vi "MANIPULATOR.vi"() -> ()   [LabVIEW 2018]
uses:
  MCode_LV_86/Set Parameter.ctl
  subVIs/Units_of_Move.ctl
  subVIs/Define_Position.ctl
  subVIs/KE_Scan_XY-Graph.ctl
  Keithley Picoammeter/subVIs/Current_Range_Control.ctl
  subVIs/Scan Mode.ctl
  Surveillance/limit_switch_Cluster.ctl
  ConversionAndInformation/Unit_Control.ctl
  <vilib>/DAQmx/read.llb/DAQmx Read (Analog 1D DBL 1Chan NSamp).vi
  subVIs/Save_Time_Global.vi
  Surveillance/Pressure_Ch_1_2_Manipulator_Pos.vi
  <vilib>/DAQmx/create/channels.llb/DAQmx Create Channel (AI-Voltage-Basic).vi
  <vilib>/DAQmx/configure/timing.llb/DAQmx Timing (Sample Clock).vi
  <vilib>/DAQmx/miscellaneous.llb/DAQmx Fill In Error Info.vi
  subVIs/Global_Next_Scan_Position.vi
  subVIs/Global_external_move_cmd.vi
  Surveillance/Switch _Laser_Global.vi
  <vilib>/Utility/file.llb/Write To Spreadsheet File (DBL).vi
  subVIs/Global_Stop_Scan.vi
panel:
  out "Current Scan Step":i32
  out "Number of Scan Steps":i32
  in  "Next Scan Step":bool
  out "Sample Scan Array Out":i32[][](array[numeric])
  in  "Last Scan Step?":bool
  out "velocity cluster":T1
  out "limit switch cluster":T2
  out "Motor 6":u16
  out "At Next Pos?":bool caption="At Next Position?"
  out "At first Scan Pos?":bool
  out "waypoint info pic":picture
  in  "Disp Axis Info":bool
  out "axis info pic":picture
  in  "Current\nRange Ch2":T3 items=["Autorange", "+/- 20 mikroA", "+/- 2 mikroA", "+/- 200 nA", "+/- 20 nA", "+/- 2 nA"]
  in  "Current\nRange Ch1":T3 items=["Autorange", "+/- 20 mikroA", "+/- 2 mikroA", "+/- 200 nA", "+/- 20 nA", "+/- 2 nA"]
  in  "GPIB (t) / RS-232 (f)":bool=TRUE
  in  "DAQ Dev":refnum<visa-resource-name>="GPIB0::25::INSTR"
  out "Status":i32 format="%.0b"
  out "use data":bool
  out "buffer":string
  in  "Cluster":T4={"Baudrate (57600)"=57600, "Data Bits (8)"=8, "Parity (None)"=0, "Stop Bits (1)"=10, "Flow Control (None)"=0, "End Mode Read (TermChar)"=2} {"End Mode Read (TermChar)" items=["None", "Last Bit", "TermChar"]; "Flow Control (None)" items=["None", "XON/XOFF", "RTS/CTS", "XON/XOFF & RTS/CTS", "DTR/DSR", "XON/XOFF & DTR/DSR"]; "Stop Bits (1)" items=["1.0"=10, "1.5"=15, "2.0"=20]; "Parity (None)" items=["None", "Odd", "Even", "Mark", "Space"]; "Baudrate (57600)" items=["300"=300, "600"=600, "1200"=1200, "2400"=2400, "4800"=4800, "9600"=9600, "19200"=19200, "38400"=38400, "57600"=57600, "115200"=115200]}
  in  "Notizen":string="Limit switch rotation at +225 degrees\n                                          -135 degrees\nSample 1\nSample 2\nSample 3\nSample 4 rutile single crystal (left edge, middle)"
  out "Loaded Positions":string
  in  "Load Motor Positions":bool
  in  "Define New\nPos Dummy":bool
  in  "Set x,y,z Zero Dummy":bool
  in  "Set Angle Zero Dummy":bool
  in  "Stop w Save Pos":bool
  out "MM?":bool
  in  "emergency stop":bool
  in  "stop":bool
  in  "Tab Control":T5(tab)
  in  "ComPort Manipulator":refnum<visa-resource-name>="COM5"
  out "error out":errorcluster={"status"=FALSE, "code"=1073676294, "source"="VISA Read in write_read.vi"}
  out "ComPort out":refnum<visa-resource-name>
  in  "Answer":string
  in  "Send Cmd":bool
  in  "Value":string
  in  "Reset Error":bool
  in  "Command":T6
  in  "Send Cmd as is":bool
  in  "Send As Is String":string
  in  "Motor":u16(ring) items=["none", "1", "2", "3", "4", "all"]
  in  "Print":bool
  in  "Print Error":bool
  out "Transmitted String":string
  in  "Clear Answer":bool
  out "Firmware Version":string
  out "Stop Scan GLOBAL":bool
  out "scan info pic":picture
  in  "ext. Cmd":bool
  out "Scan\nProb?":bool
  in  "POV Map":bool
  out "Next Pos":i32[](array[numeric])
  in  "Disp Path":bool=TRUE
  in  "refresh (s)":dbl=2.0
  in  "Reset Map":bool
  out "Pos Graph":cluster{dbl[], dbl[]}[](graph)
  out "Paused?":bool
  in  "Disp Waypoint Info":bool
  out "Pico Error":bool
  in  "Z tilt (x/z)":dbl=0.00339817
  in  "pause scan":bool
  in  "Scan Type":bool
  in  "Scan Mode":T7 caption="Scan Settings" items=["Mode 1", "Mode 2", "Reversed 1", "Reversed 2"]
  in  "Disp Scan Info":bool
  in  "Stop Scan (2D)":bool
  in  "Speed [microns/s]":dbl=100.0 min=0.0 max=1500.0
  in  "Sample\nScan":bool
  in  "Channel IN":tag
  out "Mean":dbl caption="Analog IN (V)" format="%_3e"
  in  "V_min":dbl=-10.0
  in  "V_max":dbl=10.0
  in  "Stop NI":bool
  in  "Start NI":bool
  out "Display Saved Pos String":string
  in  "Display Saved Position":bool
  in  "WAYPOINTS":u16(ring) items=["Current Position", "Diode Bottom", "Diode Middle Small", "Diode Middle Large", "Diode Top", "Phosphor", "Sample 1", "Sample 2", "Sample 3", "Sample 4", "Horizontal Motor Scan", "Vertical Motor Scan", "Corner Left Top", "Corner Bottom Right"]
  in  "Go to Saved Position":bool
  in  "Motor 4":dbl
  in  "Motor 3":dbl
  in  "Motor 2":dbl
  in  "Motor 1":dbl
  in  "Def Speed":bool
  in  "Unit of Move":T8=1 items=["STEPS", "MICRONS / DEG", "MILLIMETER / DEG", "CENTIMETER / DEG", "INCHES / DEG"]
  in  "move in plain 2":bool caption="M1 + / M2 -"
  in  "move in plain 1":bool caption="M1 - / M2 +"
  in  "move away detector":bool caption="M1 +"
  in  "move to detector":bool caption="M1 -"
  in  "move clockwise":bool caption="M4 -"
  in  "move counterclockwise":bool caption="M4 +"
  in  "move away x-rays":bool caption="M2 +"
  in  "move to x-rays":bool caption="M2 -"
  out "Saved Positions":string
  in  "Save Motor Positions":bool
  in  "Set Angle Zero":bool
  in  "Set x,y,z Zero":bool
  in  "move down":bool caption="M3 +"
  in  "move up":bool caption="M3 -"
  in  "Rel Steps":string="1"
  in  "Speed":dbl=250.0 caption="(microns/s)/\n(degrees/s)" min=0.0 max=2000.0
  in  "Pos 1 (Steps)":i32 caption="Position 1 (Steps)"
  in  "Pos 2 (Steps)":i32 caption="Position 2 (Steps)"
  in  "Pos 3 (Steps)":i32 caption="Position 3 (Steps)"
  in  "Pos 4 (Steps)":i32 caption="Position 4 (Steps)"
  in  "Pos 1":dbl caption="Position 1" step=1.0 format="%_6g"
  in  "Pos 2":dbl caption="Position 2" step=1.0 format="%_6g"
  in  "Pos 3":dbl caption="Position 3" step=1.0 format="%_6g"
  in  "Pos 4 [Angle]":dbl caption="Position 4 [Angle]" step=0.1 format="%_6g"
  in  "Get Motor Positions":bool
  in  "Pos Unit":T8=1 items=["STEPS", "MICRONS / DEG", "MILLIMETER / DEG", "CENTIMETER / DEG", "INCHES / DEG"]
  in  "Z tilt (degrees)":dbl=-0.1947 caption="(degrees)"
  in  "Z tilt comp":bool
  in  "Motor2-xRays (degrees)":dbl
  in  "Unit of Move 3":T8=1 items=["STEPS", "MICRONS / DEG", "MILLIMETER / DEG", "CENTIMETER / DEG", "INCHES / DEG"]
  in  "M1 Change":T9
  in  "M2 Change":T9
  in  "M3 Change":T9
  in  "M4 Change":T9
  in  "Define New Pos":bool caption="DEFINE CURRENT POSITION"
  out "Data":dbl[](array[numeric]) caption="Channel 1 (A)\n\nChannel 2 (A)" format="%#_3e"
  in  "Stop K":bool
  in  "Calc Scan Time":bool
  out "Scan Time":string
  in  "Start K":bool
  in  "Line Spacing [microns]":dbl=500.0
  in  "Pico Steps":i32 caption="Steps"
  in  "PicoMotor":u16(ring) caption="Motor" items=["A", "B", "C"]
  in  "Move Pico":bool
  in  "Picomotors Port":refnum<visa-resource-name>="COM1"
  in  "GaussFit der (f, def) / raw (t)":bool caption="GaussFit\nder (f)\nraw (t)"
  in  "div I zero":bool=TRUE caption="divide by other K Ch"
  in  "Interrupt 2":bool
  in  "Interrupt 1":bool
  in  "Go to Cursor (1 Motor)":bool
  in  "Knife Edge Scan\n(1 Motor)":bool
  in  "Scan Range":dbl=100.0
  in  "Axis":u16(ring) items=["Detector", "X-Rays", "Vertical", "In-Plain", "Vertical (with tilt)"]
  in  "Nr. of Steps":u32=10
  in  "Integration Time per Step":u32=1500
  in  "Channel":i32=1 min=0 max=7 step=1
  in  "Go to Cursor (2 Motors)":bool
  in  "Knife Edge Scan\n(2 Motors)":bool
  out "XY Graph":T10
  out "FWHM":dbl format="%.1f"
  out "Center":dbl format="%.1f"
  out "Resolution":dbl
  out "Start\nTime":timestamp
  out "Estimated\nStop Time":timestamp
  out "Scan Number":i32
  out "Residue":dbl
  in  "NI DAQ (t) / Keithley (f)":bool
  out "current time":string
  out "end time":string
  in  "Switch Laser":bool
  in  "XPS Scan Speed [µm/s]":dbl=100.0 caption="Scan Speed [µm/s]" min=0.0 max=1500.0
  in  "Z tilt comp XPS":bool
  in  "Z tilt (M2/M3) XPS":dbl=0.00202
  in  "scan up M3- XPS":bool
  in  "scan down M3+ XPS":bool
  in  "Scan Distance XPS":string="5" caption="Scan Distance (mm)"
  in  "stop scan XPS":bool
  in  "scan left XPS":bool
  in  "scan right XPS":bool
  in  "Hor Angle Offset (degrees)":dbl
  in  "Hor Angle Offset (rad) M2/M1":dbl
  out "M4 XPS":dbl caption="M4 Angle (degrees)" step=10.0 format="%_6g"
  out "M3 XPS":dbl caption="M3 Vertical (micrometer)" step=1.0 format="%_6g"
  out "M2 XPS":dbl caption="M2 Analyzer (micrometer)" step=1.0 format="%_6g"
  out "M1 XPS":dbl caption="M1 X-rays (micrometer)" step=1.0 format="%_6g"
  in  "Rel Steps XPS":string="1000" caption="Micrometer µm"
  in  "approach XPS":bool caption="M 2 - / M 1 -"
  in  "retract XPS":bool caption="M 2 + / M 1 +"
  in  "in plain 2 XPS":bool caption="M 2 - / M 1 +"
  in  "in plain 1 XPS":bool caption="M 2 + / M 1 -"
  in  "away X-rays M1+ XPS":bool caption="M 1 +"
  in  "to X-rays M1- XPS":bool caption="M 1 -"
  in  "move clockwise XPS":bool caption="M 4 -"
  in  "move counterclockwise XPS":bool caption="M 4 +"
  in  "away analyzer M2+ XPS":bool caption="M 2 +"
  in  "to analyzer M2- XPS":bool caption="M 2 -"
  in  "down M3+ XPS":bool caption="M 3 +"
  in  "up M3- XPS":bool caption="M 3 -"
  in  "Rel Deg XPS":string="1" caption="Degrees"
  out "Pos Graph 2":cluster{dbl[], dbl[]}[](graph)
  in  "down M3+ TEST":bool
  in  "up M3- TEST":bool
  out "actual angle":dbl format="%_6g"
  out "V_max Motor 2":i32
  out "V_max Motor 1":i32
  out "steps motor 2 ()":string
  out "steps motor 1 ()":string
  in  "Idiotensicherung":bool
  out "delta time (ms)":i32
  in  "steps 2":i32
  in  "Loop Stop":bool
  in  "Motor 5":u16(ring) items=["none", "1", "2", "3", "4", "all"]
  in  "Move Time Test":bool
  in  "motor stopped":bool
  out "1":u32
  out "2":u32
  out "single steps 1":i32[](array[numeric])
  out "single steps 2":i32[](array[numeric])
  out "move time (ms)":u32
  out "single steps":i32[](array[numeric])
  out "New X-Ray Pos":i32
  out "Percentage Range Micron Pos":dbl
  out "Range X-Rays":i32
  out "Range M1/M3":i32
  out "Min Value X-Rays":i32
  in  "direction":bool
  in  "In-Plain subVI Test":bool
  in  "Speed [micron/s] 2":dbl=750.0 min=0.0
  in  "Steps":dbl format="%#_13g"
  in  "Unit of Move 2":T8 items=["STEPS", "MICRONS / DEG", "CENTIMETER / DEG", "INCHES / DEG"]
  out "move time (ms) 4":u32
  out "actual angle 2":dbl format="%_6g"
  out "angle":dbl
  out "Array Lengths equal?":bool
  out "V_max 1/3 and 2":i32[](array[numeric])
  out "micron steps":dbl[](array[numeric])
  out "New M1/M3 Pos":i32
  out "KE Scan Array":dbl[][](array[numeric])
  out "Transmitted 1/3":string
  out "Transmitted 2":string
  in  "Save latest KE Scan":bool
  out "error Keithley":errorcluster
  out "error NI":errorcluster
  out "corner 1":dbl[](array[numeric])
  out "corner 2":dbl[](array[numeric])
  in  "Reset V_max":bool
  in  "Save Files Array":path[](array[path])
  out "KE Positions":dbl[](array[numeric]) caption="(micron/degree)"
  out "Transmitted String Baud Rate":string
  in  "Baudrate":u32(ring)=9600 items=["9600"=9600, "19200"=19200, "38400"=38400, "115200"=115200]
  in  "Change Baud Rate":bool
  # "LIMIT\nSWITCH"
  # "KEITHLEY SETTINGS"
  # "angle element -90 to 90 deg:\n[sample holder facing xrays]\nIn plain 1 -> towards detector\nIn plain 2 -> away from det.\nangle <-90 or >90 deg:\n[back of sample holder facing xrays]\nIn plain 1 -> away from det.\nIn plain 2 -> towards detector"
  # "RELATIVE MOVEMENT"
  # "ABSOLUTE MOVEMENT"
  # "motor 1: detector axis [+ away / - towards detector]"
  # "motor 2: x-ray axis [+ away / - towards x-rays]"
  # "motor 3: vertical axis [+ down / - up]"
  # "motor 4: angle [+ counterclockwise / - clockwise]"
  # "TILT COMPENSATION"
  # "WAYPOINTS"
  # "NOT functional"
  # "Sample holder facing x-rays. Alpha is the angle between\nmanipulator z-axis and x-rays incident on the sample holder.\n\"Z tilt\" is > 0 if alpha >90 degreees (\"Z tilt\"<0 -> alpha < 90)."
  # "KEITHLEY PICCOAMMETER"
  # "NI USB DAQ BOARD"
  # "SAMPLE SCAN"
  # "NEWFOCUS PICOMOTORS"
  # "DAQ Source"
  # "Range: +/-"
  # "microns around current position"
  # "+1 | Integration time per step:"
  # "Steps: 2x"
  # "ms"
  # "Axis:"
  # "| Sampling:"
  # "microns"
  # "FINE POSITIONING"
  # "SCANNING SAMPLE"
  # "Replace In-Plain\nCode with real\ntrigonometric\nfunctions!"
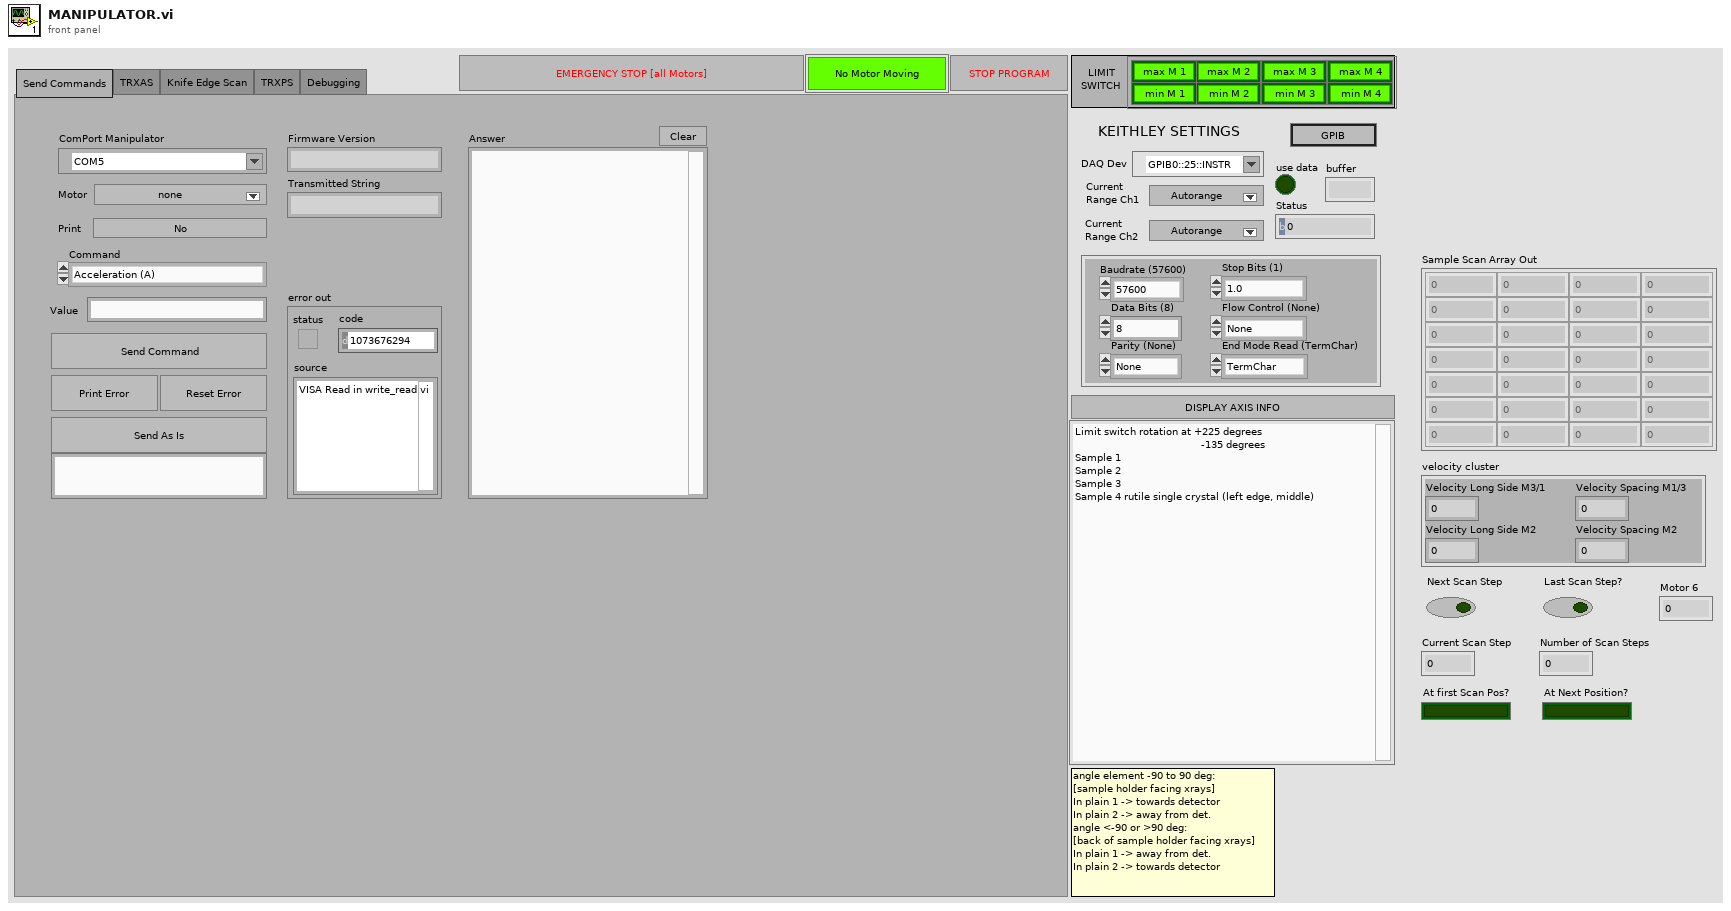
[diagram p1: front panel]
types:
  T1 = cluster{"Velocity Long Side M3/1":dbl, "Velocity Long Side M2":dbl, "Velocity Spacing M1/3":dbl, "Velocity Spacing M2":dbl}
  T2 = typedef "limit_switch_Cluster.ctl" = cluster{"Limit Switch max M 1":bool, "Limit Switch min M 1":bool, "Limit Switch max M 2":bool, "Limit Switch min M 2":bool, "Limit Switch max M 3":bool, "Limit Switch min M 3":bool, "Limit Switch max M 4":bool, "Limit Switch min M 4":bool}
  T3 = typedef "Current_Range_Control.ctl" = u16
  T4 = cluster{"Baudrate (57600)":u32, "Data Bits (8)":u16, "Parity (None)":u16, "Stop Bits (1)":u16, "Flow Control (None)":u16, "End Mode Read (TermChar)":u16}
  T5 = enum32{"Send Commands", "TRXAS", "Knife Edge Scan", "TRXPS", "Debugging"}
  T6 = typedef "Set Parameter.ctl" = enum16{"Acceleration (A)", "Baud Rate (BD)", "Counter 1 (C1)", "Counter 2 (C2)", "Control C Software Reset (CE)", "Check Sum Enable (CK)", "Clock Mode (CM)", "Clock Mode Ratio (CR)", "Clock Mode Out Step Width (CW)", "Deceleration (D)", "Digital Filtering, Input 1 (D1)", "Digital Filtering, Input 2 (D2)", "Digital Filtering, Input 3 (D3)", "Digital Filtering, Input 4 (D4)", "Digital Filtering, Input 5 (D5)", "Digital Filtering, Input 9 (D9)", "Digital Filtering, Input 10 (D10)", "Digital Filtering, Input 11 (D11)", "Digital Filtering, Input 12 (D12)", "Deadband (DB)", "Decrement Variable (DC)", "Enable/Disable Drive (DE)", "Device Name (DN)", "End Program Execution (E)", "Encoder Function Enable (EE)", "Error Flag (EF)", "Encoder Lines (EL)", "Echo Mode (EM)", "Error Value (ER)", "Escape (ES)", "Execute Program at Address (EX)", "Firmware Version (VR)", "Hold (H)", "Hold Current (HC)", "Hold Current Delay Time (HI)", "Home to Encoder Index (HM)", "Home to Home Switch (HT)", "Increment Variable (IC)", "Initialize Parameters to NVM (IP)", "Input into Variable (IV)", "Jog Enable (JE)", "Limit Stop Mode (LM)", "Move Absolute (MA)", "Move Relative (MR)", "MicroStepping Select (MS)", "Motor Settling Delay Time (MT)", "Moving [Flag] (MV)", "Output 1 (O1)", "Output 2 (O2)", "Output 3 (O3)", "Output 4 (O4)", "Output 9 (O9)", "Output 10 (O10)", "Output 11 (O11)", "Output 12 (O12)", "Output High Byte (9-12) (OH)", "Output Low Byte (1-4) (OL)", "Output Total (1-4 and 9-12) (OT)", "Position (P)", "Position Maintenance (PM)", "Party Mode (PY)", "Register 1 (R1)", "Register 2 (R2)", "Register 3 (R3)", "Register 4 (R4)", "Reset Error(\\03)", "Run Current (RC)", "Stall Factor (SF)", "Slew (SL)", "Stall Mode Set (SM)", "Upgrade Firmware (UG)", "Velocity Initial (VI)", "Velocity Maximum (VM)", "Current1 (I1)", "Current2 (I2)", "Current3 (I3)", "Current4 (I4)", "Current5 (I5)", "Current6 (I6)", "Save (S)"}
  T7 = typedef "Scan Mode.ctl" = u16
  T8 = typedef "Units_of_Move.ctl" = u16
  T9 = typedef "Define_Position.ctl" = bool
  T10 = typedef "KE_Scan_XY-Graph.ctl" = cluster{dbl[], "subarray":dbl[]}[]
  T11 = typedef "Unit_Control.ctl" = enum16{"Angle (Degrees)", "Rad", "Angle [TMC]", "Microsteps [TMC]", "Inches", "Nanometer", "Meter", "Centimeter", "Millimeter", "Micron"}
  T12 = cluster{"Baudrate (115200)":u32, "Data Bits (8)":u16, "Parity (None)":u16, "Stop Bits (1)":u16, "Flow Control (None)":u16, "End Mode for Reads (TermChar)":u16}
  T13 = enum16{"open", "replace", "create", "open or create", "replace or create", "replace or create with confirmation"}
  T14 = typedef "imagedata.ctl" = cluster{"image type":i32, "image depth":i32, "image":u8[], "mask":u8[], "colors":u32[], "Rectangle":cluster{"left":i16, "top":i16, "right":i16, "bottom":i16}}
  T15 = typedef "Semaphore RefNum" = refnum<k1>
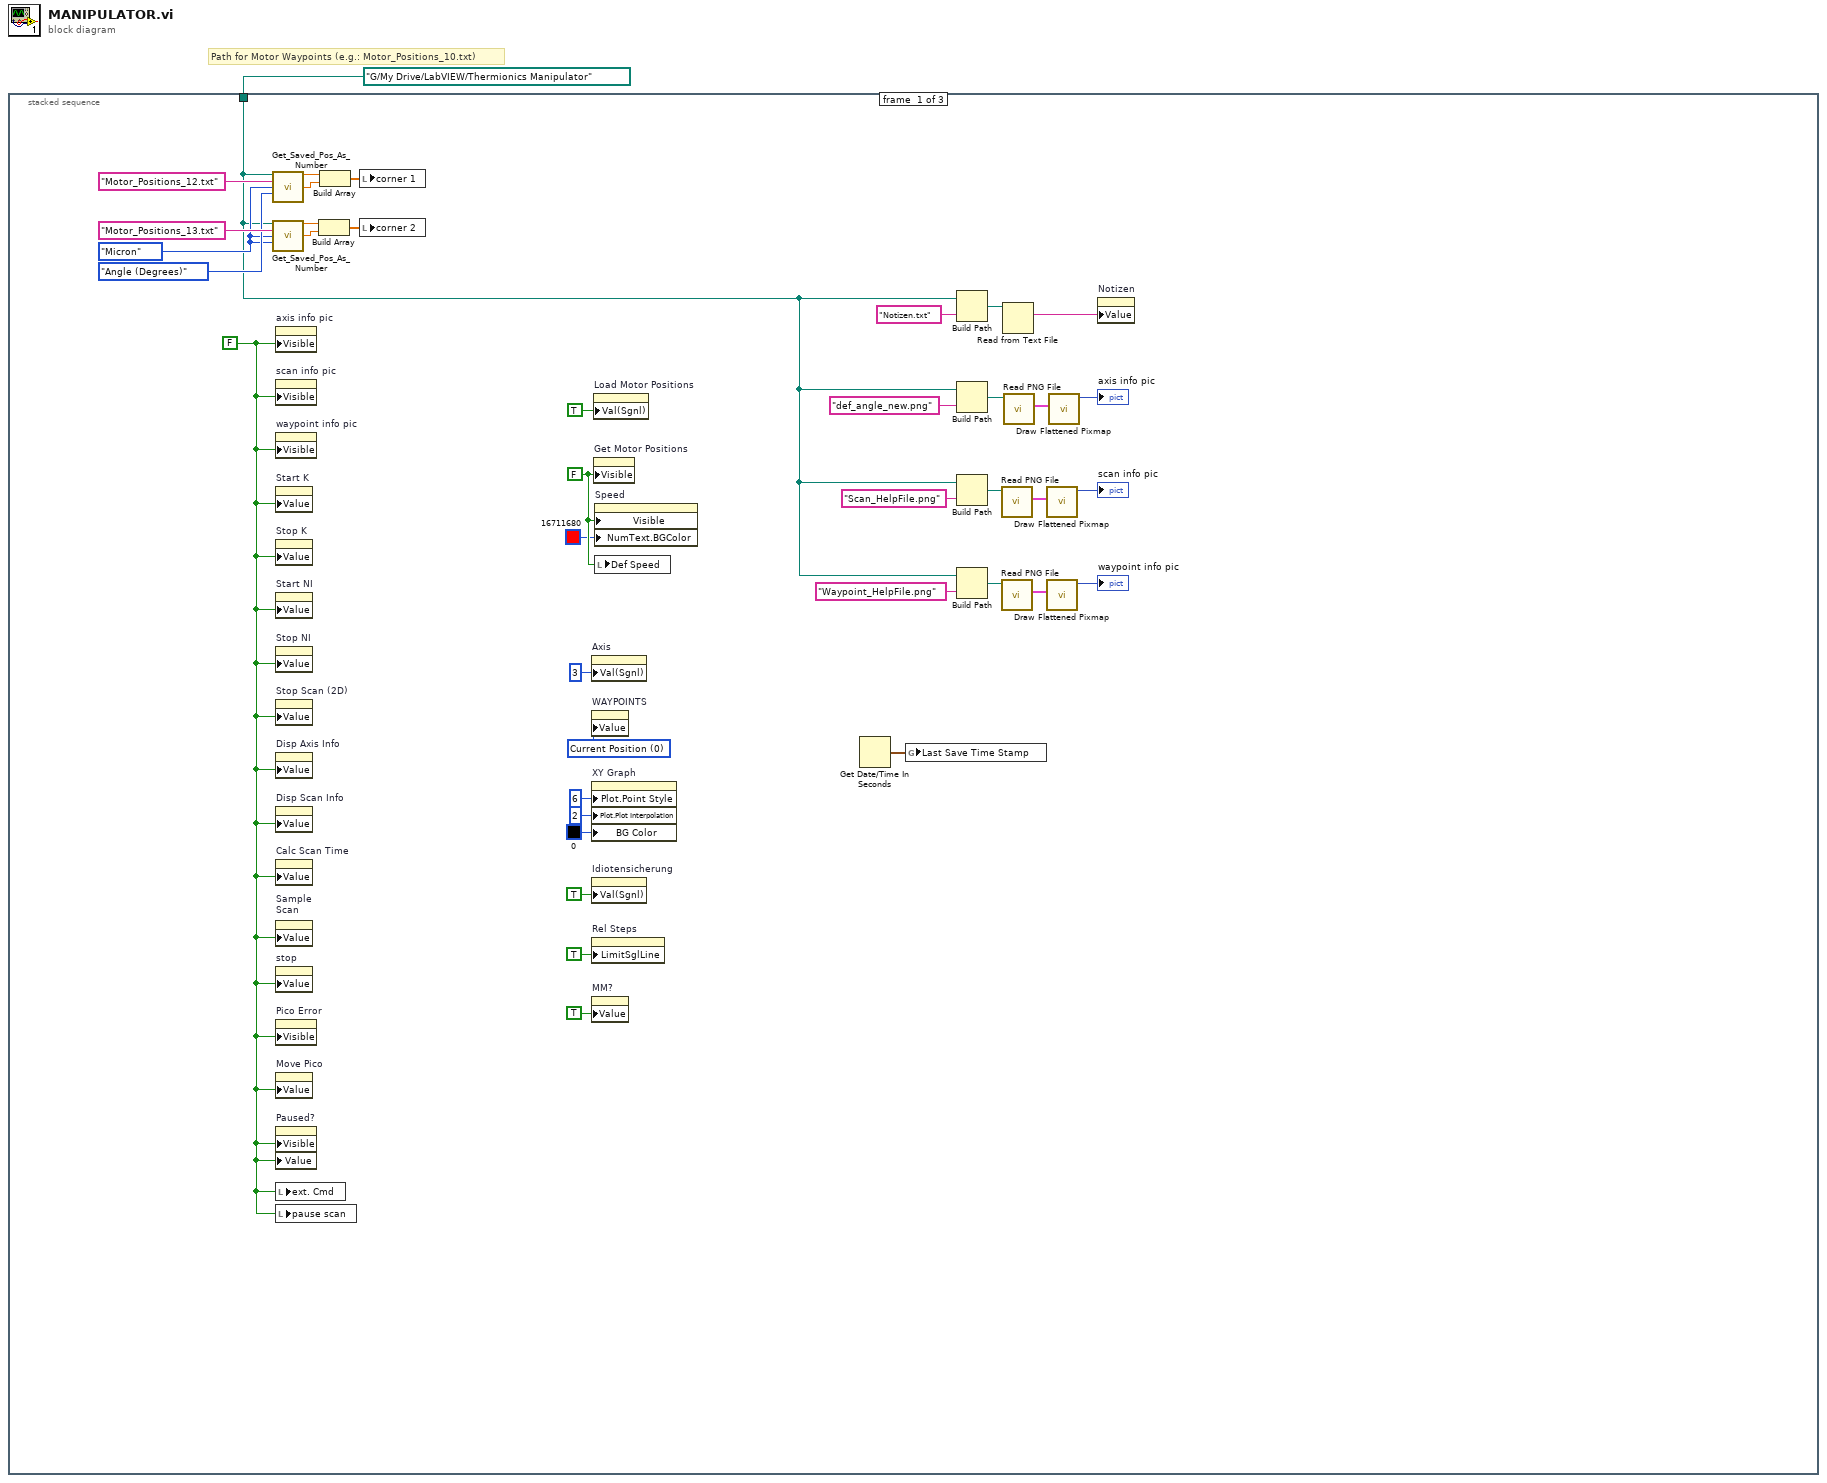
[diagram p0: block diagram]
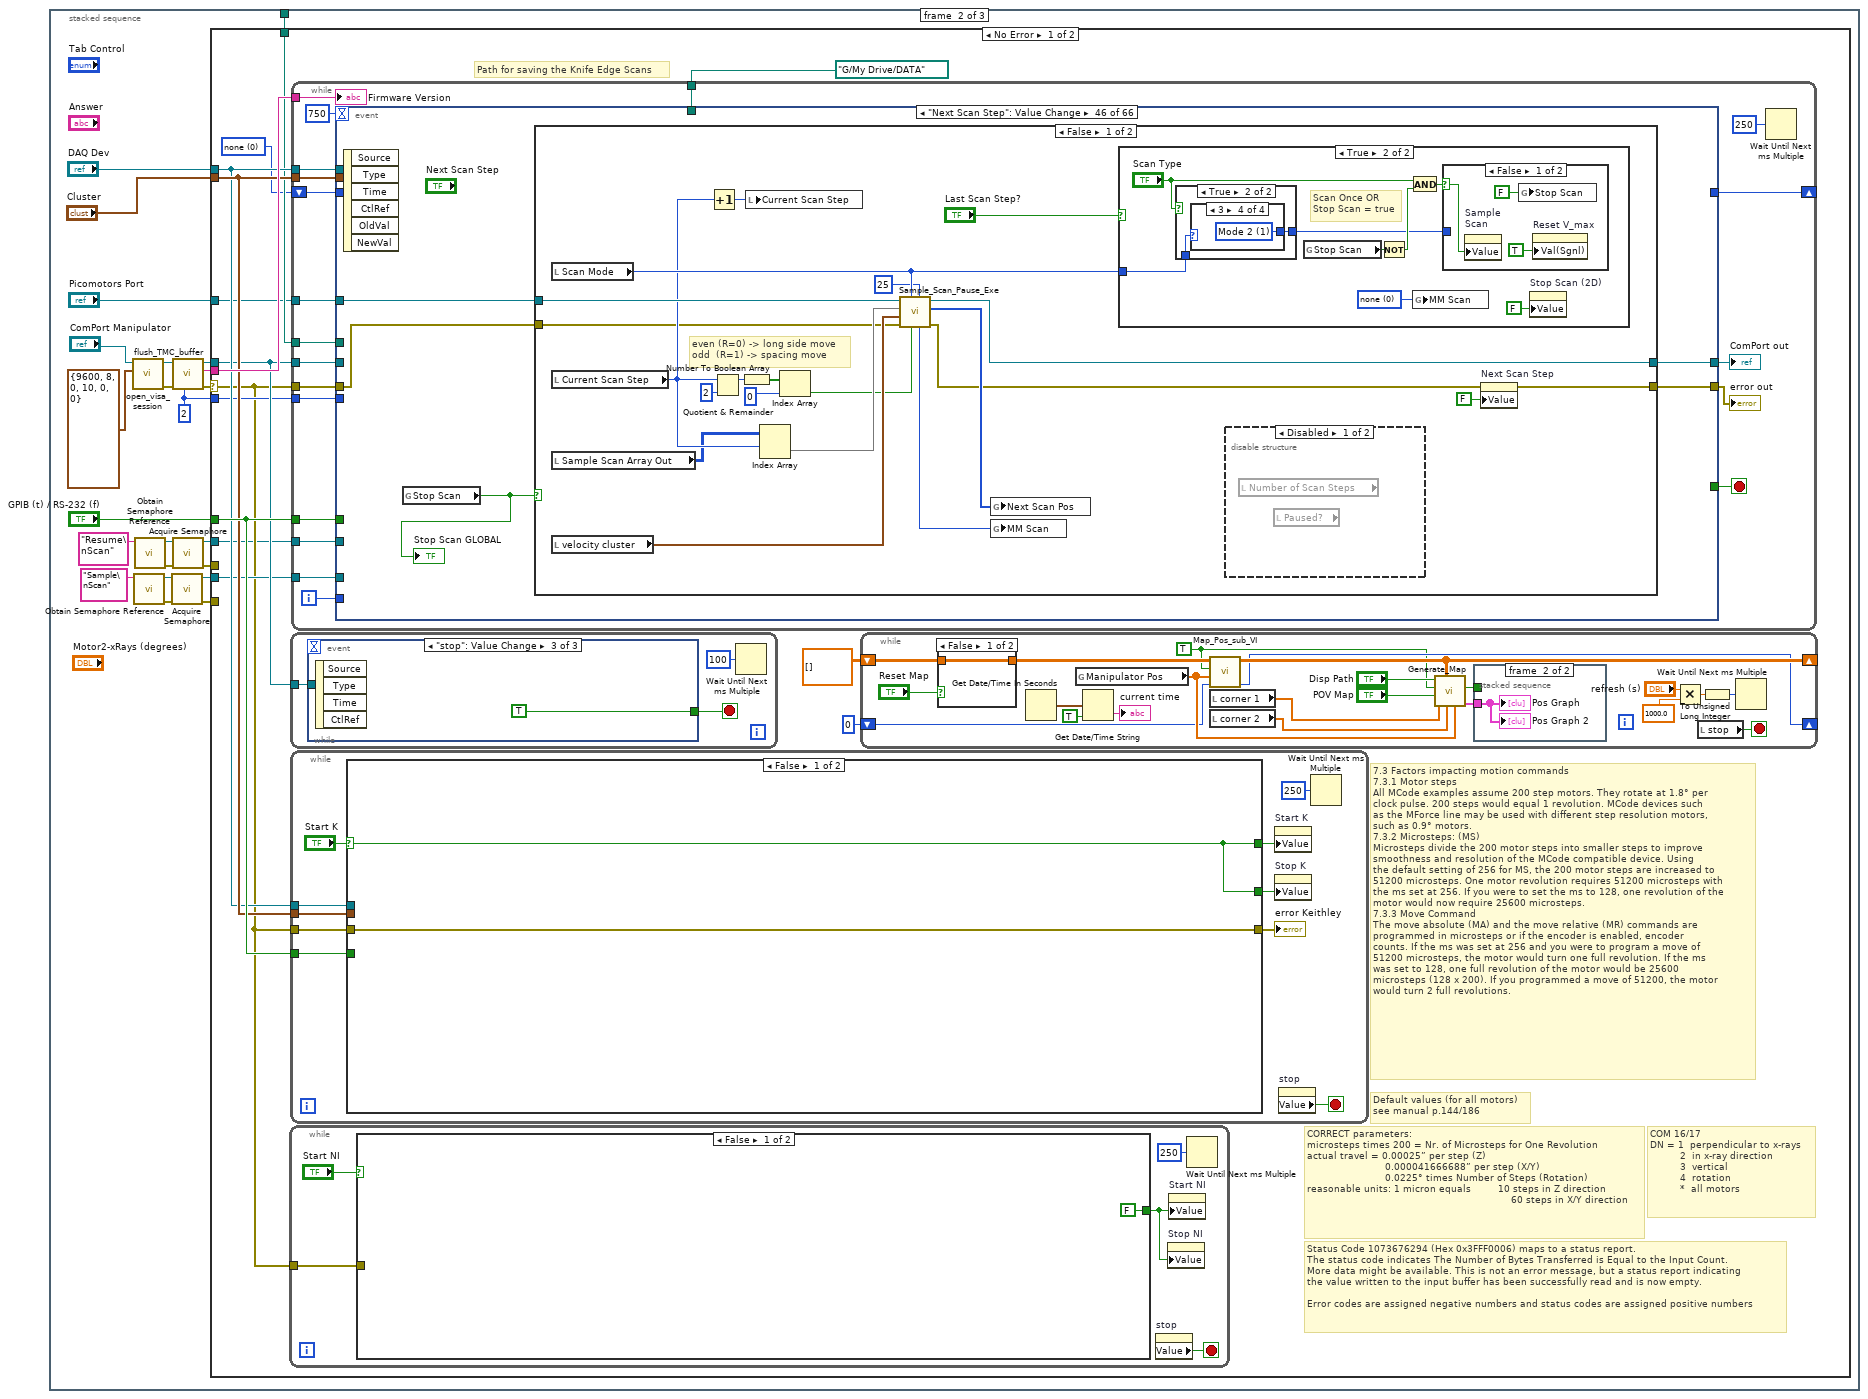
[diagram p2: hidden frame]
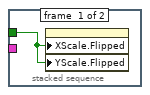
[diagram p3: hidden frame]
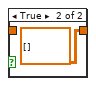
[diagram p4: hidden frame]
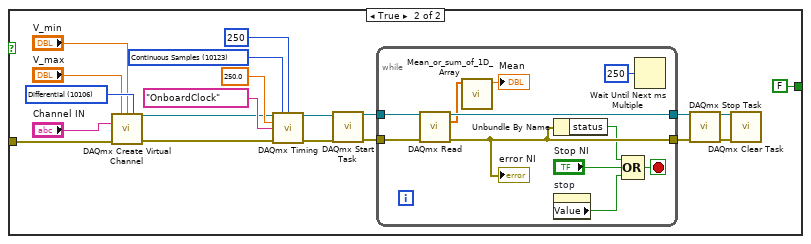
[diagram p5: hidden frame]
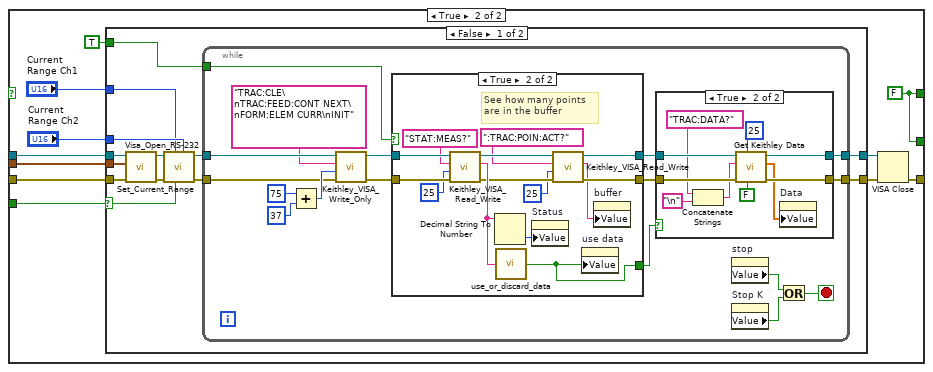
[diagram p6: hidden frame]
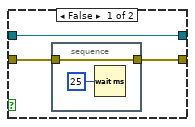
[diagram p7: hidden frame]
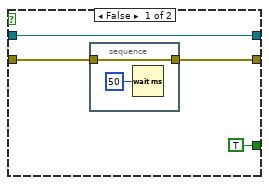
[diagram p8: hidden frame]
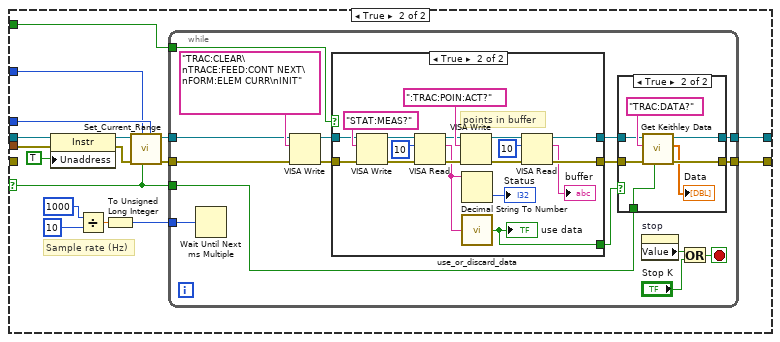
[diagram p9: hidden frame]
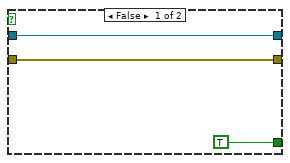
[diagram p11: hidden frame]
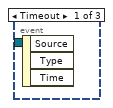
[diagram p12: hidden frame]
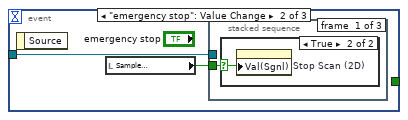
[diagram p13: hidden frame]
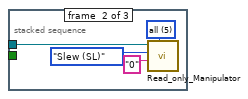
[diagram p15: hidden frame]
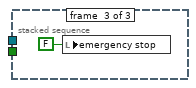
[diagram p16: hidden frame]
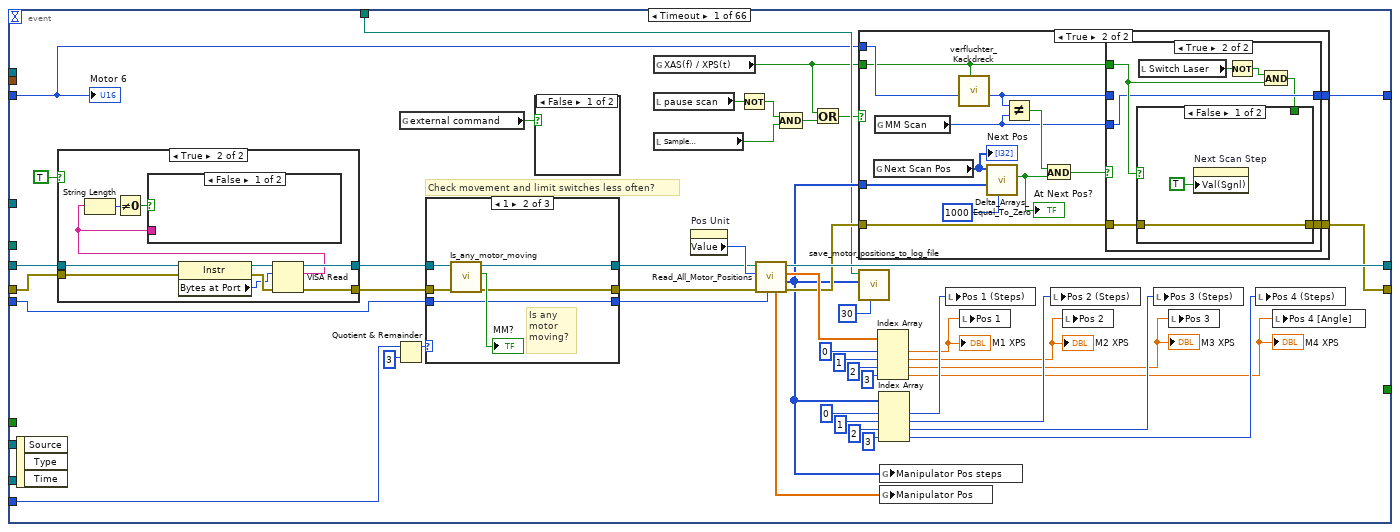
[diagram p17: hidden frame]
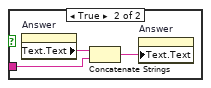
[diagram p19: hidden frame]
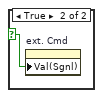
[diagram p20: hidden frame]
diagram:
  # "Path for Motor Waypoints (e.g.: Motor_Positions_10.txt)"
  n1 = stacked-sequence {
    tunnel: path "G:/My Drive/LabVIEW/Thermionics Manipulator" ("file path (use dialog)") -> [w5 w48 _]
    frame #0 {
      w18 = Unit_Control."Micron" ("Outuput Unit 1/2/3")
      w27 = u16 0 items=["Current Position", "Diode Bottom", "Diode Middle Small", "Diode Middle Large", "Diode Top", "Phosphor", "Sample 1", "Sample 2", "Sample 3", "Sample 4"] ("WAYPOINTS")
      w25 = FALSE ("Visible")
      w9 = FALSE ("Visible")
      n2 = call "Get_Saved_Pos_As_Number.vi"("file path"=w5, "file name"="Motor_Positions_12.txt" ("name or relative path"), "Outuput Unit 1/2/3"=w18, "Outuput Unit 4"=Unit_Control."Angle (Degrees)" ("Outuput Unit 1/2/3")) -> ("Pos 1"=w17:dbl, "Pos 3"=w16:dbl)  [unwired: 7 in, 3 out]
      n3 = call "Get_Saved_Pos_As_Number.vi"("file path"=w5, "file name"="Motor_Positions_13.txt" ("name or relative path"), "Outuput Unit 1/2/3"=w18, "Outuput Unit 4"=w18) -> ("Pos 1"=w15:dbl, "Pos 3"=w14:dbl)  [unwired: 7 in, 3 out]
      n4 = property on="axis info pic" class="Pict"("Visible"=w9) -> ()  [unwired: 2 in, 2 out]
      n5 = property on="scan info pic" class="Pict"("Visible"=w9) -> ()  [unwired: 2 in, 2 out]
      n6 = property on="waypoint info pic" class="Pict"("Visible"=w9) -> ()  [unwired: 2 in, 2 out]
      n7 = property on="Start K" class="Bool (strict)"("Value"=w9) -> ()  [unwired: 2 in, 2 out]
      n8 = property on="Stop K" class="Bool (strict)"("Value"=w9) -> ()  [unwired: 2 in, 2 out]
      n9 = property on="Start NI" class="Bool (strict)"("Value"=w9) -> ()  [unwired: 2 in, 2 out]
      n10 = property on="Stop NI" class="Bool (strict)"("Value"=w9) -> ()  [unwired: 2 in, 2 out]
      n11 = property on="Stop Scan (2D)" class="Bool (strict)"("Value"=w9) -> ()  [unwired: 2 in, 2 out]
      n12 = property on="Disp Axis Info" class="Bool (strict)"("Value"=w9) -> ()  [unwired: 2 in, 2 out]
      n13 = property on="Disp Scan Info" class="Bool (strict)"("Value"=w9) -> ()  [unwired: 2 in, 2 out]
      n14 = property on="Calc Scan Time" class="Bool (strict)"("Value"=w9) -> ()  [unwired: 2 in, 2 out]
      n15 = property on="Sample\nScan" class="Bool (strict)"("Value"=w9) -> ()  [unwired: 2 in, 2 out]
      n16 = property on="stop" class="Bool (strict)"("Value"=w9) -> ()  [unwired: 2 in, 2 out]
      n17 = property on="Pico Error" class="Bool (strict)"("Visible"=w9) -> ()  [unwired: 2 in, 2 out]
      n18 = property on="Move Pico" class="Bool (strict)"("Value"=w9) -> ()  [unwired: 2 in, 2 out]
      n19 = property on="Paused?" class="Bool (strict)"("Visible"=w9, "Value"=w9) -> ()  [unwired: 2 in, 2 out]
      n20 = local write "ext. Cmd"(w9) -> ()
      n21 = local write "pause scan"(w9) -> ()
      n22 = Build Array(w15, w14) -> (w22:dbl[])
      n23 = Build Array(w17, w16) -> (w23:dbl[])
      n24 = local write "corner 1"(w23) -> ()
      n25 = local write "corner 2"(w22) -> ()
      n26 = property on="Axis" class="Ring (strict)"("Val(Sgnl)"=u16 3 ("Value (Signaling)")) -> ()  [unwired: 2 in, 2 out]
      n27 = property on="WAYPOINTS" class="Ring (strict)"("Value"=w27) -> ()  [unwired: 2 in, 2 out]
      n28 = property on="XY Graph" class="XYGraph (strict)"("Plot.Point Style"=u8 6, "Plot.Plot Interpolation"=u8 2, "BG Color"=u32 0) -> ()  [unwired: 2 in, 2 out]
      n29 = property on="Idiotensicherung" class="Bool (strict)"("Val(Sgnl)"=TRUE ("Idiotensicherung")) -> ()  [unwired: 2 in, 2 out]
      n30 = property on="Rel Steps" class="Str"("LimitSglLine"=TRUE ("Limit To Single Line?")) -> ()  [unwired: 2 in, 2 out]
      n31 = property on="MM?" class="Bool (strict)"("Value"=TRUE) -> ()  [unwired: 2 in, 2 out]
      n32 = property on="Load Motor Positions" class="Bool (strict)"("Val(Sgnl)"=TRUE ("Value (Signaling)")) -> ()  [unwired: 2 in, 2 out]
      n33 = property on="Get Motor Positions" class="Bool (strict)"("Visible"=w25) -> ()  [unwired: 2 in, 2 out]
      n34 = property on="Speed" class="DigNum (strict)"("Visible"=w25, "NumText.BGColor"=u32 16711680) -> ()  [unwired: 2 in, 2 out]
      n35 = local write "Def Speed"(w25) -> ()
      n36 = Get Date/Time In Seconds() -> (seconds since 1Jan1904=w10:timestamp)
      n37 = global write "Save_Time_Global.vi" "Last Save Time Stamp"(w10) -> ()
      n38 = Build Path(base path=w5, name or relative path="Notizen.txt") -> (appended path=w38:path)
      n39 = Build Path(base path=w5, name or relative path="def_angle_new.png") -> (appended path=w4:path)
      n40 = Build Path(base path=w5, name or relative path="Scan_HelpFile.png") -> (appended path=w3:path)
      n41 = Build Path(base path=w5, name or relative path="Waypoint_HelpFile.png") -> (appended path=w2:path)
      n42 = call <vilib>:"Read PNG File.vi"("path to PNG file"=w3) -> ("image data"=w33:T14)  [unwired: 8 in, 2 out]
      n43 = call <vilib>:"Read PNG File.vi"("path to PNG file"=w2) -> ("image data"=w13:T14)  [unwired: 8 in, 2 out]
      n44 = Read from Text File(file (use dialog)=w38) -> (text=w39:string)  [unwired: 3 in, 3 out]
      n45 = call <vilib>:"Read PNG File.vi"("path to PNG file"=w4) -> ("image data"=w36:T14)  [unwired: 8 in, 2 out]
      n46 = call <vilib>:"Draw Flattened Pixmap.vi"("image data"=w33) -> ("new picture"=→"scan info pic":picture)  [unwired: 8 in]
      n47 = call <vilib>:"Draw Flattened Pixmap.vi"("image data"=w13) -> ("new picture"=→"waypoint info pic":picture)  [unwired: 8 in]
      n48 = call <vilib>:"Draw Flattened Pixmap.vi"("image data"=w36) -> ("new picture"=→"axis info pic":picture)  [unwired: 8 in]
      n49 = property on="Notizen" class="Str"("Value"=w39) -> ()  [unwired: 2 in, 2 out]
    }
    frame #1 {
      w58 = 2 ("Echo Mode")
      n50 = call "open_visa_session.vi"("Cluster"=T12 {"Baudrate (115200)"=9600, "Data Bits (8)"=8, "Parity (None)"=0, "Stop Bits (1)"=10, "Flow Control (None)"=0, "End Mode for Reads (TermChar)"=0}, "ComPort"="ComPort Manipulator") -> ("error out"=w61:errorcluster, "VISA resource name out"=w62:refnum<visa-resource-name>)  [unwired: 8 in]
      n51 = call <vilib>:"Obtain Semaphore Reference.vi"("name (unnamed)"="Sample\nScan") -> ("error out"=w52:errorcluster, "semaphore"=w53:T15)  [unwired: 4 in, 1 out]
      n52 = call <vilib>:"Obtain Semaphore Reference.vi"("name (unnamed)"="Resume\nScan") -> ("error out"=w47:errorcluster, "semaphore"=w45:T15)  [unwired: 4 in, 1 out]
      n53 = call <vilib>:"Acquire Semaphore.vi"("error in (no error)"=w52, "semaphore"=w53) -> ("error out"=w50:errorcluster, "semaphore out"=w49:T15)  [unwired: 3 in, 1 out]
      n54 = call "flush_TMC_buffer.vi"("Echo Mode"=w58, "error in"=w61, "ComPort"=w62) -> ("error out"=w56:errorcluster, "Firmware Version"=w60:string, "VISA ressource out"=w59:refnum<visa-resource-name>)  [unwired: 6 in]
      n55 = call <vilib>:"Acquire Semaphore.vi"("error in (no error)"=w47, "semaphore"=w45) -> ("error out"=w44:errorcluster, "semaphore out"=w43:T15)  [unwired: 3 in, 1 out]
      n56 = case shown="No Error" w56 {
        selector: w56 -> [w70 _]
        tunnel: w60 -> [w78 _]
        tunnel: w59 -> [w73 _]
        tunnel: w58 -> [w72 _]
        tunnel: "DAQ Dev" -> [w74 _]
        tunnel: "GPIB (t) / RS-232 (f)" -> [w76 _]
        tunnel: "Cluster" -> [w75 _]
        tunnel: w50 -> [_ _]
        tunnel: w49 -> [w71 _]
        tunnel: w48 -> [w68 _]
        tunnel: w44 -> [_ _]
        tunnel: w43 -> [w67 _]
        tunnel: "Picomotors Port" -> [w66 _]
        frame No Error {
          w64 = u16 0 items=["none", "1", "2", "3", "4", "all"] ("Motor 6")
          # "Status Code 1073676294 (Hex 0x3FFF0006) maps to a status report.\nThe status code indicates The Number of Bytes Transferred is Equal to the Input Count.\nMore data might be available. This is not an error message, but a status report indicating\nthe value written to the input buffer has been successfully read and is now empty.\n\nError codes are assigned negative numbers and status codes are assigned positive numbers"
          # "COM 16/17\nDN = 1  perpendicular to x-rays\n          2  in x-ray direction\n          3  vertical\n          4  rotation\n          *  all motors"
          # "CORRECT parameters:\nmicrosteps times 200 = Nr. of Microsteps for One Revolution\nactual travel = 0.00025” per step (Z)\n                          0.000041666688” per step (X/Y)\n                          0.0225° times Number of Steps (Rotation)\nreasonable units: 1 micron equals         10 steps in Z direction\n                                                                    60 steps in X/Y direction"
          # "Path for saving the Knife Edge Scans"
          # "7.3 Factors impacting motion commands\n7.3.1 Motor steps\nAll MCode examples assume 200 step motors. They rotate at 1.8° per\nclock pulse. 200 steps would equal 1 revolution. MCode devices such\nas the MForce line may be used with different step resolution motors,\nsuch as 0.9° motors.\n7.3.2 Microsteps: (MS)\nMicrosteps divide the 200 motor steps into smaller steps to improve\nsmoothness and resolution of the MCode compatible device. Using\nthe default setting of 256 for MS, the 200 motor steps are increased to\n51200 microsteps. One motor revolution requires 51200 microsteps with\nthe ms set at 256. If you were to set the ms to 128, one revolution of the\nmotor would now require 25600 microsteps.\n7.3.3 Move Command\nThe move absolute (MA) and the move relative (MR) commands are\nprogrammed in microsteps or if the encoder is enabled, encoder\ncounts. If the ms was set at 256 and you were to program a move of\n51200 microsteps, the motor would turn one full revolution. If the ms\nwas set to 128, one full revolution of the motor would be 25600\nmicrosteps (128 x 200). If you programmed a move of 51200, the motor\nwould turn 2 full revolutions."
          # "Default values (for all motors)\nsee manual p.144/186"
          n57 = while {
            tunnel: w70 -> [w106]
            stop <- w109 stop-if-true
            n58 = case shown="False" "Start NI" {
              tunnel: w106 -> [_ w113]
              tunnel: [FALSE FALSE] -> w105
              frame False {
              }
              frame True {
                w121 = 10106 items=["default"=-1, "RSE"=10083, "NRSE"=10078, "Differential"=10106, "Pseudodifferential"=12529] ("Terminal Configuration")
                w116 = 10123 items=["Finite Samples"=10178, "Continuous Samples"=10123, "Hardware Timed Single Point"=12522] ("Sample Mode")
                n59 = call-poly <vilib>:"DAQmx Create Virtual Channel.vi"("maximum value"="V_max", "minimum value"="V_min", "input terminal configuration"=w121, "physical channels"="Channel IN", "error in"=w113) -> ("task out"=w118:refnum<k21>, "error out"=w117:errorcluster)  [unwired: 9 in]
                n60 = call-poly <vilib>:"DAQmx Timing.vi"("task/channels in"=w118, "sample mode"=w116, "samples per channel"=250 ("Number of Samples"), "rate"=250.0 ("Sample Rate"), "source"=tag "OnboardClock" ("Sample Clock Source"), "error in"=w117) -> ("task out"=w129:refnum<k21>, "error out"=w128:errorcluster)  [unwired: 8 in]
                n61 = call <vilib>:"DAQmx Start Task.vi"("task/channels in"=w129, "error in"=w128) -> ("task out"=w119:refnum<k21>, "error out"=w120:errorcluster)  [unwired: 12 in]
                n62 = while {
                  tunnel: w119 -> [w141]
                  tunnel: w120 -> [w135]
                  tunnel: [w140] -> w124
                  tunnel: [w139] -> w125
                  stop <- w137 stop-if-true
                  n63 = call-poly <vilib>:"DAQmx Read.vi"("task/channels in"=w141, "error in"=w135) -> ("task out"=w140:refnum<k21>, "data"=w132:dbl[], "error out"=w139:errorcluster)  [unwired: 11 in]
                  "error NI" <- w139
                  n64 = call "Mean_or_sum_of_1D_Array.vi"("Array"=w132) -> ("Sum/Mean"=→"Mean":dbl)  [unwired: 10 in]
                  n65 = Unbundle By Name(w139) -> ("status"=w138:bool)
                  n66 = property on="stop" class="Bool (strict)"() -> ("Value"=w134:bool)  [unwired: 2 in, 2 out]
                  n67 = Compound Arithmetic op=OR(w138, "Stop NI", w134) -> (w137:bool)
                  n68 = Wait Until Next ms Multiple(millisecond multiple=u32 250) -> ()  [unwired: 1 out]
                }
                n69 = call <vilib>:"DAQmx Stop Task.vi"("task/channels in"=w124, "error in"=w125) -> ("task out"=w127:refnum<k21>, "error out"=w126:errorcluster)  [unwired: 12 in]
                n70 = call <vilib>:"DAQmx Clear Task.vi"("task in"=w127, "error in"=w126) -> ()  [unwired: 13 in, 1 out]
              }
            }
            n71 = property on="stop" class="Bool (strict)"() -> ("Value"=w109:bool)  [unwired: 2 in, 2 out]
            n72 = property on="Stop NI" class="Bool (strict)"("Value"=w105) -> ()  [unwired: 2 in, 2 out]
            n73 = property on="Start NI" class="Bool (strict)"("Value"=w105) -> ()  [unwired: 2 in, 2 out]
            n74 = Wait Until Next ms Multiple(millisecond multiple=u32 250) -> ()  [unwired: 1 out]
          }
          n75 = while {
            tunnel: w73 -> [w294]
            stop <- w295 stop-if-true
            n76 = event shown="[2] \"stop\": Value Change" {
              selector: _ -> [_ _ _]
              dyn-events: _ -> [_ _ _]
              timeout: _ -> [_ _ _]
              tunnel: [_ _ TRUE] -> w295
              tunnel: w294 -> [_ w297 _]
              event Timeout {
                n77 = event-data() -> ()  [unwired: 1 in, 3 out]
              }
              event "emergency stop": Value Change {
                n78 = event-data() -> ()  [unwired: 1 in, 1 out]
                n79 = local read "Sample\nScan"() -> (w296:bool)
                n80 = stacked-sequence {
                  tunnel: w297 -> [_ w303 _]
                  tunnel: w296 -> [w298 _ _]
                  frame #0 {
                    n81 = case shown="True" w298 {
                      selector: w298 -> [_ w299]
                      frame False {
                      }
                      frame True {
                        n82 = property on="Stop Scan (2D)" class="Bool (strict)"("Val(Sgnl)"=w299) -> ()  [unwired: 2 in, 2 out]
                      }
                    }
                  }
                  frame #1 {
                    w302 = u16 5 items=["none", "1", "2", "3", "4", "all"] ("Motor")
                    n83 = call "Read_only_Manipulator.vi"("Motor"=w302, "Value"="0", "Command"=Set_Parameter."Slew (SL)", "VISA resource name"=w303) -> ()  [unwired: 4 in, 4 out]
                  }
                  frame #2 {
                    n84 = local write "emergency stop"(FALSE ("emergency stop")) -> ()
                  }
                }
              }
              event "stop": Value Change {
                n85 = event-data() -> ()  [unwired: 1 in, 4 out]
              }
            }
            n86 = Wait Until Next ms Multiple(millisecond multiple=u32 100) -> ()  [unwired: 1 out]
          }
          n87 = while {
            tunnel: w76 -> [w143]
            tunnel: w74 -> [w145]
            tunnel: w70 -> [w144]
            tunnel: w75 -> [w142]
            stop <- w149 stop-if-true
            n88 = case shown="False" "Start K" {
              selector: "Start K" -> [w153 _]
              tunnel: [w153 w164] -> w150
              tunnel: [w153 w164] -> w147
              tunnel: [w152 w158] -> w146
              tunnel: w145 -> [_ w163]
              tunnel: w144 -> [w152 w162]
              tunnel: w143 -> [_ w161]
              tunnel: w142 -> [_ w160]
              frame False {
              }
              frame True {
                w164 = FALSE
                n89 = case shown="False" w161 {
                  selector: w161 -> [w170 w233]
                  tunnel: [w169 w241] -> w159
                  tunnel: w163 -> [w177 w240]
                  tunnel: w162 -> [w176 w239]
                  tunnel: w160 -> [w175 _]
                  tunnel: [w168 w234] -> w157
                  tunnel: TRUE ("Check Completeness of Data (true)") -> [w167 w230]
                  tunnel: "Current\nRange Ch2" -> [w166 w232]
                  tunnel: "Current\nRange Ch1" -> [w165 w231]
                  frame False {
                    n90 = call "Visa_Open_RS-232.vi"("error in (no error)"=w176, "Cluster"=w175, "ComPort"=w177) -> ("error out"=w173:errorcluster, "VISA resource name out"=w174:refnum<visa-resource-name>)  [unwired: 7 in]
                    n91 = call "Set_Current_Range.vi"("Current Range Ch 2"=w166, "GPIB (t) / RS-232 (f)"=w170, "Current Range Ch 1"=w165, "error in (no error)"=w173, "VISA resource name"=w174) -> ("error out"=w171:errorcluster, "VISA resource name out"=w172:refnum<visa-resource-name>)  [unwired: 5 in]
                    n92 = while {
                      tunnel: w172 -> [w189]
                      tunnel: w171 -> [w181]
                      tunnel: [w194] -> w168
                      tunnel: [w185] -> w169
                      tunnel: w167 -> [w193]
                      stop <- w178 stop-if-true
                      n93 = Add(x=u32 75 ("milliseconds to wait"), y=u32 37) -> (x+y=w183:u32)
                      n94 = call "Keithley_VISA_Write_Only.vi"("error in (no error)"=w181, "milliseconds to wait"=w183, "command"="TRAC:CLE\nTRAC:FEED:CONT NEXT\nFORM:ELEM CURR\nINIT", "VISA resource name"=w189) -> ("error out"=w187:errorcluster, "VISA resource name out"=w188:refnum<visa-resource-name>)  [unwired: 6 in]
                      n95 = case shown="True" w193 {
                        tunnel: w188 -> [w213 w228]
                        tunnel: w187 -> [w211 w229]
                        tunnel: [w213 w220] -> w192
                        tunnel: [TRUE w216] -> w190
                        tunnel: [w210 w219] -> w191
                        frame False {
                          n96 = stacked-sequence {
                            tunnel: w211 -> [w215]
                            tunnel: [w215] -> w210
                            frame #0 {
                              n97 = Wait (ms)(milliseconds to wait=u32 50) -> ()  [unwired: 1 out]
                            }
                          }
                        }
                        frame True {
                          # "See how many points\nare in the buffer"
                          n98 = call "Keithley_VISA_Read_Write.vi"("error in (no error)"=w229, "milliseconds to wait"=u32 25, "command"="STAT:MEAS?" ("write buffer"), "VISA resource name"=w228) -> ("error out"=w224:errorcluster, "read buffer"=w225:string, "VISA resource name out"=w223:refnum<visa-resource-name>)  [unwired: 5 in]
                          n99 = Decimal String To Number(string=w225) -> (number=w218:i32)  [unwired: 2 in, 1 out]
                          n100 = call "use_or_discard_data.vi"("Status"=w225) -> ("use data"=w216:bool)
                          n101 = property on="Status" class="DigNum (strict)"("Value"=w218) -> ()  [unwired: 2 in, 2 out]
                          n102 = call "Keithley_VISA_Read_Write.vi"("error in (no error)"=w224, "milliseconds to wait"=u32 25, "command"=":TRAC:POIN:ACT?" ("write buffer"), "VISA resource name"=w223) -> ("error out"=w219:errorcluster, "read buffer"=w217:string, "VISA resource name out"=w220:refnum<visa-resource-name>)  [unwired: 5 in]
                          n103 = property on="use data" class="Bool (strict)"("Value"=w216) -> ()  [unwired: 2 in, 2 out]
                          n104 = property on="buffer" class="Str"("Value"=w217) -> ()  [unwired: 2 in, 2 out]
                        }
                      }
                      n105 = case shown="True" w190 {
                        tunnel: [w197 w207] -> w194
                        tunnel: [w195 w206] -> w185
                        tunnel: w192 -> [w197 w209]
                        tunnel: w191 -> [w196 w208]
                        frame False {
                          n106 = stacked-sequence {
                            tunnel: w196 -> [w199]
                            tunnel: [w199] -> w195
                            frame #0 {
                              n107 = Wait (ms)(milliseconds to wait=u32 25) -> ()  [unwired: 1 out]
                            }
                          }
                        }
                        frame True {
                          n108 = Concatenate Strings("TRAC:DATA?", "\n") -> (w205:string)
                          n109 = call "Get Keithley Data.vi"("GPIB = true, RS-232 = false"=FALSE, "wait after write (ms)"=u32 25 ("milliseconds to wait"), "error in (no error)"=w208, "Command"=w205, "VISA resource name"=w209) -> ("error out"=w206:errorcluster, "Data"=w201:dbl[], "VISA resource name out"=w207:refnum<visa-resource-name>)  [unwired: 3 in, 1 out]
                          n110 = property on="Data" class="Arr (strict)"("Value"=w201) -> ()  [unwired: 2 in, 2 out]
                        }
                      }
                      n111 = property on="stop" class="Bool (strict)"() -> ("Value"=w180:bool)  [unwired: 2 in, 2 out]
                      n112 = property on="Stop K" class="Bool (strict)"() -> ("Value"=w179:bool)  [unwired: 2 in, 2 out]
                      n113 = Or(x=w180, y=w179) -> (x .or. y?=w178:bool)
                    }
                  }
                  frame True {
                    # "Sample rate (Hz)"
                    n114 = property class="Instr"(reference=w240, error in=w239, "Unaddress"=TRUE ("GPIB Settings:Unaddressing")) -> (reference out=w238:refnum<visa-resource-name>, error out=w237:errorcluster)
                    n115 = Divide(x=1000, y=10) -> (x/y=w244:dbl)
                    n116 = To Unsigned Long Integer(number=w244) -> (unsigned 32bit integer=w243:u32)
                    n117 = call "Set_Current_Range.vi"("Current Range Ch 2"=w232, "GPIB (t) / RS-232 (f)"=w233, "Current Range Ch 1"=w231, "error in (no error)"=w237, "VISA resource name"=w238) -> ("error out"=w235:errorcluster, "VISA resource name out"=w236:refnum<visa-resource-name>)  [unwired: 5 in]
                    n118 = while {
                      tunnel: w236 -> [w261]
                      tunnel: w235 -> [w254]
                      tunnel: [w260] -> w234
                      tunnel: [w259] -> w241
                      tunnel: w230 -> [w257]
                      tunnel: w243 -> [w253]
                      tunnel: w233 -> [w247]
                      stop <- w249 stop-if-true
                      n119 = Wait Until Next ms Multiple(millisecond multiple=w253) -> ()  [unwired: 1 out]
                      n120 = VISA Write(VISA resource name=w261, write buffer="TRAC:CLEAR\nTRACE:FEED:CONT NEXT\nFORM:ELEM CURR\nINIT", error in (no error)=w254) -> (VISA resource name out=w258:refnum<visa-resource-name>, error out=w252:errorcluster)  [unwired: 1 out]
                      n121 = case shown="True" w257 {
                        tunnel: w258 -> [w274 w288]
                        tunnel: w252 -> [w273 w287]
                        tunnel: [w274 w282] -> w256
                        tunnel: [w273 w281] -> w255
                        tunnel: [TRUE ("use data") w276] -> w248
                        frame False {
                        }
                        frame True {
                          # "points in buffer"
                          n122 = VISA Write(VISA resource name=w288, write buffer="STAT:MEAS?", error in (no error)=w287) -> (VISA resource name out=w290:refnum<visa-resource-name>, error out=w289:errorcluster)  [unwired: 1 out]
                          n123 = VISA Read(VISA resource name=w290, byte count=u32 10, error in (no error)=w289) -> (VISA resource name out=w280:refnum<visa-resource-name>, read buffer=w277:string, error out=w279:errorcluster)  [unwired: 1 out]
                          n124 = VISA Write(VISA resource name=w280, write buffer=":TRAC:POIN:ACT?", error in (no error)=w279) -> (VISA resource name out=w284:refnum<visa-resource-name>, error out=w283:errorcluster)  [unwired: 1 out]
                          n125 = Decimal String To Number(string=w277) -> (number=→"Status":i32)  [unwired: 2 in, 1 out]
                          n126 = call "use_or_discard_data.vi"("Status"=w277) -> ("use data"=w276:bool)
                          "use data" <- w276
                          n127 = VISA Read(VISA resource name=w284, byte count=u32 10, error in (no error)=w283) -> (VISA resource name out=w282:refnum<visa-resource-name>, read buffer=→"buffer":string, error out=w281:errorcluster)  [unwired: 1 out]
                        }
                      }
                      n128 = case shown="True" w248 {
                        tunnel: [w264 w268] -> w260
                        tunnel: [w263 w267] -> w259
                        tunnel: w256 -> [w264 w270]
                        tunnel: w255 -> [w263 w269]
                        tunnel: w247 -> [_ w265]
                        frame False {
                        }
                        frame True {
                          n129 = call "Get Keithley Data.vi"("GPIB = true, RS-232 = false"=w265, "error in (no error)"=w269, "Command"="TRAC:DATA?", "VISA resource name"=w270) -> ("error out"=w267:errorcluster, "Data"=→"Data":dbl[], "VISA resource name out"=w268:refnum<visa-resource-name>)  [unwired: 4 in, 1 out]
                        }
                      }
                      n130 = property on="stop" class="Bool (strict)"() -> ("Value"=w251:bool)  [unwired: 2 in, 2 out]
                      n131 = Or(x=w251, y="Stop K") -> (x .or. y?=w249:bool)
                    }
                  }
                }
                n132 = VISA Close(VISA resource name=w157, error in (no error)=w159) -> (error out=w158:errorcluster)
              }
            }
            "error Keithley" <- w146
            n133 = property on="Start K" class="Bool (strict)"("Value"=w150) -> ()  [unwired: 2 in, 2 out]
            n134 = property on="Stop K" class="Bool (strict)"("Value"=w147) -> ()  [unwired: 2 in, 2 out]
            n135 = property on="stop" class="Bool (strict)"() -> ("Value"=w149:bool)  [unwired: 2 in, 2 out]
            n136 = Wait Until Next ms Multiple(millisecond multiple=u32 250) -> ()  [unwired: 1 out]
          }
          n137 = while {
            tunnel: w73 -> [w325]
            tunnel: w70 -> [w324]
            tunnel: w68 -> [w320]
            tunnel: w78 -> [w319]
            tunnel: w72 -> [w317]
            tunnel: w74 -> [w316]
            tunnel: path "G:/My Drive/DATA" ("file path (use dialog)") -> [w315]
            tunnel: w76 -> [w314]
            tunnel: w75 -> [w313]
            tunnel: w71 -> [w312]
            tunnel: w67 -> [w311]
            tunnel: w66 -> [w310]
            shift-right: [w308] -> _
            shift-left: w64 -> [w309]
            i -> [w306]
            stop <- w321 stop-if-true
            n138 = event shown="[45] \"Next Scan Step\": Value Change" {
              selector: _ -> [_ _ _ _ _ _ _ _ _ _ _ _ _ _ _ _ _ _ _ _ _ _ _ _ _ _ _ _ _ _ _ _ _ _ _ _ _ _ _ _ _ _ _ _ _ _ _ _ _ _ _ _ _ _ _ _ _ _ _ _ _ _ _ _ _ _]
              dyn-events: _ -> [_ _ _ _ _ _ _ _ _ _ _ _ _ _ _ _ _ _ _ _ _ _ _ _ _ _ _ _ _ _ _ _ _ _ _ _ _ _ _ _ _ _ _ _ _ _ _ _ _ _ _ _ _ _ _ _ _ _ _ _ _ _ _ _ _ _]
              timeout: 750 -> [_ _ _ _ _ _ _ _ _ _ _ _ _ _ _ _ _ _ _ _ _ _ _ _ _ _ _ _ _ _ _ _ _ _ _ _ _ _ _ _ _ _ _ _ _ _ _ _ _ _ _ _ _ _ _ _ _ _ _ _ _ _ _ _ _ _]
              tunnel: w325 -> [w371 _ w513 w520 w533 w540 _ w559 w714 w874 w951 w1023 w1110 w1215 _ _ _ _ w1374 w1377 w1387 w1400 w1469 w1478 w1503 w1528 w1616 w1651 w1686 w1718 _ _ w1785 w1833 w1932 _ _ w2032 w2158 _ w2293 w2307 _ w2358 w2386 _ w2440 _ w2477 w2540 _ _ _ _ _ _ _ _ _ _ _ _ _ _ w2659 w2681]
              tunnel: w324 -> [w370 _ w514 w519 w532 w539 _ w560 w715 w873 w950 w1022 w1109 w1214 _ _ _ _ w1373 w1376 w1386 w1399 w1468 w1479 w1504 w1529 w1615 w1650 w1687 w1717 w1734 _ w1784 w1832 w1931 _ _ w2034 w2161 w2251 w2292 w2306 _ w2365 w2371 w2392 _ _ w2478 w2539 w2543 _ _ _ _ _ _ _ _ _ _ _ _ w2624 w2658 w2680]
              tunnel: [w348 _ w511 w517 w529 w537 _ w544 w701 w870 w955 w1029 w1093 w1199 _ _ _ _ w1371 w1380 w1390 w1398 w1472 w1490 w1515 w1536 w1627 w1648 w1684 w1716 _ _ w1777 w1820 w1919 _ _ w2008 w2131 _ w2301 w2331 _ _ w2382 w2394 _ _ w2471 w2535 _ _ _ _ _ _ _ _ _ _ _ _ _ _ w2661 w2679] -> w323
              tunnel: [w345 _ w512 w516 w528 w538 _ w548 w704 w867 w942 w1016 w1089 w1196 _ _ _ _ w1364 w1381 w1391 w1397 w1473 w1489 w1514 w1535 w1626 w1649 w1685 w1704 w1733 _ w1776 w1817 w1909 _ _ w1986 w2109 w2252 w2300 w2330 _ w2362 w2376 w2393 _ _ w2474 w2532 w2542 _ _ _ _ _ _ _ _ _ _ _ _ w2623 w2660 w2670] -> w322
              tunnel: [_ _ _ _ _ _ _ _ _ _ _ _ _ _ _ _ _ _ _ _ _ _ _ _ _ _ _ _ _ _ _ _ _ _ _ _ _ _ _ _ _ _ _ _ _ _ _ _ _ _ _ _ _ _ _ _ _ _ _ _ _ _ _ _ _ TRUE] -> w321
              tunnel: w320 -> [_ _ _ _ _ _ _ _ _ _ _ _ _ _ _ _ _ _ _ _ _ _ _ _ _ _ _ w1646 w1688 w1713 w1737 _ _ _ _ _ _ _ _ _ _ _ _ w2366 w2387 _ _ _ _ _ _ _ _ _ _ _ _ _ _ _ _ _ _ _ _ w2667]
              tunnel: w317 -> [w327 _ _ _ _ _ _ w552 w708 _ _ _ w1106 w1211 _ _ _ _ w1372 _ _ w1403 _ _ _ _ _ w1644 w1683 w1712 _ _ _ _ w1907 _ _ w2033 w2162 _ _ _ _ _ _ _ _ _ w2476 _ _ _ _ _ _ _ _ _ _ _ _ _ _ _ _ w2678]
              tunnel: w316 -> [_ _ _ _ _ _ _ _ _ _ _ _ _ _ _ _ _ _ _ _ _ _ _ _ _ _ _ _ _ _ _ _ _ _ _ _ _ w2000 w2123 _ _ _ _ _ _ _ _ _ _ _ _ _ _ _ _ _ _ _ _ _ _ _ _ _ _ _]
              tunnel: w315 -> [w337 _ _ _ _ _ _ _ _ _ _ _ _ _ _ _ _ _ _ _ _ _ _ _ _ _ _ _ _ _ _ _ _ _ _ _ _ w1984 w2105 _ _ _ _ _ _ _ _ _ _ _ _ _ _ _ _ _ _ _ _ _ _ _ _ _ _ _]
              tunnel: w314 -> [_ _ _ _ _ _ _ _ _ _ _ _ _ _ _ _ _ _ _ _ _ _ _ _ _ _ _ _ _ _ _ _ _ _ _ _ _ w1998 w2121 _ _ _ _ _ _ _ _ _ _ _ _ _ _ _ _ _ _ _ _ _ _ _ _ _ _ _]
              tunnel: w313 -> [_ _ _ _ _ _ _ _ _ _ _ _ _ _ _ _ _ _ _ _ _ _ _ _ _ _ _ _ _ _ _ _ _ _ _ _ _ w2001 w2124 _ _ _ _ _ _ _ _ _ _ _ _ _ _ _ _ _ _ _ _ _ _ _ _ _ _ _]
              tunnel: w312 -> [_ _ _ _ _ _ _ _ _ _ _ _ _ _ _ _ _ _ _ _ _ _ _ _ _ _ _ _ _ _ _ _ _ _ _ _ _ _ _ _ _ _ _ _ _ _ w2439 w2462 _ _ _ _ _ _ _ _ _ _ _ _ _ _ _ _ _ _]
              tunnel: w311 -> [_ _ _ _ _ _ _ _ _ _ _ _ _ _ _ _ _ _ _ _ _ _ _ _ _ _ _ _ _ _ _ _ _ _ _ _ _ _ _ _ _ _ _ _ _ _ w2442 _ _ _ _ _ _ _ _ _ _ _ _ _ _ _ _ _ _ _]
              tunnel: w310 -> [_ _ _ _ _ _ _ _ _ _ _ _ _ _ _ _ _ _ _ _ _ _ _ _ _ _ _ _ _ _ _ _ _ _ _ _ _ _ _ _ _ _ _ _ _ w2395 _ _ _ _ _ _ _ _ _ _ _ _ _ _ _ _ _ w2622 _ _]
              tunnel: w309 -> [w336 _ _ _ _ _ _ _ _ _ _ _ _ _ _ _ _ _ _ _ _ _ _ _ _ _ _ _ _ _ _ _ _ _ _ _ _ _ _ _ _ _ _ _ _ _ _ _ _ _ _ _ _ _ _ _ _ _ _ _ _ _ _ _ _ _]
              tunnel: [w344 _ _ _ _ _ _ _ _ _ _ _ _ _ _ _ _ _ _ _ _ _ _ _ _ _ _ _ _ _ _ _ _ _ _ _ _ _ _ _ _ _ _ _ _ _ _ _ _ _ _ _ _ _ _ _ _ _ _ _ _ _ _ _ _ _] -> w308
              tunnel: w306 -> [w331 _ _ _ _ _ _ _ _ _ _ _ _ _ _ _ _ _ _ _ _ _ _ _ _ _ _ _ _ _ _ _ _ _ _ _ _ _ _ _ _ _ _ _ _ _ _ _ _ _ _ _ _ _ _ _ _ _ _ _ _ _ _ _ _ _]
              event Timeout {
                # "Check movement and limit switches less often?"
                n139 = event-data() -> ()  [unwired: 1 in, 3 out]
                n140 = case shown="True" TRUE {
                  tunnel: w371 -> [w373 w381]
                  tunnel: w370 -> [w372 w380]
                  tunnel: [w373 w377] -> w369
                  tunnel: [w372 w376] -> w368
                  frame False {
                  }
                  frame True {
                    n141 = property class="Instr"(reference=w381, error in=w380) -> (reference out=w379:refnum<visa-resource-name>, error out=w378:errorcluster, "Bytes at Port"=w375:u32)
                    n142 = VISA Read(VISA resource name=w379, byte count=w375, error in (no error)=w378) -> (VISA resource name out=w377:refnum<visa-resource-name>, read buffer=w374:string, error out=w376:errorcluster)  [unwired: 1 out]
                    n143 = String Length(string=w374) -> (length=w383:i32)
                    n144 = Not Equal To 0?(x=w383) -> (x != 0?=w382:bool)
                    n145 = case shown="False" w382 {
                      tunnel: w374 -> [_ w384]
                      frame False {
                      }
                      frame True {
                        n146 = property on="Answer" class="Str"() -> ("Text.Text"=w386:string)  [unwired: 2 in, 2 out]
                        n147 = Concatenate Strings(w386, w384) -> (w385:string)
                        n148 = property on="Answer" class="Str"("Text.Text"=w385) -> ()  [unwired: 2 in, 2 out]
                      }
                    }
                  }
                }
                n149 = Quotient & Remainder(x=w331, y=3) -> (x-y*floor(x/y)=w328:i32)  [unwired: 1 out]
                n150 = global read "Global_external_move_cmd.vi" "external command"() -> (w329:bool)
                n151 = case shown="1" w328 {
                  tunnel: w369 -> [w390 w396 w402]
                  tunnel: w368 -> [w389 w395 w401]
                  tunnel: [w390 w392 w400] -> w363
                  tunnel: w327 -> [w388 w393 w398]
                  tunnel: [w389 w391 w399] -> w347
                  tunnel: [w388 w393 w398] -> w332
                  frame 0, Default {
                  }
                  frame 1 {
                    # "Is any\nmotor\nmoving?"
                    n152 = call "Is_any_motor_moving.vi"("error in (no error)"=w395, "VISA resource name"=w396) -> ("error out"=w391:errorcluster, "Motor Moving"=→"MM?":bool, "VISA ressource out"=w392:refnum<visa-resource-name>)  [unwired: 6 in, 1 out]
                  }
                  frame 2 {
                    n153 = call "Any_limit_switch_active.vi"("Echo Mode"=w398, "error in (no error)"=w401, "VISA resource name"=w402) -> ("error out"=w403:errorcluster, "limit switch cluster"=→"limit switch cluster":T2, "VISA ressource out"=w400:refnum<visa-resource-name>, "Any Limit Switch?"=w404:bool)  [unwired: 4 in, 1 out]
                    n154 = call "Play_Beep_Sound.vi"("error in"=w403, "Play Sound (def=t)"=w404, "duration (s)"=u32 1) -> ("error out"=w399:errorcluster)  [unwired: 8 in]
                  }
                }
                n155 = case shown="False" w329 {
                  selector: w329 -> [_ w387]
                  frame False {
                  }
                  frame True {
                    n156 = property on="ext. Cmd" class="Bool (strict)"("Val(Sgnl)"=w387) -> ()  [unwired: 2 in, 2 out]
                  }
                }
                n157 = global read "Global_Next_Scan_Position.vi" "XAS(f) / XPS(t)"() -> (w333:bool)
                n158 = local read "pause scan"() -> (w366:bool)
                n159 = local read "Sample\nScan"() -> (w365:bool)
                n160 = property on="Pos Unit" class="Ring (strict)"() -> ("Value"=w364:T8)  [unwired: 2 in, 2 out]
                n161 = Not(x=w366) -> (.not. x?=w367:bool)
                n162 = call "Read_All_Motor_Positions.vi"("Echo Mode"=w332, "error in"=w347, "Pos Unit"=w364, "VISA resource name"=w363) -> ("error out"=w346:errorcluster, "Manipulator Pos (Steps)"=w339:i32[], "Manipulator Pos (Pos Unit Input)"=w361:dbl[], "VISA out"=w348:refnum<visa-resource-name>, "Manipulator Pos (Microns/Degrees)"=w362:dbl[])  [unwired: 3 in]
                n163 = Compound Arithmetic op=AND(w367, w365) -> (w335:bool)
                n164 = Or(x=w333, y=w335) -> (x .or. y?=w334:bool)
                n165 = case shown="True" w334 {
                  tunnel: w346 -> [w407 w420]
                  tunnel: [w407 w419] -> w345
                  tunnel: w339 -> [_ w412]
                  tunnel: [w406 w418] -> w344
                  tunnel: w336 -> [w406 w411]
                  tunnel: w333 -> [_ w408]
                  frame False {
                  }
                  frame True {
                    n166 = global read "Global_Next_Scan_Position.vi" "Next Scan Pos"() -> (w413:i32[])
                    "Next Pos" <- w413
                    n167 = global read "Global_Next_Scan_Position.vi" "MM Scan"() -> (w415:u16)
                    n168 = call "verfluchter_Kackdreck.vi"("XAS (false, def), XPS (true)"=w408, "Last Motor moved in Scan"=w411) -> ("Last Motor Moved in Scan (Out)"=w410:u16)  [unwired: 9 in]
                    n169 = call "Delta_Arrays_Equal_To_Zero.vi"("max difference (0)"=1000, "Current Manipulator Position"=w412, "Next Scan Position"=w413) -> ("At Pos?"=w414:bool)  [unwired: 8 in]
                    "At Next Pos?" <- w414
                    n170 = Not Equal?(x=w410, y=w415) -> (x != y?=w417:bool)
                    n171 = And(x=w417, y=w414) -> (x .and. y?=w416:bool)
                    n172 = case shown="True" w416 {
                      tunnel: w420 -> [w422 w429]
                      tunnel: [w422 w428] -> w419
                      tunnel: [w421 w424] -> w418
                      tunnel: w415 -> [_ w424]
                      tunnel: w410 -> [w421 _]
                      tunnel: w408 -> [_ w425]
                      frame False {
                      }
                      frame True {
                        n173 = local read "Switch Laser"() -> (w427:bool)
                        n174 = Not(x=w427) -> (.not. x?=w426:bool)
                        n175 = And(x=w426, y=w425) -> (x .and. y?=w423:bool)
                        n176 = case shown="False" w425 {
                          tunnel: w429 -> [w430 w433]
                          tunnel: [w430 w432] -> w428
                          tunnel: w423 -> [_ w434]
                          frame False {
                            n177 = property on="Next Scan Step" class="Bool (strict)"("Val(Sgnl)"=TRUE ("Value (Signaling)")) -> ()  [unwired: 2 in, 2 out]
                          }
                          frame True {
                            n178 = case shown="True" w434 {
                              tunnel: w433 -> [w435 w436]
                              tunnel: [w435 w436] -> w432
                              frame False {
                              }
                              frame True {
                                n179 = call "PoD_Laser_ON_OFF.vi"("Enable VI"=TRUE, "Laser ON (t) / OFF (f)"=FALSE) -> ("AO switched"=w437:bool)  [unwired: 9 in]
                                n180 = Not(x=w437) -> (.not. x?=w438:bool)
                                n181 = global write "Switch _Laser_Global.vi" "Laser (on, t; off, f)"(w438) -> ()
                              }
                            }
                          }
                        }
                      }
                    }
                  }
                }
                n182 = call "save_motor_positions_to_log_file.vi"("Save Time (s)"=30, "Manipulator Pos (Steps)"=w339, "file path"=w337) -> ()  [unwired: 7 in, 2 out]
                n183 = Index Array(array=w361, index #1=0 ("index"), index #2=1 ("index"), index #3=2 ("index"), index #4=3 ("index")) -> (element #1=w343:dbl, element #2=w342:dbl, element #3=w341:dbl, element #4=w340:dbl)
                "M4 XPS" <- w340
                "M3 XPS" <- w341
                "M2 XPS" <- w342
                "M1 XPS" <- w343
                n184 = Index Array(array=w339, index #1=0 ("index"), index #2=1 ("index"), index #3=2 ("index"), index #4=3 ("index")) -> (element #1=w352:i32, element #2=w351:i32, element #3=w350:i32, element #4=w349:i32)
                n185 = global write "Pressure_Ch_1_2_Manipulator_Pos.vi" "Manipulator Pos steps"(w339) -> ()
                n186 = global write "Pressure_Ch_1_2_Manipulator_Pos.vi" "Manipulator Pos"(w362) -> ()
                n187 = local write "Pos 1 (Steps)"(w352) -> ()
                n188 = local write "Pos 1"(w343) -> ()
                n189 = local write "Pos 2 (Steps)"(w351) -> ()
                n190 = local write "Pos 2"(w342) -> ()
                n191 = local write "Pos 3 (Steps)"(w350) -> ()
                n192 = local write "Pos 3"(w341) -> ()
                n193 = local write "Pos 4 (Steps)"(w349) -> ()
                n194 = local write "Pos 4 [Angle]"(w340) -> ()
                "Motor 6" <- w336
              }
              event "ext. Cmd": Value Change {
                w445 = FALSE ("external command")
                n195 = event-data() -> ()  [unwired: 1 in, 6 out]
                n196 = global read "Global_external_move_cmd.vi" "Direction (+ true, - false)"() -> (w451:bool)
                n197 = global read "Pressure_Ch_1_2_Manipulator_Pos.vi" "Manipulator Pos steps"() -> (w448:i32[])
                n198 = global read "Global_external_move_cmd.vi" "Unit of Move"() -> (w441:T8)
                n199 = global read "Global_external_move_cmd.vi" "Rel Steps"() -> (w443:string)
                n200 = global read "Global_external_move_cmd.vi" "Motor"() -> (w442:u16)
                n201 = case shown="4" w442 {
                  tunnel: w451 -> [w491 w495 w499 w503]
                  tunnel: TRUE -> [w490 w494 w498 w502]
                  frame 1 {
                    n202 = case shown="False" w491 {
                      tunnel: w490 -> [w492 w493]
                      frame False {
                        n203 = property on="move to detector" class="Bool (strict)"("Val(Sgnl)"=w492) -> ()  [unwired: 2 in, 2 out]
                      }
                      frame True {
                        n204 = property on="move away detector" class="Bool (strict)"("Val(Sgnl)"=w493) -> ()  [unwired: 2 in, 2 out]
                      }
                    }
                  }
                  frame 2 {
                    n205 = case shown="False" w495 {
                      tunnel: w494 -> [w496 w497]
                      frame False {
                        n206 = property on="move to x-rays" class="Bool (strict)"("Val(Sgnl)"=w496) -> ()  [unwired: 2 in, 2 out]
                      }
                      frame True {
                        n207 = property on="move away x-rays" class="Bool (strict)"("Val(Sgnl)"=w497) -> ()  [unwired: 2 in, 2 out]
                      }
                    }
                  }
                  frame 3, Default {
                    n208 = case shown="False" w499 {
                      tunnel: w498 -> [w500 w501]
                      frame False {
                        n209 = property on="move up" class="Bool (strict)"("Val(Sgnl)"=w500) -> ()  [unwired: 2 in, 2 out]
                      }
                      frame True {
                        n210 = property on="move down" class="Bool (strict)"("Val(Sgnl)"=w501) -> ()  [unwired: 2 in, 2 out]
                      }
                    }
                  }
                  frame 4 {
                    n211 = case shown="False" w503 {
                      tunnel: w502 -> [w504 w505]
                      frame False {
                        n212 = property on="move clockwise" class="Bool (strict)"("Val(Sgnl)"=w504) -> ()  [unwired: 2 in, 2 out]
                      }
                      frame True {
                        n213 = property on="move counterclockwise" class="Bool (strict)"("Val(Sgnl)"=w505) -> ()  [unwired: 2 in, 2 out]
                      }
                    }
                  }
                }
                n214 = case shown="2" w441 {
                  tunnel: w443 -> [w454 w461 w468 w475 w482]
                  tunnel: [w454 w460 w467 w474 w481] -> _
                  tunnel: w442 -> [_ w462 w469 w476 w483]
                  tunnel: [w453 w456 w463 w470 w477] -> w444
                  frame 0, Default {
                    n215 = Scan Value(string=w454, format string="%.6f") -> (value=w453:dbl)  [unwired: 1 in, 1 out]
                  }
                  frame 1 {
                    n216 = call "Conversion_Simple.vi"("Input = DBL/String (DBL[false])"=TRUE, "Motor"=w462, "Output Unit"=Unit_Control."Microsteps [TMC]" ("Input Unit"), "Input Unit"=Unit_Control."Micron", "Input String"=w461) -> (2:"Output"=w460:string, 3:"Output"=w456:dbl)  [unwired: 5 in]
                  }
                  frame 2 {
                    n217 = call "Conversion_Simple.vi"("Input = DBL/String (DBL[false])"=TRUE, "Motor"=w469, "Output Unit"=Unit_Control."Microsteps [TMC]" ("Input Unit"), "Input Unit"=Unit_Control."Millimeter", "Input String"=w468) -> (2:"Output"=w467:string, 3:"Output"=w463:dbl)  [unwired: 5 in]
                  }
                  frame 3 {
                    n218 = call "Conversion_Simple.vi"("Input = DBL/String (DBL[false])"=TRUE, "Motor"=w476, "Output Unit"=Unit_Control."Microsteps [TMC]" ("Input Unit"), "Input Unit"=Unit_Control."Centimeter", "Input String"=w475) -> (2:"Output"=w474:string, 3:"Output"=w470:dbl)  [unwired: 5 in]
                  }
                  frame 4 {
                    n219 = call "Conversion_Simple.vi"("Input = DBL/String (DBL[false])"=TRUE, "Motor"=w483, "Output Unit"=Unit_Control."Microsteps [TMC]" ("Input Unit"), "Input Unit"=Unit_Control."Inches", "Input String"=w482) -> (2:"Output"=w481:string, 3:"Output"=w477:dbl)  [unwired: 5 in]
                  }
                }
                n220 = call "Motor_Pos_from_GlobaL_Variable.vi"("Motor"=w442, "Manipulator Pos IN"=w448) -> ("Motor Index"=w449:i32, "Motor Pos"=w450:i32)  [unwired: 8 in]
                n221 = case shown="False" w451 {
                  tunnel: w444 -> [w485 w488]
                  tunnel: w450 -> [w486 w489]
                  tunnel: [w484 w487] -> w447
                  frame False {
                    n222 = Subtract(x=w486, y=w485) -> (x-y=w484:dbl)
                  }
                  frame True {
                    n223 = Add(x=w488, y=w489) -> (x+y=w487:dbl)
                  }
                }
                n224 = Replace Array Subset(array=w448, new element=w447, index=w449) -> (w446:i32[])
                n225 = global write "Global_external_move_cmd.vi" "external command"(w445) -> ()
                n226 = local write "ext. Cmd"(w445) -> ()
                n227 = property on="Rel Steps" class="Str"("Value"=w443) -> ()  [unwired: 2 in, 2 out]
                n228 = property on="Unit of Move" class="Ring (strict)"("Value"=w441) -> ()  [unwired: 2 in, 2 out]
                n229 = global write "Global_external_move_cmd.vi" "Goal Man Pos (Steps)"(w446) -> ()
              }
              event "Send Cmd": Value Change {
                n230 = event-data() -> ()  [unwired: 1 in, 6 out]
                n231 = call "Read_only_Manipulator.vi"("Print?"="Print", "Motor"="Motor", "error in (no error)"=w514, "Value"="Value", "Command"="Command", "VISA resource name"=w513) -> ("error out"=w515:errorcluster, "Transmitted String"=→"Transmitted String":string, "VISA ressource out"=w511:refnum<visa-resource-name>)  [unwired: 2 in, 1 out]
                n232 = call <vilib>:"General Error Handler.vi"("error in (no error)"=w515) -> ("error out"=w512:errorcluster)  [unwired: 10 in, 4 out]
              }
              event "Send Cmd as is": Value Change {
                n233 = event-data() -> ()  [unwired: 1 in, 6 out]
                n234 = VISA Write(VISA resource name=w520, write buffer="Send As Is String", error in (no error)=w519) -> (VISA resource name out=w522:refnum<visa-resource-name>, error out=w521:errorcluster)  [unwired: 1 out]
                n235 = stacked-sequence {
                  tunnel: w522 -> [w525]
                  tunnel: [w525] -> w517
                  tunnel: w521 -> [w524]
                  tunnel: [w524] -> w516
                  frame #0 {
                    n236 = Wait (ms)(milliseconds to wait=u32 50) -> ()  [unwired: 1 out]
                  }
                }
                n237 = property on="Transmitted String" class="Str"("Text.Text"="Send As Is String") -> ()  [unwired: 2 in, 2 out]
              }
              event "Print Error": Value Change {
                n238 = event-data() -> ()  [unwired: 1 in, 6 out]
                n239 = local read "Motor"() -> (w527:u16)
                n240 = call "Read_only_Manipulator.vi"("Print?"=TRUE, "Motor"=w527, "error in (no error)"=w532, "Command"=Set_Parameter."Error Value (ER)", "VISA resource name"=w533) -> ("error out"=w528:errorcluster, "Transmitted String"=w526:string, "VISA ressource out"=w529:refnum<visa-resource-name>)  [unwired: 3 in, 1 out]
                n241 = property on="Transmitted String" class="Str"("Text.Text"=w526) -> ()  [unwired: 2 in, 2 out]
              }
              event "Reset Error": Value Change {
                n242 = event-data() -> ()  [unwired: 1 in, 6 out]
                n243 = local read "Motor"() -> (w535:u16)
                n244 = call "Read_only_Manipulator.vi"("Motor"=w535, "error in (no error)"=w539, "Command"=Set_Parameter."Reset Error(\\03)", "VISA resource name"=w540) -> ("error out"=w538:errorcluster, "Transmitted String"=w534:string, "VISA ressource out"=w537:refnum<visa-resource-name>)  [unwired: 4 in, 1 out]
                n245 = property on="Transmitted String" class="Str"("Text.Text"=w534) -> ()  [unwired: 2 in, 2 out]
              }
              event "Clear Answer": Value Change {
                n246 = event-data() -> ()  [unwired: 1 in, 6 out]
                n247 = property on="Answer" class="Str"("Text.Text"="") -> ()  [unwired: 2 in, 2 out]
              }
              event "move up", "move down": Value Change {
                w561 = u16 3 items=["none", "1", "2", "3", "4", "all"] ("Motor")
                n248 = event-data() -> ()  [unwired: 1 in, 6 out]
                n249 = property on="Speed" class="DigNum (strict)"() -> ("Value"=w558:dbl)  [unwired: 2 in, 2 out]
                n250 = property on="Def Speed" class="Bool (strict)"() -> ("Value"=w557:bool)  [unwired: 2 in, 2 out]
                n251 = case shown="True" w557 {
                  tunnel: w558 -> [w586 _]
                  tunnel: [w579 w593] -> w553
                  tunnel: w559 -> [w585 w589]
                  tunnel: w560 -> [w584 w597]
                  tunnel: [w583 w596] -> w550
                  tunnel: [w582 w595] -> w551
                  tunnel: w561 -> [w579 w593]
                  tunnel: [w578 w591] -> w555
                  frame True {
                    n252 = call "Conversion_Simple.vi"("Motor"=w579, "Output Unit"=Unit_Control."Microsteps [TMC]" ("Input Unit"), "Input Unit"=Unit_Control."Micron", "Input"=w586) -> (2:"Output"=w580:string, 3:"Output"=w578:dbl)  [unwired: 6 in]
                    n253 = call "Read_only_Manipulator.vi"("Motor"=w579, "error in (no error)"=w584, "Value"=w580, "Command"=Set_Parameter."Velocity Maximum (VM)", "VISA resource name"=w585) -> ("error out"=w583:errorcluster, "VISA ressource out"=w582:refnum<visa-resource-name>)  [unwired: 3 in, 2 out]
                  }
                  frame False {
                    w591 = 15000.0 ("Output")
                    n254 = To Long Integer(number=w591) -> (32bit integer=w590:i32)
                    n255 = Number To Decimal String(number=w590) -> (decimal integer string=w592:string)  [unwired: 1 in]
                    n256 = call "Read_only_Manipulator.vi"("Motor"=w593, "error in (no error)"=w597, "Value"=w592, "Command"=Set_Parameter."Velocity Maximum (VM)", "VISA resource name"=w589) -> ("error out"=w596:errorcluster, "VISA ressource out"=w595:refnum<visa-resource-name>)  [unwired: 3 in, 2 out]
                  }
                }
                n257 = case shown="True" "move down" {
                  tunnel: ["-" "+"] -> w567
                  tunnel: [-1.0 1.0] -> w562
                  frame False {
                  }
                  frame True {
                  }
                }
                n258 = case shown="2" "Unit of Move" {
                  tunnel: "Rel Steps" -> [w660 w667 w674 w681 w688]
                  tunnel: [w660 w666 w673 w680 w687] -> w564
                  tunnel: w553 -> [_ w668 w675 w682 w689]
                  tunnel: [w659 w662 w669 w676 w683] -> w554
                  frame 0, Default {
                    n259 = Scan Value(string=w660, format string="%.6f") -> (value=w659:dbl)  [unwired: 1 in, 1 out]
                  }
                  frame 1 {
                    n260 = call "Conversion_Simple.vi"("Input = DBL/String (DBL[false])"=TRUE, "Motor"=w668, "Output Unit"=Unit_Control."Microsteps [TMC]" ("Input Unit"), "Input Unit"=Unit_Control."Micron", "Input String"=w667) -> (2:"Output"=w666:string, 3:"Output"=w662:dbl)  [unwired: 5 in]
                  }
                  frame 2 {
                    n261 = call "Conversion_Simple.vi"("Input = DBL/String (DBL[false])"=TRUE, "Motor"=w675, "Output Unit"=Unit_Control."Microsteps [TMC]" ("Input Unit"), "Input Unit"=Unit_Control."Millimeter", "Input String"=w674) -> (2:"Output"=w673:string, 3:"Output"=w669:dbl)  [unwired: 5 in]
                  }
                  frame 3 {
                    n262 = call "Conversion_Simple.vi"("Input = DBL/String (DBL[false])"=TRUE, "Motor"=w682, "Output Unit"=Unit_Control."Microsteps [TMC]" ("Input Unit"), "Input Unit"=Unit_Control."Centimeter", "Input String"=w681) -> (2:"Output"=w680:string, 3:"Output"=w676:dbl)  [unwired: 5 in]
                  }
                  frame 4 {
                    n263 = call "Conversion_Simple.vi"("Input = DBL/String (DBL[false])"=TRUE, "Motor"=w689, "Output Unit"=Unit_Control."Microsteps [TMC]" ("Input Unit"), "Input Unit"=Unit_Control."Inches", "Input String"=w688) -> (2:"Output"=w687:string, 3:"Output"=w683:dbl)  [unwired: 5 in]
                  }
                }
                n264 = property on="Z tilt (degrees)" class="DigNum (strict)"() -> ("Value"=w556:dbl)  [unwired: 2 in, 2 out]
                n265 = Concatenate Strings(w567, w564) -> (w568:string)
                n266 = case shown="True" "Z tilt comp" {
                  tunnel: w551 -> [w598 w625]
                  tunnel: w550 -> [w599 w626]
                  tunnel: [w604 w629] -> w549
                  tunnel: [w603 w628] -> w545
                  tunnel: w568 -> [w602 w606]
                  tunnel: w553 -> [w600 w636]
                  tunnel: w554 -> [_ w637]
                  tunnel: w556 -> [_ w632]
                  tunnel: w562 -> [_ w644]
                  tunnel: w555 -> [_ w630]
                  tunnel: w552 -> [_ _]
                  frame False {
                    n267 = call "Read_only_Manipulator.vi"("Motor"=w600, "error in (no error)"=w599, "Value"=w602, "Command"=Set_Parameter."Move Relative (MR)", "VISA resource name"=w598) -> ("error out"=w604:errorcluster, "VISA ressource out"=w603:refnum<visa-resource-name>)  [unwired: 3 in, 2 out]
                  }
                  frame True {
                    w607 = 6.0
                    w639 = Set_Parameter."Move Relative (MR)" ("Command")
                    w618 = u16 2 items=["none", "1", "2", "3", "4", "all"] ("Motor")
                    # "This is the ratio of\nlength per step for\nmotors 3 and 2."
                    n268 = To Long Integer(number=w637) -> (32bit integer=w616:i32)
                    n269 = Negate(x=w632) -> (-x=w646:dbl)
                    n270 = Sign(1:w646) -> (0:w645:dbl)
                    n271 = Multiply(x=w645, y=w644) -> (x*y=w643:dbl)
                    n272 = call "Conversion_Simple.vi"("Output Unit"=Unit_Control."Rad", "Input Unit"=Unit_Control."Angle (Degrees)", "Input"=w632) -> ("Output"=w647:dbl)  [unwired: 7 in, 1 out]
                    n273 = To Long Integer(number=w643) -> (32bit integer=w642:i32)
                    n274 = Tangent(1:w647) -> (0:w631:dbl)
                    n275 = case shown="0, Default" w642 {
                      tunnel: ["-" "0" "+"] -> w638
                      frame -1 {
                      }
                      frame 0, Default {
                      }
                      frame 1 {
                      }
                    }
                    n276 = Multiply(x=w631, y=w616) -> (x*y=w615:dbl)
                    n277 = Multiply(x=w631, y=w630) -> (x*y=w613:dbl)
                    n278 = Multiply(x=w607, y=w613) -> (x*y=w612:dbl)
                    n279 = Multiply(x=w607, y=w615) -> (x*y=w614:dbl)
                    n280 = To Long Integer(number=w612) -> (32bit integer=w611:i32)
                    n281 = To Long Integer(number=w614) -> (32bit integer=w609:i32)
                    n282 = Absolute Value(x=w611) -> (abs(x)=w610:i32)
                    n283 = Absolute Value(x=w609) -> (abs(x)=w608:i32)
                    n284 = Number To Decimal String(number=w610) -> (decimal integer string=w623:string)  [unwired: 1 in]
                    n285 = Number To Decimal String(number=w608) -> (decimal integer string=w627:string)  [unwired: 1 in]
                    n286 = Concatenate Strings(w638, w627) -> (w635:string)
                    n287 = call "Read_only_Manipulator.vi"("Motor"=w618, "error in (no error)"=w626, "Value"=w623, "Command"=Set_Parameter."Velocity Maximum (VM)", "VISA resource name"=w625) -> ("error out"=w621:errorcluster, "VISA ressource out"=w622:refnum<visa-resource-name>)  [unwired: 3 in, 2 out]
                    n288 = stacked-sequence {
                      tunnel: w636 -> [w653]
                      tunnel: w635 -> [w655]
                      tunnel: [w653] -> w634
                      tunnel: [w655] -> w633
                      tunnel: w622 -> [w652]
                      tunnel: w621 -> [w651]
                      tunnel: [w651] -> w620
                      tunnel: [w652] -> w619
                      tunnel: w618 -> [w654]
                      tunnel: [w654] -> w617
                      tunnel: w606 -> [w650]
                      tunnel: [w650] -> w605
                      frame #0 {
                      }
                    }
                    n289 = call "Read_only_Manipulator.vi"("Motor"=w634, "error in (no error)"=w620, "Value"=w605, "Command"=w639, "VISA resource name"=w619) -> ("error out"=w640:errorcluster, "VISA ressource out"=w641:refnum<visa-resource-name>)  [unwired: 3 in, 2 out]
                    n290 = call "Read_only_Manipulator.vi"("Motor"=w617, "error in (no error)"=w640, "Value"=w633, "Command"=w639, "VISA resource name"=w641) -> ("error out"=w629:errorcluster, "VISA ressource out"=w628:refnum<visa-resource-name>)  [unwired: 3 in, 2 out]
                  }
                }
                n291 = local read "Sample\nScan"() -> (w542:bool)
                n292 = case shown="False" TRUE {
                  tunnel: w542 -> [_ _]
                  frame False {
                    n293 = property on="Reset V_max" class="Bool (strict)"("Val(Sgnl)"=TRUE) -> ()  [unwired: 2 in, 2 out]
                  }
                  frame True {
                  }
                }
                n294 = case shown="True" "move down" {
                  tunnel: w549 -> [w573 w577]
                  tunnel: [w572 w576] -> w548
                  tunnel: FALSE ("Input = DBL/String (DBL[false])") -> [w571 w575]
                  tunnel: w545 -> [w570 w574]
                  tunnel: [w570 w574] -> w544
                  frame False {
                    n295 = property on="move up" class="Bool (strict)"(error in=w573, "Value"=w571) -> (error out=w572:errorcluster)  [unwired: 1 in, 1 out]
                  }
                  frame True {
                    n296 = property on="move down" class="Bool (strict)"(error in=w577, "Value"=w575) -> (error out=w576:errorcluster)  [unwired: 1 in, 1 out]
                  }
                }
              }
              event "up M3- TEST", "down M3+ TEST": Value Change {
                w716 = u16 3 items=["none", "1", "2", "3", "4", "all"] ("Motor")
                n297 = event-data() -> ()  [unwired: 1 in, 6 out]
                n298 = property on="Speed" class="DigNum (strict)"() -> ("Value"=w713:dbl)  [unwired: 2 in, 2 out]
                n299 = property on="Def Speed" class="Bool (strict)"() -> ("Value"=w712:bool)  [unwired: 2 in, 2 out]
                n300 = property on="Rel Steps" class="Str"() -> ("Value"=w697:string)  [unwired: 2 in, 2 out]
                n301 = property on="Unit of Move" class="Ring (strict)"() -> ("Value"=w696:T8)  [unwired: 2 in, 2 out]
                n302 = case shown="True" w712 {
                  tunnel: w713 -> [w738 _]
                  tunnel: [w731 w745] -> w694
                  tunnel: w714 -> [w737 w741]
                  tunnel: w715 -> [w736 w749]
                  tunnel: [w735 w748] -> w706
                  tunnel: [w734 w747] -> w707
                  tunnel: w716 -> [w731 w745]
                  tunnel: [w730 w743] -> w710
                  frame True {
                    n303 = call "Conversion_Simple.vi"("Motor"=w731, "Output Unit"=Unit_Control."Microsteps [TMC]" ("Input Unit"), "Input Unit"=Unit_Control."Micron", "Input"=w738) -> (2:"Output"=w732:string, 3:"Output"=w730:dbl)  [unwired: 6 in]
                    n304 = call "Read_only_Manipulator.vi"("Motor"=w731, "error in (no error)"=w736, "Value"=w732, "Command"=Set_Parameter."Velocity Maximum (VM)", "VISA resource name"=w737) -> ("error out"=w735:errorcluster, "VISA ressource out"=w734:refnum<visa-resource-name>)  [unwired: 3 in, 2 out]
                  }
                  frame False {
                    w743 = 15000.0 ("Output")
                    n305 = To Long Integer(number=w743) -> (32bit integer=w742:i32)
                    n306 = Number To Decimal String(number=w742) -> (decimal integer string=w744:string)  [unwired: 1 in]
                    n307 = call "Read_only_Manipulator.vi"("Motor"=w745, "error in (no error)"=w749, "Value"=w744, "Command"=Set_Parameter."Velocity Maximum (VM)", "VISA resource name"=w741) -> ("error out"=w748:errorcluster, "VISA ressource out"=w747:refnum<visa-resource-name>)  [unwired: 3 in, 2 out]
                  }
                }
                n308 = case shown="True" "down M3+ TEST" {
                  tunnel: ["-" "+"] -> w719
                  tunnel: [-1.0 1.0] -> w717
                  frame False {
                  }
                  frame True {
                  }
                }
                n309 = case shown="2" w696 {
                  tunnel: w697 -> [w831 w838 w845 w852 w859]
                  tunnel: [w831 w837 w844 w851 w858] -> w718
                  tunnel: w694 -> [_ w839 w846 w853 w860]
                  tunnel: [w830 w833 w840 w847 w854] -> w709
                  frame 0, Default {
                    n310 = Scan Value(string=w831, format string="%.6f") -> (value=w830:dbl)  [unwired: 1 in, 1 out]
                  }
                  frame 1 {
                    n311 = call "Conversion_Simple.vi"("Input = DBL/String (DBL[false])"=TRUE, "Motor"=w839, "Output Unit"=Unit_Control."Microsteps [TMC]" ("Input Unit"), "Input Unit"=Unit_Control."Micron", "Input String"=w838) -> (2:"Output"=w837:string, 3:"Output"=w833:dbl)  [unwired: 5 in]
                  }
                  frame 2 {
                    n312 = call "Conversion_Simple.vi"("Input = DBL/String (DBL[false])"=TRUE, "Motor"=w846, "Output Unit"=Unit_Control."Microsteps [TMC]" ("Input Unit"), "Input Unit"=Unit_Control."Millimeter", "Input String"=w845) -> (2:"Output"=w844:string, 3:"Output"=w840:dbl)  [unwired: 5 in]
                  }
                  frame 3 {
                    n313 = call "Conversion_Simple.vi"("Input = DBL/String (DBL[false])"=TRUE, "Motor"=w853, "Output Unit"=Unit_Control."Microsteps [TMC]" ("Input Unit"), "Input Unit"=Unit_Control."Centimeter", "Input String"=w852) -> (2:"Output"=w851:string, 3:"Output"=w847:dbl)  [unwired: 5 in]
                  }
                  frame 4 {
                    n314 = call "Conversion_Simple.vi"("Input = DBL/String (DBL[false])"=TRUE, "Motor"=w860, "Output Unit"=Unit_Control."Microsteps [TMC]" ("Input Unit"), "Input Unit"=Unit_Control."Inches", "Input String"=w859) -> (2:"Output"=w858:string, 3:"Output"=w854:dbl)  [unwired: 5 in]
                  }
                }
                n315 = property on="Z tilt comp" class="Bool (strict)"() -> ("Value"=w695:bool)  [unwired: 2 in, 2 out]
                n316 = property on="Z tilt (degrees)" class="DigNum (strict)"() -> ("Value"=w711:dbl)  [unwired: 2 in, 2 out]
                n317 = Concatenate Strings(w719, w718) -> (w720:string)
                n318 = case shown="True" w695 {
                  tunnel: w707 -> [w750 w776]
                  tunnel: w706 -> [w751 w778]
                  tunnel: [w756 w786] -> w705
                  tunnel: [w755 w788] -> w702
                  tunnel: w720 -> [w754 w791]
                  tunnel: w694 -> [w752 w807]
                  tunnel: w709 -> [_ w808]
                  tunnel: w711 -> [_ w803]
                  tunnel: w717 -> [_ w813]
                  tunnel: w710 -> [_ w801]
                  tunnel: w708 -> [_ _]
                  frame False {
                    n319 = call "Read_only_Manipulator.vi"("Motor"=w752, "error in (no error)"=w751, "Value"=w754, "Command"=Set_Parameter."Move Relative (MR)", "VISA resource name"=w750) -> ("error out"=w756:errorcluster, "VISA ressource out"=w755:refnum<visa-resource-name>)  [unwired: 3 in, 2 out]
                  }
                  frame True {
                    w759 = TRUE ("abs?")
                    w765 = FALSE ("abs?")
                    w783 = u16 4 items=["none", "1", "2", "3", "4", "all"] ("Motor")
                    w773 = u16 1 items=["none", "1", "2", "3", "4", "all"] ("Motor")
                    w792 = 6.0
                    w772 = Set_Parameter."Velocity Maximum (VM)" ("Command")
                    w771 = Set_Parameter."Move Relative (MR)" ("Command")
                    w774 = u16 2 items=["none", "1", "2", "3", "4", "all"] ("Motor")
                    # "3"
                    # "2"
                    # "1"
                    # "tan(in-plain angle)"
                    # "This is the ratio of\nlength per step for\nmotors 3 and 2."
                    n320 = To Long Integer(number=w808) -> (32bit integer=w795:i32)
                    n321 = local read "Pos 4 (Steps)"() -> (w781:i32)
                    n322 = Negate(x=w803) -> (-x=w815:dbl)
                    n323 = Sign(1:w815) -> (0:w814:dbl)
                    n324 = Multiply(x=w814, y=w813) -> (x*y=w812:dbl)
                    n325 = call "Conversion_Simple.vi"("Input = DBL/String (DBL[false])"=FALSE ("DBL/String (DBL[false])"), "Motor"=w783, "Output Unit"=Unit_Control."Rad" ("Input Unit"), "Input Unit"=Unit_Control."Angle [TMC]", "Input"=w781) -> ("Output"=w784:dbl)  [unwired: 5 in, 1 out]
                    n326 = call "Conversion_Simple.vi"("Output Unit"=Unit_Control."Rad", "Input Unit"=Unit_Control."Angle (Degrees)", "Input"=w803) -> ("Output"=w816:dbl)  [unwired: 7 in, 1 out]
                    n327 = To Long Integer(number=w812) -> (32bit integer=w811:i32)
                    n328 = Tangent(1:w784) -> (0:w761:dbl)
                    n329 = Tangent(1:w816) -> (0:w802:dbl)
                    n330 = case shown="0, Default" w811 {
                      tunnel: ["-" "0" "+"] -> w768
                      frame -1 {
                      }
                      frame 0, Default {
                      }
                      frame 1 {
                      }
                    }
                    n331 = Multiply(x=w802, y=w801) -> (x*y=w793:dbl)
                    n332 = Multiply(x=w802, y=w795) -> (x*y=w794:dbl)
                    n333 = Multiply(x=w792, y=w793) -> (x*y=w757:dbl)
                    n334 = Multiply(x=w792, y=w794) -> (x*y=w766:dbl)
                    n335 = Divide(x=w766, y=w761) -> (x/y=w767:dbl)
                    n336 = Divide(x=w757, y=w761) -> (x/y=w760:dbl)
                    n337 = call "Round_DBL_to_String.vi"("Double"=w767, "abs?"=w765) -> ("String"=w764:string)
                    n338 = call "Round_DBL_to_String.vi"("Double"=w766, "abs?"=w765) -> ("String"=w770:string)
                    n339 = call "Round_DBL_to_String.vi"("Double"=w760, "abs?"=w759) -> ("String"=w758:string)
                    n340 = call "Round_DBL_to_String.vi"("Double"=w757, "abs?"=w759) -> ("String"=w769:string)
                    n341 = call "Read_only_Manipulator.vi"("Motor"=w774, "error in (no error)"=w778, "Value"=w769, "Command"=w772, "VISA resource name"=w776) -> ("error out"=w777:errorcluster, "VISA ressource out"=w775:refnum<visa-resource-name>)  [unwired: 3 in, 2 out]
                    n342 = Concatenate Strings(w768, w764) -> (w763:string)
                    n343 = Concatenate Strings(w768, w770) -> (w806:string)
                    n344 = call "Read_only_Manipulator.vi"("Motor"=w773, "error in (no error)"=w777, "Value"=w758, "Command"=w772, "VISA resource name"=w775) -> ("error out"=w799:errorcluster, "VISA ressource out"=w800:refnum<visa-resource-name>)  [unwired: 3 in, 2 out]
                    n345 = stacked-sequence {
                      tunnel: w807 -> [w824]
                      tunnel: w806 -> [w826]
                      tunnel: [w824] -> w805
                      tunnel: [w826] -> w804
                      tunnel: w800 -> [w823]
                      tunnel: w799 -> [w822]
                      tunnel: [w822] -> w798
                      tunnel: [w823] -> w797
                      tunnel: w774 -> [w825]
                      tunnel: [w825] -> w796
                      tunnel: w791 -> [w821]
                      tunnel: [w821] -> w790
                      tunnel: [w820] -> w785
                      tunnel: w773 -> [w820]
                      tunnel: [w819] -> w762
                      tunnel: w763 -> [w819]
                      frame #0 {
                      }
                    }
                    n346 = call "Read_only_Manipulator.vi"("Motor"=w805, "error in (no error)"=w798, "Value"=w790, "Command"=w771, "VISA resource name"=w797) -> ("error out"=w809:errorcluster, "VISA ressource out"=w810:refnum<visa-resource-name>)  [unwired: 3 in, 2 out]
                    n347 = call "Read_only_Manipulator.vi"("Motor"=w796, "error in (no error)"=w809, "Value"=w804, "Command"=w771, "VISA resource name"=w810) -> ("error out"=w787:errorcluster, "VISA ressource out"=w789:refnum<visa-resource-name>)  [unwired: 3 in, 2 out]
                    n348 = call "Read_only_Manipulator.vi"("Motor"=w785, "error in (no error)"=w787, "Value"=w762, "Command"=w771, "VISA resource name"=w789) -> ("error out"=w786:errorcluster, "VISA ressource out"=w788:refnum<visa-resource-name>)  [unwired: 3 in, 2 out]
                  }
                }
                n349 = local read "Sample\nScan"() -> (w699:bool)
                n350 = case shown="False" TRUE {
                  tunnel: w699 -> [_ _]
                  frame False {
                    n351 = property on="Reset V_max" class="Bool (strict)"("Val(Sgnl)"=TRUE) -> ()  [unwired: 2 in, 2 out]
                  }
                  frame True {
                  }
                }
                n352 = case shown="False" "down M3+ TEST" {
                  tunnel: w705 -> [w724 w728]
                  tunnel: [w723 w727] -> w704
                  tunnel: FALSE ("Input = DBL/String (DBL[false])") -> [w722 w726]
                  tunnel: w702 -> [w725 w729]
                  tunnel: [w725 w729] -> w701
                  frame False {
                    n353 = property on="up M3- TEST" class="Bool (strict)"(error in=w724, "Value"=w722) -> (error out=w723:errorcluster)  [unwired: 1 in, 1 out]
                  }
                  frame True {
                    n354 = property on="down M3+ TEST" class="Bool (strict)"(error in=w728, "Value"=w726) -> (error out=w727:errorcluster)  [unwired: 1 in, 1 out]
                  }
                }
              }
              event "move to x-rays", "move away x-rays": Value Change {
                w877 = u16 2 items=["none", "1", "2", "3", "4", "all"] ("Motor")
                n355 = event-data() -> ()  [unwired: 1 in, 6 out]
                n356 = property on="Speed" class="DigNum (strict)"() -> ("Value"=w876:dbl)  [unwired: 2 in, 2 out]
                n357 = property on="Def Speed" class="Bool (strict)"() -> ("Value"=w875:bool)  [unwired: 2 in, 2 out]
                n358 = property on="Unit of Move" class="Ring (strict)"() -> ("Value"=w879:u16)  [unwired: 2 in, 2 out]
                n359 = case shown="True" w875 {
                  tunnel: w876 -> [_ w900]
                  tunnel: [w892 w903] -> w878
                  tunnel: w874 -> [w890 w909]
                  tunnel: w873 -> [w894 w908]
                  tunnel: [w893 w907] -> w871
                  tunnel: [w891 w906] -> w872
                  tunnel: w877 -> [w892 w903]
                  frame False {
                    n360 = To Long Integer(number=15000.0 ("Output")) -> (32bit integer=w895:i32)
                    n361 = Number To Decimal String(number=w895) -> (decimal integer string=w897:string)  [unwired: 1 in]
                    n362 = call "Read_only_Manipulator.vi"("Motor"=w892, "error in (no error)"=w894, "Value"=w897, "Command"=Set_Parameter."Velocity Maximum (VM)", "VISA resource name"=w890) -> ("error out"=w893:errorcluster, "VISA ressource out"=w891:refnum<visa-resource-name>)  [unwired: 3 in, 2 out]
                  }
                  frame True {
                    n363 = In Range and Coerce(upper limit=250.0, x=w900, lower limit=0.0) -> (coerced(x)=w899:dbl)  [unwired: 1 out]
                    n364 = call "Conversion_Simple.vi"("Motor"=w903, "Output Unit"=Unit_Control."Microsteps [TMC]" ("Input Unit"), "Input Unit"=Unit_Control."Micron", "Input"=w899) -> ("Output"=w904:string)  [unwired: 6 in, 1 out]
                    n365 = call "Read_only_Manipulator.vi"("Motor"=w903, "error in (no error)"=w908, "Value"=w904, "Command"=Set_Parameter."Velocity Maximum (VM)", "VISA resource name"=w909) -> ("error out"=w907:errorcluster, "VISA ressource out"=w906:refnum<visa-resource-name>)  [unwired: 3 in, 2 out]
                  }
                }
                n366 = case shown="True" "move away x-rays" {
                  tunnel: ["-" "+"] -> w883
                  frame False {
                  }
                  frame True {
                  }
                }
                n367 = property on="Rel Steps" class="Str"() -> ("Text.Text"=w881:string)  [unwired: 2 in, 2 out]
                n368 = case shown="1" w879 {
                  tunnel: w881 -> [w912 w917 w923 w929 w935]
                  tunnel: [w912 w915 w921 w927 w933] -> w880
                  tunnel: w878 -> [_ w918 w924 w930 w936]
                  frame 0, Default {
                  }
                  frame 1 {
                    n369 = call "Conversion_Simple.vi"("Input = DBL/String (DBL[false])"=TRUE ("DBL/String (DBL[false])"), "Motor"=w918, "Output Unit"=Unit_Control."Microsteps [TMC]" ("Input Unit"), "Input Unit"=Unit_Control."Micron", "Input String"=w917) -> ("Output"=w915:string)  [unwired: 5 in, 1 out]
                  }
                  frame 2 {
                    n370 = call "Conversion_Simple.vi"("Input = DBL/String (DBL[false])"=TRUE ("DBL/String (DBL[false])"), "Motor"=w924, "Output Unit"=Unit_Control."Microsteps [TMC]" ("Input Unit"), "Input Unit"=Unit_Control."Millimeter", "Input String"=w923) -> ("Output"=w921:string)  [unwired: 5 in, 1 out]
                  }
                  frame 3 {
                    n371 = call "Conversion_Simple.vi"("Input = DBL/String (DBL[false])"=TRUE ("DBL/String (DBL[false])"), "Motor"=w930, "Output Unit"=Unit_Control."Microsteps [TMC]" ("Input Unit"), "Input Unit"=Unit_Control."Centimeter", "Input String"=w929) -> ("Output"=w927:string)  [unwired: 5 in, 1 out]
                  }
                  frame 4 {
                    n372 = call "Conversion_Simple.vi"("Input = DBL/String (DBL[false])"=TRUE ("DBL/String (DBL[false])"), "Motor"=w936, "Output Unit"=Unit_Control."Microsteps [TMC]" ("Input Unit"), "Input Unit"=Unit_Control."Inches", "Input String"=w935) -> ("Output"=w933:string)  [unwired: 5 in, 1 out]
                  }
                }
                n373 = Concatenate Strings(w883, w880) -> (w882:string)
                n374 = call "Read_only_Manipulator.vi"("Motor"=w878, "error in (no error)"=w871, "Value"=w882, "Command"=Set_Parameter."Move Relative (MR)", "VISA resource name"=w872) -> ("error out"=w868:errorcluster, "VISA ressource out"=w870:refnum<visa-resource-name>)  [unwired: 3 in, 2 out]
                n375 = local read "Sample\nScan"() -> (w869:bool)
                n376 = case shown="False" w869 {
                  frame False {
                    n377 = property on="Reset V_max" class="Bool (strict)"("Val(Sgnl)"=TRUE) -> ()  [unwired: 2 in, 2 out]
                  }
                  frame True {
                  }
                }
                n378 = case shown="True" "move away x-rays" {
                  tunnel: w868 -> [w886 w888]
                  tunnel: [w886 w888] -> w867
                  tunnel: FALSE -> [w885 w887]
                  frame False {
                    n379 = property on="move to x-rays" class="Bool (strict)"("Value"=w885) -> ()  [unwired: 2 in, 2 out]
                  }
                  frame True {
                    n380 = property on="move away x-rays" class="Bool (strict)"("Value"=w887) -> ()  [unwired: 2 in, 2 out]
                  }
                }
              }
              event "move counterclockwise", "move clockwise": Value Change {
                w949 = u16 4 items=["none", "1", "2", "3", "4", "all"] ("Motor")
                n381 = event-data() -> ()  [unwired: 1 in, 6 out]
                n382 = property on="Speed" class="DigNum (strict)"() -> ("Value"=w947:dbl)  [unwired: 2 in, 2 out]
                n383 = property on="Def Speed" class="Bool (strict)"() -> ("Value"=w948:bool)  [unwired: 2 in, 2 out]
                n384 = case shown="True" "move counterclockwise" {
                  tunnel: ["-" "+"] -> w957
                  frame False {
                  }
                  frame True {
                  }
                }
                n385 = property on="Rel Steps" class="Str"() -> ("Text.Text"=w954:string)  [unwired: 2 in, 2 out]
                n386 = property on="Unit of Move" class="Ring (strict)"() -> ("Value"=w953:u16)  [unwired: 2 in, 2 out]
                n387 = case shown="True" w948 {
                  tunnel: w947 -> [_ w974]
                  tunnel: [w965 w978] -> w946
                  tunnel: w951 -> [w964 w977]
                  tunnel: w950 -> [w967 w983]
                  tunnel: [w968 w982] -> w944
                  tunnel: [w966 w981] -> w945
                  tunnel: w949 -> [w965 w978]
                  frame False {
                    n388 = To Long Integer(number=15000.0 ("Output")) -> (32bit integer=w969:i32)
                    n389 = Number To Decimal String(number=w969) -> (decimal integer string=w971:string)  [unwired: 1 in]
                    n390 = call "Read_only_Manipulator.vi"("Motor"=w965, "error in (no error)"=w967, "Value"=w971, "Command"=Set_Parameter."Velocity Maximum (VM)", "VISA resource name"=w964) -> ("error out"=w968:errorcluster, "VISA ressource out"=w966:refnum<visa-resource-name>)  [unwired: 3 in, 2 out]
                  }
                  frame True {
                    n391 = In Range and Coerce(upper limit=5.2734375, x=w974, lower limit=0.0) -> (coerced(x)=w973:dbl)  [unwired: 1 out]
                    n392 = call "Conversion_Simple.vi"("Motor"=w978, "Output Unit"=Unit_Control."Angle [TMC]" ("Input Unit"), "Input Unit"=Unit_Control."Angle (Degrees)", "Input"=w973) -> ("Output"=w979:string)  [unwired: 6 in, 1 out]
                    n393 = call "Read_only_Manipulator.vi"("Motor"=w978, "error in (no error)"=w983, "Value"=w979, "Command"=Set_Parameter."Velocity Maximum (VM)", "VISA resource name"=w977) -> ("error out"=w982:errorcluster, "VISA ressource out"=w981:refnum<visa-resource-name>)  [unwired: 3 in, 2 out]
                  }
                }
                n394 = case shown="2" w953 {
                  tunnel: w954 -> [w986 w991 w997 w1003 w1009]
                  tunnel: [w986 w989 w995 w1001 w1007] -> w952
                  tunnel: w946 -> [_ w992 w998 w1004 w1010]
                  frame 0, Default {
                  }
                  frame 1 {
                    n395 = call "Conversion_Simple.vi"("Input = DBL/String (DBL[false])"=TRUE ("DBL/String (DBL[false])"), "Motor"=w992, "Output Unit"=Unit_Control."Angle [TMC]" ("Input Unit"), "Input Unit"=Unit_Control."Angle (Degrees)", "Input String"=w991) -> ("Output"=w989:string)  [unwired: 5 in, 1 out]
                  }
                  frame 2 {
                    n396 = call "Conversion_Simple.vi"("Input = DBL/String (DBL[false])"=TRUE ("DBL/String (DBL[false])"), "Motor"=w998, "Output Unit"=Unit_Control."Angle [TMC]" ("Input Unit"), "Input Unit"=Unit_Control."Angle (Degrees)", "Input String"=w997) -> ("Output"=w995:string)  [unwired: 5 in, 1 out]
                  }
                  frame 3 {
                    n397 = call "Conversion_Simple.vi"("Input = DBL/String (DBL[false])"=TRUE ("DBL/String (DBL[false])"), "Motor"=w1004, "Output Unit"=Unit_Control."Angle [TMC]" ("Input Unit"), "Input Unit"=Unit_Control."Angle (Degrees)", "Input String"=w1003) -> ("Output"=w1001:string)  [unwired: 5 in, 1 out]
                  }
                  frame 4 {
                    n398 = call "Conversion_Simple.vi"("Input = DBL/String (DBL[false])"=TRUE ("DBL/String (DBL[false])"), "Motor"=w1010, "Output Unit"=Unit_Control."Angle [TMC]" ("Input Unit"), "Input Unit"=Unit_Control."Angle (Degrees)", "Input String"=w1009) -> ("Output"=w1007:string)  [unwired: 5 in, 1 out]
                  }
                }
                n399 = Concatenate Strings(w957, w952) -> (w958:string)
                n400 = call "Read_only_Manipulator.vi"("Motor"=w946, "error in (no error)"=w944, "Value"=w958, "Command"=Set_Parameter."Move Relative (MR)", "VISA resource name"=w945) -> ("error out"=w941:errorcluster, "VISA ressource out"=w955:refnum<visa-resource-name>)  [unwired: 3 in, 2 out]
                n401 = local read "Sample\nScan"() -> (w943:bool)
                n402 = case shown="False" w943 {
                  frame False {
                    n403 = property on="Reset V_max" class="Bool (strict)"("Val(Sgnl)"=TRUE) -> ()  [unwired: 2 in, 2 out]
                  }
                  frame True {
                  }
                }
                n404 = case shown="False" "move counterclockwise" {
                  tunnel: [w960 w962] -> w942
                  tunnel: w941 -> [w960 w962]
                  tunnel: FALSE -> [w959 w961]
                  frame False {
                    n405 = property on="move clockwise" class="Bool (strict)"("Value"=w959) -> ()  [unwired: 2 in, 2 out]
                  }
                  frame True {
                    n406 = property on="move counterclockwise" class="Bool (strict)"("Value"=w961) -> ()  [unwired: 2 in, 2 out]
                  }
                }
              }
              event "move to detector", "move away detector": Value Change {
                w1020 = u16 1 items=["none", "1", "2", "3", "4", "all"] ("Motor")
                n407 = event-data() -> ()  [unwired: 1 in, 6 out]
                n408 = property on="Speed" class="DigNum (strict)"() -> ("Value"=w1025:dbl)  [unwired: 2 in, 2 out]
                n409 = property on="Def Speed" class="Bool (strict)"() -> ("Value"=w1021:bool)  [unwired: 2 in, 2 out]
                n410 = case shown="True" "move away detector" {
                  tunnel: ["-" "+"] -> w1031
                  frame False {
                  }
                  frame True {
                  }
                }
                n411 = property on="Rel Steps" class="Str"() -> ("Text.Text"=w1028:string)  [unwired: 2 in, 2 out]
                n412 = property on="Unit of Move" class="Ring (strict)"() -> ("Value"=w1026:u16)  [unwired: 2 in, 2 out]
                n413 = case shown="True" w1021 {
                  tunnel: w1025 -> [_ w1047]
                  tunnel: [w1040 w1050] -> w1024
                  tunnel: w1023 -> [w1039 w1056]
                  tunnel: w1022 -> [w1045 w1055]
                  tunnel: [w1045 w1054] -> w1018
                  tunnel: [w1038 w1053] -> w1019
                  tunnel: w1020 -> [w1040 w1050]
                  frame False {
                    n414 = To Long Integer(number=15000.0 ("Output")) -> (32bit integer=w1041:i32)
                    n415 = Number To Decimal String(number=w1041) -> (decimal integer string=w1043:string)  [unwired: 1 in]
                    n416 = call "Read_only_Manipulator.vi"("Motor"=w1040, "Value"=w1043, "Command"=Set_Parameter."Velocity Maximum (VM)", "VISA resource name"=w1039) -> ("VISA ressource out"=w1038:refnum<visa-resource-name>)  [unwired: 4 in, 3 out]
                  }
                  frame True {
                    n417 = In Range and Coerce(upper limit=250.0, x=w1047, lower limit=0.0) -> (coerced(x)=w1046:dbl)  [unwired: 1 out]
                    n418 = call "Conversion_Simple.vi"("Motor"=w1050, "Output Unit"=Unit_Control."Microsteps [TMC]" ("Input Unit"), "Input Unit"=Unit_Control."Micron", "Input"=w1046) -> ("Output"=w1051:string)  [unwired: 6 in, 1 out]
                    n419 = call "Read_only_Manipulator.vi"("Motor"=w1050, "error in (no error)"=w1055, "Value"=w1051, "Command"=Set_Parameter."Velocity Maximum (VM)", "VISA resource name"=w1056) -> ("error out"=w1054:errorcluster, "VISA ressource out"=w1053:refnum<visa-resource-name>)  [unwired: 3 in, 2 out]
                  }
                }
                n420 = case shown="0, Default" w1026 {
                  tunnel: w1028 -> [w1059 w1064 w1070 w1076 w1082]
                  tunnel: [w1059 w1062 w1068 w1074 w1080] -> w1027
                  tunnel: w1024 -> [_ w1065 w1071 w1077 w1083]
                  frame 0, Default {
                  }
                  frame 1 {
                    n421 = call "Conversion_Simple.vi"("Input = DBL/String (DBL[false])"=TRUE ("DBL/String (DBL[false])"), "Motor"=w1065, "Output Unit"=Unit_Control."Microsteps [TMC]" ("Input Unit"), "Input Unit"=Unit_Control."Micron", "Input String"=w1064) -> ("Output"=w1062:string)  [unwired: 5 in, 1 out]
                  }
                  frame 2 {
                    n422 = call "Conversion_Simple.vi"("Input = DBL/String (DBL[false])"=TRUE ("DBL/String (DBL[false])"), "Motor"=w1071, "Output Unit"=Unit_Control."Microsteps [TMC]" ("Input Unit"), "Input Unit"=Unit_Control."Millimeter", "Input String"=w1070) -> ("Output"=w1068:string)  [unwired: 5 in, 1 out]
                  }
                  frame 3 {
                    n423 = call "Conversion_Simple.vi"("Input = DBL/String (DBL[false])"=TRUE ("DBL/String (DBL[false])"), "Motor"=w1077, "Output Unit"=Unit_Control."Microsteps [TMC]" ("Input Unit"), "Input Unit"=Unit_Control."Centimeter", "Input String"=w1076) -> ("Output"=w1074:string)  [unwired: 5 in, 1 out]
                  }
                  frame 4 {
                    n424 = call "Conversion_Simple.vi"("Input = DBL/String (DBL[false])"=TRUE ("DBL/String (DBL[false])"), "Motor"=w1083, "Output Unit"=Unit_Control."Microsteps [TMC]" ("Input Unit"), "Input Unit"=Unit_Control."Inches", "Input String"=w1082) -> ("Output"=w1080:string)  [unwired: 5 in, 1 out]
                  }
                }
                n425 = Concatenate Strings(w1031, w1027) -> (w1032:string)
                n426 = call "Read_only_Manipulator.vi"("Motor"=w1024, "error in (no error)"=w1018, "Value"=w1032, "Command"=Set_Parameter."Move Relative (MR)", "VISA resource name"=w1019) -> ("error out"=w1015:errorcluster, "VISA ressource out"=w1029:refnum<visa-resource-name>)  [unwired: 3 in, 2 out]
                n427 = local read "Sample\nScan"() -> (w1017:bool)
                n428 = case shown="False" w1017 {
                  frame False {
                    n429 = property on="Reset V_max" class="Bool (strict)"("Val(Sgnl)"=TRUE) -> ()  [unwired: 2 in, 2 out]
                  }
                  frame True {
                  }
                }
                n430 = case shown="True" "move away detector" {
                  tunnel: [w1034 w1036] -> w1016
                  tunnel: w1015 -> [w1034 w1036]
                  tunnel: FALSE -> [w1033 w1035]
                  frame False {
                    n431 = property on="move to detector" class="Bool (strict)"("Value"=w1033) -> ()  [unwired: 2 in, 2 out]
                  }
                  frame True {
                    n432 = property on="move away detector" class="Bool (strict)"("Value"=w1035) -> ()  [unwired: 2 in, 2 out]
                  }
                }
              }
              event "move in plain 1", "move in plain 2": Value Change {
                w1090 = u16 1 items=["none", "1", "2", "3", "4", "all"] ("Motor")
                w1120 = u16 1 items=["none", "1", "2", "3", "4", "all"] ("Motor")
                w1119 = u16 2 items=["none", "1", "2", "3", "4", "all"] ("Motor")
                # "for angle between zero and ninty degrees:\n[origin = sample, zero points to detector, ninty away from x-rays ]\nmove in plain 1 = towards detector / away from x-rays\nmove in plain 2 = away from detector / towards x-rays"
                # "Do you need to maintain a constant v_x/v_y during acceleration and deceleration as well?\nThis would mean: Set A and D such that A_x/A_y = v_x/v_y."
                n433 = event-data() -> ()  [unwired: 1 in, 6 out]
                n434 = property on="Rel Steps" class="Str"() -> ("Text.Text"=w1104:string)  [unwired: 2 in, 2 out]
                n435 = property on="Unit of Move" class="Ring (strict)"() -> ("Value"=w1103:u16)  [unwired: 2 in, 2 out]
                n436 = property on="Def Speed" class="Bool (strict)"() -> ("Value"=w1100:bool)  [unwired: 2 in, 2 out]
                n437 = case shown="1" w1103 {
                  tunnel: w1104 -> [w1140 w1146 w1152 w1158 w1164]
                  tunnel: Unit_Control."Microsteps [TMC]" ("Input Unit") -> [_ w1143 w1149 w1155 w1161]
                  tunnel: [w1139 w1142 w1148 w1154 w1160] -> w1102
                  tunnel: w1090 -> [_ w1141 w1147 w1153 w1159]
                  frame 0, Default {
                    n438 = Scan Value(string=w1140, format string="%.6f") -> (value=w1139:dbl)  [unwired: 1 in, 1 out]
                  }
                  frame 1 {
                    n439 = call "Conversion_Simple.vi"("Input = DBL/String (DBL[false])"=TRUE ("DBL/String (DBL[false])"), "Motor"=w1141, "Output Unit"=w1143, "Input Unit"=Unit_Control."Micron", "Input String"=w1146) -> ("Output"=w1142:dbl)  [unwired: 5 in, 1 out]
                  }
                  frame 2 {
                    n440 = call "Conversion_Simple.vi"("Input = DBL/String (DBL[false])"=TRUE ("DBL/String (DBL[false])"), "Motor"=w1147, "Output Unit"=w1149, "Input Unit"=Unit_Control."Millimeter", "Input String"=w1152) -> ("Output"=w1148:dbl)  [unwired: 5 in, 1 out]
                  }
                  frame 3 {
                    n441 = call "Conversion_Simple.vi"("Input = DBL/String (DBL[false])"=TRUE ("DBL/String (DBL[false])"), "Motor"=w1153, "Output Unit"=w1155, "Input Unit"=Unit_Control."Centimeter", "Input String"=w1158) -> ("Output"=w1154:dbl)  [unwired: 5 in, 1 out]
                  }
                  frame 4 {
                    n442 = call "Conversion_Simple.vi"("Input = DBL/String (DBL[false])"=TRUE ("DBL/String (DBL[false])"), "Motor"=w1159, "Output Unit"=w1161, "Input Unit"=Unit_Control."Inches", "Input String"=w1164) -> ("Output"=w1160:dbl)  [unwired: 5 in, 1 out]
                  }
                }
                n443 = case shown="True" w1100 {
                  tunnel: [15000.0 ("Output") w1137] -> w1107
                  tunnel: w1090 -> [_ w1133]
                  frame False {
                  }
                  frame True {
                    n444 = property on="Speed" class="DigNum (strict)"() -> ("Value"=w1134:dbl)  [unwired: 2 in, 2 out]
                    n445 = call "Conversion_Simple.vi"("Motor"=w1133, "Output Unit"=Unit_Control."Microsteps [TMC]" ("Input Unit"), "Input Unit"=Unit_Control."Micron", "Input"=w1134) -> ("Output"=w1137:dbl)  [unwired: 6 in, 1 out]
                  }
                }
                n446 = local read "Hor Angle Offset (degrees)"() -> (w1086:dbl)
                n447 = Not(x=w1100) -> (.not. x?=w1101:bool)
                n448 = call "set_in_plane_move_speeds.vi"("Echo Mode"=w1106, "Use standard V_max (t)"=w1101, "error in (no error)"=w1109, "rotate by (degrees)"=w1086, "V_max total"=w1107, "VISA resource name"=w1110) -> ("error out"=w1099:errorcluster, "V_max Motor 2"=w1087:i32, "V_max Motor 1"=w1111:i32, "VISA ressource out"=w1097:refnum<visa-resource-name>, "Angle Sample Holder"=w1108:dbl)  [unwired: 1 in]
                "V_max Motor 1" <- w1111
                "V_max Motor 2" <- w1087
                n449 = Not(x="move in plain 1") -> (.not. x?=w1118:bool)
                n450 = Divide(x=w1087, y=w1111) -> (x/y=w1117:dbl)
                n451 = call "in plane scan.vi"("invert y"=w1118, "invert x"="move in plain 1", "angle (degrees)"=w1108, "v total"=w1102) -> ("v_y string"=w1121:string, "v_x string"=w1122:string)  [unwired: 2 in, 4 out]
                n452 = Inverse Tangent(1:w1117) -> (0:w1116:dbl)
                n453 = call "wait_milliseconds.vi"("milliseconds to wait"=u32 0, "error in"=w1099) -> ("error out"=w1096:errorcluster)  [unwired: 9 in]
                n454 = call "Conversion_Simple.vi"("Output Unit"=Unit_Control."Angle (Degrees)", "Input Unit"=Unit_Control."Rad", "Input"=w1116) -> ("Output"=→"actual angle":dbl)  [unwired: 7 in, 1 out]
                n455 = case shown="True" TRUE {
                  tunnel: w1122 -> [w1170 w1183]
                  tunnel: w1121 -> [w1167 w1182]
                  tunnel: w1097 -> [w1175 w1181]
                  tunnel: w1120 -> [_ w1180]
                  tunnel: w1119 -> [_ w1179]
                  tunnel: [w1172 w1178] -> w1094
                  tunnel: [w1173 w1176] -> w1095
                  tunnel: w1096 -> [w1174 w1177]
                  frame False {
                    w1166 = "\n"
                    n456 = call <vilib>:"Space Constant.vi"() -> ("String"=w1168:string)
                    n457 = Concatenate Strings("1MR" ("string"), w1168, w1170, w1166, "2MR" ("string"), w1168, w1167, w1166) -> (w1165:string)
                    n458 = VISA Write(VISA resource name=w1175, write buffer=w1165, error in (no error)=w1174) -> (VISA resource name out=w1172:refnum<visa-resource-name>, error out=w1173:errorcluster)  [unwired: 1 out]
                  }
                  frame True {
                    w1184 = Set_Parameter."Move Relative (MR)" ("Command")
                    n459 = call "Read_only_Manipulator.vi"("Motor"=w1180, "error in (no error)"=w1177, "Value"=w1183, "Command"=w1184, "VISA resource name"=w1181) -> ("error out"=w1185:errorcluster, "VISA ressource out"=w1186:refnum<visa-resource-name>)  [unwired: 3 in, 2 out]
                    n460 = call "Read_only_Manipulator.vi"("Motor"=w1179, "error in (no error)"=w1185, "Value"=w1182, "Command"=w1184, "VISA resource name"=w1186) -> ("error out"=w1176:errorcluster, "VISA ressource out"=w1178:refnum<visa-resource-name>)  [unwired: 3 in, 2 out]
                    "steps motor 1 ()" <- w1183
                    "steps motor 2 ()" <- w1182
                  }
                }
                n461 = case shown="True" "move in plain 1" {
                  tunnel: w1095 -> [w1126 w1131]
                  tunnel: [w1125 w1130] -> w1089
                  tunnel: w1094 -> [w1127 w1129]
                  tunnel: [w1127 w1129] -> w1093
                  tunnel: FALSE -> [w1124 w1128]
                  frame False {
                    n462 = property on="move in plain 2" class="Bool (strict)"(error in=w1126, "Value"=w1124) -> (error out=w1125:errorcluster)  [unwired: 1 in, 1 out]
                  }
                  frame True {
                    n463 = property on="move in plain 1" class="Bool (strict)"(error in=w1131, "Value"=w1128) -> (error out=w1130:errorcluster)  [unwired: 1 in, 1 out]
                  }
                }
                n464 = local read "Sample\nScan"() -> (w1088:bool)
                n465 = case shown="False" w1088 {
                  frame False {
                    n466 = property on="Reset V_max" class="Bool (strict)"("Val(Sgnl)"=TRUE) -> ()  [unwired: 2 in, 2 out]
                  }
                  frame True {
                  }
                }
              }
              event "retract XPS", "approach XPS": Value Change {
                w1197 = u16 1 items=["none", "1", "2", "3", "4", "all"] ("Motor")
                w1223 = u16 1 items=["none", "1", "2", "3", "4", "all"] ("Motor")
                w1222 = u16 2 items=["none", "1", "2", "3", "4", "all"] ("Motor")
                # "for angle between zero and ninty degrees:\n[origin = sample, zero points to detector, ninty away from x-rays ]\nmove in plain 1 = towards detector / away from x-rays\nmove in plain 2 = away from detector / towards x-rays"
                n467 = event-data() -> ()  [unwired: 1 in, 6 out]
                n468 = property on="Rel Steps XPS" class="Str"() -> ("Text.Text"=w1209:string)  [unwired: 2 in, 2 out]
                n469 = property on="Def Speed" class="Bool (strict)"() -> ("Value"=w1206:bool)  [unwired: 2 in, 2 out]
                n470 = case shown="1" u16 1 ("Unit of Move") {
                  tunnel: w1209 -> [w1243 w1249 w1255 w1261 w1267]
                  tunnel: Unit_Control."Microsteps [TMC]" ("Input Unit") -> [_ w1246 w1252 w1258 w1264]
                  tunnel: [w1242 w1245 w1251 w1257 w1263] -> w1208
                  tunnel: w1197 -> [_ w1244 w1250 w1256 w1262]
                  frame 0, Default {
                    n471 = Scan Value(string=w1243, format string="%.6f") -> (value=w1242:dbl)  [unwired: 1 in, 1 out]
                  }
                  frame 1 {
                    n472 = call "Conversion_Simple.vi"("Input = DBL/String (DBL[false])"=TRUE ("DBL/String (DBL[false])"), "Motor"=w1244, "Output Unit"=w1246, "Input Unit"=Unit_Control."Micron", "Input String"=w1249) -> ("Output"=w1245:dbl)  [unwired: 5 in, 1 out]
                  }
                  frame 2 {
                    n473 = call "Conversion_Simple.vi"("Input = DBL/String (DBL[false])"=TRUE ("DBL/String (DBL[false])"), "Motor"=w1250, "Output Unit"=w1252, "Input Unit"=Unit_Control."Millimeter", "Input String"=w1255) -> ("Output"=w1251:dbl)  [unwired: 5 in, 1 out]
                  }
                  frame 3 {
                    n474 = call "Conversion_Simple.vi"("Input = DBL/String (DBL[false])"=TRUE ("DBL/String (DBL[false])"), "Motor"=w1256, "Output Unit"=w1258, "Input Unit"=Unit_Control."Centimeter", "Input String"=w1261) -> ("Output"=w1257:dbl)  [unwired: 5 in, 1 out]
                  }
                  frame 4 {
                    n475 = call "Conversion_Simple.vi"("Input = DBL/String (DBL[false])"=TRUE ("DBL/String (DBL[false])"), "Motor"=w1262, "Output Unit"=w1264, "Input Unit"=Unit_Control."Inches", "Input String"=w1267) -> ("Output"=w1263:dbl)  [unwired: 5 in, 1 out]
                  }
                }
                n476 = local read "Hor Angle Offset (degrees)"() -> (w1188:dbl)
                n477 = case shown="True" w1206 {
                  tunnel: [15000.0 ("Output") w1240] -> w1212
                  tunnel: w1197 -> [_ w1236]
                  frame False {
                  }
                  frame True {
                    n478 = property on="Speed" class="DigNum (strict)"() -> ("Value"=w1237:dbl)  [unwired: 2 in, 2 out]
                    n479 = call "Conversion_Simple.vi"("Motor"=w1236, "Output Unit"=Unit_Control."Microsteps [TMC]" ("Input Unit"), "Input Unit"=Unit_Control."Micron", "Input"=w1237) -> ("Output"=w1240:dbl)  [unwired: 6 in, 1 out]
                  }
                }
                n480 = Not(x=w1206) -> (.not. x?=w1207:bool)
                n481 = call "set_in_plane_move_speeds.vi"("Switch X and Y (f)"=TRUE, "Echo Mode"=w1211, "Use standard V_max (t)"=w1207, "error in (no error)"=w1214, "rotate by (degrees)"=w1188, "V_max total"=w1212, "VISA resource name"=w1215) -> ("error out"=w1205:errorcluster, "V_max Motor 2"=w1190:i32, "V_max Motor 1"=w1191:i32, "VISA ressource out"=w1203:refnum<visa-resource-name>, "Angle Sample Holder"=w1213:dbl)
                n482 = Not(x="retract XPS") -> (.not. x?=w1221:bool)
                n483 = Divide(x=w1190, y=w1191) -> (x/y=w1220:dbl)
                n484 = call "in plane scan.vi"("invert y"=w1221, "invert x"="retract XPS", "rotate by (degrees)"=90.0, "angle (degrees)"=w1213, "v total"=w1208) -> ("v_y string"=w1224:string, "v_x string"=w1225:string)  [unwired: 1 in, 4 out]
                n485 = Inverse Tangent(1:w1220) -> (0:w1219:dbl)
                n486 = call "wait_milliseconds.vi"("milliseconds to wait"=u32 0, "error in"=w1205) -> ("error out"=w1202:errorcluster)  [unwired: 9 in]
                n487 = call "Conversion_Simple.vi"("Output Unit"=Unit_Control."Angle (Degrees)", "Input Unit"=Unit_Control."Rad", "Input"=w1219) -> ("Output"=w1192:dbl)  [unwired: 7 in, 1 out]
                n488 = case shown="True" TRUE {
                  tunnel: w1225 -> [w1273 w1280]
                  tunnel: w1224 -> [w1270 w1279]
                  tunnel: w1203 -> [w1278 w1286]
                  tunnel: w1223 -> [_ w1285]
                  tunnel: w1222 -> [_ w1284]
                  tunnel: [w1275 w1283] -> w1200
                  tunnel: [w1276 w1281] -> w1201
                  tunnel: w1202 -> [w1277 w1282]
                  frame False {
                    w1269 = "\n"
                    n489 = call <vilib>:"Space Constant.vi"() -> ("String"=w1271:string)
                    n490 = Concatenate Strings("1MR" ("string"), w1271, w1273, w1269, "2MR" ("string"), w1271, w1270, w1269) -> (w1268:string)
                    n491 = VISA Write(VISA resource name=w1278, write buffer=w1268, error in (no error)=w1277) -> (VISA resource name out=w1275:refnum<visa-resource-name>, error out=w1276:errorcluster)  [unwired: 1 out]
                  }
                  frame True {
                    w1287 = Set_Parameter."Move Relative (MR)" ("Command")
                    n492 = call "Read_only_Manipulator.vi"("Motor"=w1285, "error in (no error)"=w1282, "Value"=w1280, "Command"=w1287, "VISA resource name"=w1286) -> ("error out"=w1288:errorcluster, "VISA ressource out"=w1289:refnum<visa-resource-name>)  [unwired: 3 in, 2 out]
                    n493 = local write "steps motor 2 ()"(w1279) -> ()
                    n494 = local write "steps motor 1 ()"(w1280) -> ()
                    n495 = call "Read_only_Manipulator.vi"("Motor"=w1284, "error in (no error)"=w1288, "Value"=w1279, "Command"=w1287, "VISA resource name"=w1289) -> ("error out"=w1281:errorcluster, "VISA ressource out"=w1283:refnum<visa-resource-name>)  [unwired: 3 in, 2 out]
                  }
                }
                n496 = local write "actual angle"(w1192) -> ()
                n497 = local write "V_max Motor 1"(w1191) -> ()
                n498 = local write "V_max Motor 2"(w1190) -> ()
                n499 = case shown="True" "retract XPS" {
                  tunnel: w1201 -> [w1228 w1233]
                  tunnel: [w1229 w1232] -> w1196
                  tunnel: w1200 -> [w1230 w1234]
                  tunnel: [w1230 w1234] -> w1199
                  tunnel: FALSE -> [w1227 w1231]
                  frame False {
                    n500 = property on="approach XPS" class="Bool (strict)"(error in=w1228, "Value"=w1227) -> (error out=w1229:errorcluster)  [unwired: 1 in, 1 out]
                  }
                  frame True {
                    n501 = property on="retract XPS" class="Bool (strict)"(error in=w1233, "Value"=w1231) -> (error out=w1232:errorcluster)  [unwired: 1 in, 1 out]
                  }
                }
                n502 = local read "Sample\nScan"() -> (w1195:bool)
                n503 = case shown="False" w1195 {
                  frame False {
                    n504 = property on="Reset V_max" class="Bool (strict)"("Val(Sgnl)"=TRUE) -> ()  [unwired: 2 in, 2 out]
                  }
                  frame True {
                  }
                }
              }
              event "up M3- XPS", "down M3+ XPS", "to analyzer M2- XPS", "away analyzer M2+ XPS", "to X-rays M1- XPS", "away X-rays M1+ XPS", "in plain 1 XPS", "in plain 2 XPS": Value Change {
                w1301 = T8 1 items=["STEPS", "MICRONS / DEG", "MILLIMETER / DEG", "CENTIMETER / DEG", "INCHES / DEG"] ("Unit of Move XPS")
                n505 = event-data() -> ()  [unwired: 1 in, 6 out]
                n506 = case shown="True" "up M3- XPS" {
                  selector: "up M3- XPS" -> [_ w1310]
                  frame False {
                  }
                  frame True {
                    n507 = property on="move up" class="Bool (strict)"("Val(Sgnl)"=w1310) -> ()  [unwired: 2 in, 2 out]
                  }
                }
                n508 = case shown="True" "down M3+ XPS" {
                  selector: "down M3+ XPS" -> [_ w1309]
                  frame False {
                  }
                  frame True {
                    n509 = property on="move down" class="Bool (strict)"("Val(Sgnl)"=w1309) -> ()  [unwired: 2 in, 2 out]
                  }
                }
                n510 = case shown="True" "to analyzer M2- XPS" {
                  selector: "to analyzer M2- XPS" -> [_ w1308]
                  frame False {
                  }
                  frame True {
                    n511 = property on="move to x-rays" class="Bool (strict)"("Val(Sgnl)"=w1308) -> ()  [unwired: 2 in, 2 out]
                  }
                }
                n512 = case shown="True" "away analyzer M2+ XPS" {
                  selector: "away analyzer M2+ XPS" -> [_ w1307]
                  frame False {
                  }
                  frame True {
                    n513 = property on="move away x-rays" class="Bool (strict)"("Val(Sgnl)"=w1307) -> ()  [unwired: 2 in, 2 out]
                  }
                }
                n514 = case shown="True" "to X-rays M1- XPS" {
                  selector: "to X-rays M1- XPS" -> [_ w1304]
                  frame False {
                  }
                  frame True {
                    n515 = property on="move to detector" class="Bool (strict)"("Val(Sgnl)"=w1304) -> ()  [unwired: 2 in, 2 out]
                  }
                }
                n516 = case shown="True" "away X-rays M1+ XPS" {
                  selector: "away X-rays M1+ XPS" -> [_ w1303]
                  frame False {
                  }
                  frame True {
                    n517 = property on="move away detector" class="Bool (strict)"("Val(Sgnl)"=w1303) -> ()  [unwired: 2 in, 2 out]
                  }
                }
                n518 = case shown="True" "in plain 1 XPS" {
                  selector: "in plain 1 XPS" -> [_ w1305]
                  frame False {
                  }
                  frame True {
                    n519 = property on="move in plain 1" class="Bool (strict)"("Val(Sgnl)"=w1305) -> ()  [unwired: 2 in, 2 out]
                  }
                }
                n520 = case shown="True" "in plain 2 XPS" {
                  selector: "in plain 2 XPS" -> [_ w1306]
                  frame False {
                  }
                  frame True {
                    n521 = property on="move in plain 2" class="Bool (strict)"("Val(Sgnl)"=w1306) -> ()  [unwired: 2 in, 2 out]
                  }
                }
                n522 = local write "Rel Steps"("Rel Steps XPS") -> ()
                n523 = local write "Unit of Move"(w1301) -> ()
                n524 = local write "Z tilt comp"("Z tilt comp XPS") -> ()
                n525 = property on="Z tilt (x/z)" class="DigNum (strict)"("Val(Sgnl)"="Z tilt (M2/M3) XPS") -> ()  [unwired: 2 in, 2 out]
                n526 = local write "Def Speed"(FALSE ("Def Speed")) -> ()
              }
              event "move counterclockwise XPS", "move clockwise XPS": Value Change {
                w1312 = T8 1 items=["STEPS", "MICRONS / DEG", "MILLIMETER / DEG", "CENTIMETER / DEG", "INCHES / DEG"] ("Unit of Move XPS")
                n527 = event-data() -> ()  [unwired: 1 in, 6 out]
                n528 = case shown="True" "move counterclockwise XPS" {
                  selector: "move counterclockwise XPS" -> [_ w1317]
                  frame False {
                  }
                  frame True {
                    n529 = property on="move counterclockwise" class="Bool (strict)"("Val(Sgnl)"=w1317) -> ()  [unwired: 2 in, 2 out]
                  }
                }
                n530 = case shown="True" "move clockwise XPS" {
                  selector: "move clockwise XPS" -> [_ w1316]
                  frame False {
                  }
                  frame True {
                    n531 = property on="move clockwise" class="Bool (strict)"("Val(Sgnl)"=w1316) -> ()  [unwired: 2 in, 2 out]
                  }
                }
                n532 = local write "Rel Steps"("Rel Deg XPS") -> ()
                n533 = local write "Unit of Move"(w1312) -> ()
                n534 = local write "Def Speed"(FALSE ("Def Speed")) -> ()
              }
              event "scan up M3- XPS", "scan down M3+ XPS", "scan right XPS", "scan left XPS": Value Change {
                w1348 = T8 2 items=["STEPS", "MICRONS / DEG", "MILLIMETER / DEG", "CENTIMETER / DEG", "INCHES / DEG"] ("Unit of Move 4")
                # "in plain: replace\nM1 and M2!"
                n535 = event-data() -> ()  [unwired: 1 in, 6 out]
                n536 = global read "Pressure_Ch_1_2_Manipulator_Pos.vi" "Manipulator Pos steps"() -> (w1321:i32[])
                n537 = Or(x="scan up M3- XPS", y="scan down M3+ XPS") -> (x .or. y?=w1324:bool)
                n538 = case shown="False" w1324 {
                  tunnel: "scan down M3+ XPS" -> [_ w1355]
                  tunnel: "scan up M3- XPS" -> [_ w1354]
                  tunnel: [w1351 w1353] -> w1322
                  tunnel: [0 ("index") 2 ("index")] -> w1318
                  frame False {
                    w1351 = u16 2 items=["none", "1", "2", "3", "4", "all"] ("Motor")
                  }
                  frame True {
                    w1353 = u16 3 items=["none", "1", "2", "3", "4", "all"] ("Motor")
                    n539 = case shown="True" w1354 {
                      selector: w1354 -> [_ w1357]
                      frame False {
                      }
                      frame True {
                        n540 = property on="move up" class="Bool (strict)"("Val(Sgnl)"=w1357) -> ()  [unwired: 2 in, 2 out]
                      }
                    }
                    n541 = case shown="True" w1355 {
                      selector: w1355 -> [_ w1356]
                      frame False {
                      }
                      frame True {
                        n542 = property on="move down" class="Bool (strict)"("Val(Sgnl)"=w1356) -> ()  [unwired: 2 in, 2 out]
                      }
                    }
                  }
                }
                n543 = case shown="True" "scan right XPS" {
                  selector: "scan right XPS" -> [_ w1358]
                  frame False {
                  }
                  frame True {
                    n544 = property on="move in plain 1" class="Bool (strict)"("Val(Sgnl)"=w1358) -> ()  [unwired: 2 in, 2 out]
                  }
                }
                n545 = case shown="True" "scan left XPS" {
                  selector: "scan left XPS" -> [_ w1359]
                  frame False {
                  }
                  frame True {
                    n546 = property on="move in plain 2" class="Bool (strict)"("Val(Sgnl)"=w1359) -> ()  [unwired: 2 in, 2 out]
                  }
                }
                n547 = local read "Z tilt comp XPS"() -> (w1343:bool)
                n548 = local read "Z tilt (M2/M3) XPS"() -> (w1344:dbl)
                n549 = Fract/Exp String To Number(string="Scan Distance XPS") -> (number=w1336:dbl)  [unwired: 3 in, 1 out]
                n550 = Divide(x=w1336, y="XPS Scan Speed [µm/s]") -> (x/y=w1335:dbl)
                n551 = local write "Unit of Move"(w1348) -> ()
                n552 = property on="Def Speed" class="Bool (strict)"("Value"=TRUE ("Def Speed")) -> ()  [unwired: 2 in, 2 out]
                n553 = local write "Z tilt comp"(w1343) -> ()
                n554 = property on="Z tilt (x/z)" class="DigNum (strict)"("Val(Sgnl)"=w1344) -> ()  [unwired: 2 in, 2 out]
                n555 = local write "Rel Steps"("Scan Distance XPS") -> ()
                n556 = property on="Speed" class="DigNum (strict)"("Value"="XPS Scan Speed [µm/s]") -> ()  [unwired: 2 in, 2 out]
                n557 = Multiply(x=w1335, y=1000.0) -> (x*y=w1333:dbl)
                n558 = Get Date/Time In Seconds() -> (seconds since 1Jan1904=w1332:timestamp)
                n559 = Add(x=w1333, y=w1332) -> (x+y=w1331:timestamp)
                n560 = call "Conversion_Simple.vi"("Input = DBL/String (DBL[false])"=TRUE ("DBL/String (DBL[false])"), "Motor"=w1322, "Output Unit"=Unit_Control."Microsteps [TMC]" ("Input Unit"), "Input Unit"=Unit_Control."Millimeter", "Input"="XPS Scan Speed [µm/s]") -> ("Output"=w1320:dbl)  [unwired: 5 in, 1 out]
                n561 = Get Date/Time String(seconds (now)=w1331, want seconds? (F)=TRUE) -> (time string=→"end time":string)  [unwired: 1 in, 1 out]
                n562 = Replace Array Subset(array=w1321, new element=w1320, index=w1318) -> (w1319:i32[])
                n563 = Not(x="Switch Laser") -> (.not. x?=w1346:bool)
                n564 = call "PoD_Laser_ON_OFF.vi"("Enable VI"=w1346, "Laser ON (t) / OFF (f)"=TRUE) -> ("AO switched"=w1342:bool)  [unwired: 9 in]
                n565 = global write "Switch _Laser_Global.vi" "Laser (on, t; off, f)"(w1342) -> ()
                n566 = global write "Global_Next_Scan_Position.vi" "Next Scan Pos"(w1319) -> ()
                n567 = global write "Global_Next_Scan_Position.vi" "XAS(f) / XPS(t)"(TRUE ("XAS(f) / XPS(t)")) -> ()
              }
              event "stop scan XPS": Value Change {
                n568 = event-data() -> ()  [unwired: 1 in, 6 out]
                n569 = property on="emergency stop" class="Bool (strict)"("Val(Sgnl)"=TRUE) -> ()  [unwired: 2 in, 2 out]
                n570 = call "PoD_Laser_ON_OFF.vi"("Enable VI"=TRUE, "Laser ON (t) / OFF (f)"=FALSE) -> ()  [unwired: 9 in, 1 out]
              }
              event "In-Plain subVI Test": Value Change {
                n571 = event-data() -> ()  [unwired: 1 in, 6 out]
                n572 = call "move_in_horizontal_plain.vi"("direction"="direction", "Echo Mode"=w1372, "Unit of Move"="Unit of Move 2", "error in (no error)"=w1373, "Speed [micron/s]"="Speed [micron/s] 2", "Steps"="Steps", "ComPort"=w1374) -> ("error out"=w1364:errorcluster, "move time (ms)"=→"move time (ms) 4":u32, "actual angle"=→"actual angle 2":dbl, "VISA ressource out"=w1371:refnum<visa-resource-name>)  [unwired: 1 in]
                n573 = local read "Sample\nScan"() -> (w1363:bool)
                n574 = case shown="False" w1363 {
                  frame False {
                    n575 = property on="Reset V_max" class="Bool (strict)"("Val(Sgnl)"=TRUE) -> ()  [unwired: 2 in, 2 out]
                  }
                  frame True {
                  }
                }
              }
              event "Pos 1 (Steps)": Value Change {
                w1378 = u16 1 items=["none", "1", "2", "3", "4", "all"] ("Motor")
                n576 = event-data() -> ("OldVal"=w1383:i32, "NewVal"=w1384:i32)  [unwired: 1 in, 4 out]
                n577 = Subtract(x=w1384, y=w1383) -> (x-y=w1379:i32)
                n578 = Number To Decimal String(number=w1379) -> (decimal integer string=w1382:string)  [unwired: 1 in]
                n579 = call "Read_only_Manipulator.vi"("Motor"=w1378, "error in (no error)"=w1376, "Value"=w1382, "Command"=Set_Parameter."Move Relative (MR)", "VISA resource name"=w1377) -> ("error out"=w1381:errorcluster, "VISA ressource out"=w1380:refnum<visa-resource-name>)  [unwired: 3 in, 2 out]
              }
              event "Pos 2 (Steps)": Value Change {
                w1389 = u16 2 items=["none", "1", "2", "3", "4", "all"] ("Motor")
                n580 = event-data() -> ("OldVal"=w1393:i32, "NewVal"=w1394:i32)  [unwired: 1 in, 4 out]
                n581 = Subtract(x=w1394, y=w1393) -> (x-y=w1388:i32)
                n582 = Number To Decimal String(number=w1388) -> (decimal integer string=w1392:string)  [unwired: 1 in]
                n583 = call "Read_only_Manipulator.vi"("Motor"=w1389, "error in (no error)"=w1386, "Value"=w1392, "Command"=Set_Parameter."Move Relative (MR)", "VISA resource name"=w1387) -> ("error out"=w1391:errorcluster, "VISA ressource out"=w1390:refnum<visa-resource-name>)  [unwired: 3 in, 2 out]
              }
              event "Pos 3 (Steps)": Value Change {
                w1405 = u16 3 items=["none", "1", "2", "3", "4", "all"] ("Motor")
                n584 = event-data() -> ("OldVal"=w1406:i32, "NewVal"=w1407:i32)  [unwired: 1 in, 4 out]
                n585 = Subtract(x=w1407, y=w1406) -> (x-y=w1396:i32)
                n586 = property on="Z tilt comp" class="Bool (strict)"() -> ("Value"=w1402:bool)  [unwired: 2 in, 2 out]
                n587 = property on="Z tilt (degrees)" class="DigNum (strict)"() -> ("Value"=w1401:dbl)  [unwired: 2 in, 2 out]
                n588 = Number To Decimal String(number=w1396) -> (decimal integer string=w1404:string)  [unwired: 1 in]
                n589 = case shown="True" w1402 {
                  tunnel: w1400 -> [w1409 w1437]
                  tunnel: w1399 -> [w1408 w1438]
                  tunnel: [w1414 w1441] -> w1397
                  tunnel: [w1413 w1440] -> w1398
                  tunnel: w1404 -> [w1412 w1417]
                  tunnel: w1405 -> [w1410 w1447]
                  tunnel: w1401 -> [_ w1443]
                  tunnel: w1403 -> [_ _]
                  tunnel: w1396 -> [_ w1415]
                  frame False {
                    n590 = call "Read_only_Manipulator.vi"("Motor"=w1410, "error in (no error)"=w1408, "Value"=w1412, "Command"=Set_Parameter."Move Relative (MR)", "VISA resource name"=w1409) -> ("error out"=w1414:errorcluster, "VISA ressource out"=w1413:refnum<visa-resource-name>)  [unwired: 3 in, 2 out]
                  }
                  frame True {
                    w1418 = 6.0
                    w1449 = Set_Parameter."Move Relative (MR)" ("Command")
                    w1430 = u16 2 items=["none", "1", "2", "3", "4", "all"] ("Motor")
                    # "This is the ratio of\nlength per step for\nmotors 3 and 2."
                    n591 = Negate(x=w1443) -> (-x=w1455:dbl)
                    n592 = Sign(1:w1415) -> (0:w1423:i32)
                    n593 = Sign(1:w1455) -> (0:w1454:dbl)
                    n594 = Multiply(x=w1454, y=w1423) -> (x*y=w1453:dbl)
                    n595 = call "Conversion_Simple.vi"("Output Unit"=Unit_Control."Rad", "Input Unit"=Unit_Control."Angle (Degrees)", "Input"=w1443) -> ("Output"=w1456:dbl)  [unwired: 7 in, 1 out]
                    n596 = To Long Integer(number=w1453) -> (32bit integer=w1452:i32)
                    n597 = Tangent(1:w1456) -> (0:w1442:dbl)
                    n598 = case shown="1" w1452 {
                      tunnel: ["-" "0" "+"] -> w1448
                      frame -1 {
                      }
                      frame 0, Default {
                      }
                      frame 1 {
                      }
                    }
                    n599 = Multiply(x=w1442, y=w1415) -> (x*y=w1428:dbl)
                    n600 = Multiply(x=w1442, y=15000.0) -> (x*y=w1426:dbl)
                    n601 = Multiply(x=w1418, y=w1426) -> (x*y=w1425:dbl)
                    n602 = Multiply(x=w1418, y=w1428) -> (x*y=w1427:dbl)
                    n603 = To Long Integer(number=w1425) -> (32bit integer=w1422:i32)
                    n604 = To Long Integer(number=w1427) -> (32bit integer=w1420:i32)
                    n605 = Absolute Value(x=w1422) -> (abs(x)=w1421:i32)
                    n606 = Absolute Value(x=w1420) -> (abs(x)=w1419:i32)
                    n607 = Number To Decimal String(number=w1421) -> (decimal integer string=w1435:string)  [unwired: 1 in]
                    n608 = Number To Decimal String(number=w1419) -> (decimal integer string=w1439:string)  [unwired: 1 in]
                    n609 = Concatenate Strings(w1448, w1439) -> (w1446:string)
                    n610 = call "Read_only_Manipulator.vi"("Motor"=w1430, "error in (no error)"=w1438, "Value"=w1435, "Command"=Set_Parameter."Velocity Maximum (VM)", "VISA resource name"=w1437) -> ("error out"=w1433:errorcluster, "VISA ressource out"=w1434:refnum<visa-resource-name>)  [unwired: 3 in, 2 out]
                    n611 = stacked-sequence {
                      tunnel: w1447 -> [w1462]
                      tunnel: w1446 -> [w1464]
                      tunnel: [w1462] -> w1445
                      tunnel: [w1464] -> w1444
                      tunnel: w1434 -> [w1461]
                      tunnel: w1433 -> [w1460]
                      tunnel: [w1460] -> w1432
                      tunnel: [w1461] -> w1431
                      tunnel: w1430 -> [w1463]
                      tunnel: [w1463] -> w1429
                      tunnel: w1417 -> [w1459]
                      tunnel: [w1459] -> w1416
                      frame #0 {
                      }
                    }
                    n612 = call "Read_only_Manipulator.vi"("Motor"=w1445, "error in (no error)"=w1432, "Value"=w1416, "Command"=w1449, "VISA resource name"=w1431) -> ("error out"=w1450:errorcluster, "VISA ressource out"=w1451:refnum<visa-resource-name>)  [unwired: 3 in, 2 out]
                    n613 = call "Read_only_Manipulator.vi"("Motor"=w1429, "error in (no error)"=w1450, "Value"=w1444, "Command"=w1449, "VISA resource name"=w1451) -> ("error out"=w1441:errorcluster, "VISA ressource out"=w1440:refnum<visa-resource-name>)  [unwired: 3 in, 2 out]
                  }
                }
              }
              event "Pos 4 (Steps)": Value Change {
                w1471 = u16 4 items=["none", "1", "2", "3", "4", "all"] ("Motor")
                n614 = event-data() -> ("OldVal"=w1475:i32, "NewVal"=w1476:i32)  [unwired: 1 in, 4 out]
                n615 = Subtract(x=w1476, y=w1475) -> (x-y=w1470:i32)
                n616 = Number To Decimal String(number=w1470) -> (decimal integer string=w1474:string)  [unwired: 1 in]
                n617 = call "Read_only_Manipulator.vi"("Motor"=w1471, "error in (no error)"=w1468, "Value"=w1474, "Command"=Set_Parameter."Move Relative (MR)", "VISA resource name"=w1469) -> ("error out"=w1473:errorcluster, "VISA ressource out"=w1472:refnum<visa-resource-name>)  [unwired: 3 in, 2 out]
              }
              event "Pos 1": Value Change {
                w1481 = u16 1 items=["none", "1", "2", "3", "4", "all"] ("Motor")
                n618 = event-data() -> ("OldVal"=w1492:dbl, "NewVal"=w1491:dbl)  [unwired: 1 in, 4 out]
                n619 = Subtract(x=w1491, y=w1492) -> (x-y=w1485:dbl)
                n620 = property on="Pos Unit" class="Ring (strict)"() -> ("Value"=w1480:T8)  [unwired: 2 in, 2 out]
                n621 = case shown="3" w1480 {
                  tunnel: [Unit_Control."Microsteps [TMC]" ("Output Unit") Unit_Control."Micron" ("Output Unit") Unit_Control."Millimeter" ("Output Unit") Unit_Control."Centimeter" ("Output Unit") Unit_Control."Inches" ("Output Unit")] -> w1484
                  tunnel: [Unit_Control."Microsteps [TMC]" ("Output Unit") Unit_Control."Microsteps [TMC]" ("Output Unit") Unit_Control."Microsteps [TMC]" ("Output Unit") Unit_Control."Microsteps [TMC]" ("Output Unit") Unit_Control."Microsteps [TMC]" ("Output Unit")] -> w1483
                  frame 0, Default {
                  }
                  frame 1 {
                  }
                  frame 2 {
                  }
                  frame 3 {
                  }
                  frame 4 {
                  }
                }
                n622 = call "Conversion_Simple.vi"("Motor"=w1481, "Output Unit"=w1483, "Input Unit"=w1484, "Input"=w1485) -> ("Output"=w1487:dbl)  [unwired: 6 in, 1 out]
                n623 = To Long Integer(number=w1487) -> (32bit integer=w1482:i32)
                n624 = Number To Decimal String(number=w1482) -> (decimal integer string=w1486:string)  [unwired: 1 in]
                n625 = call "Read_only_Manipulator.vi"("Motor"=w1481, "error in (no error)"=w1479, "Value"=w1486, "Command"=Set_Parameter."Move Relative (MR)", "VISA resource name"=w1478) -> ("error out"=w1489:errorcluster, "VISA ressource out"=w1490:refnum<visa-resource-name>)  [unwired: 3 in, 2 out]
              }
              event "Pos 2": Value Change {
                w1507 = u16 2 items=["none", "1", "2", "3", "4", "all"] ("Motor")
                n626 = event-data() -> ("OldVal"=w1517:dbl, "NewVal"=w1516:dbl)  [unwired: 1 in, 4 out]
                n627 = Subtract(x=w1516, y=w1517) -> (x-y=w1510:dbl)
                n628 = property on="Pos Unit" class="Ring (strict)"() -> ("Value"=w1505:T8)  [unwired: 2 in, 2 out]
                n629 = case shown="0, Default" w1505 {
                  tunnel: [Unit_Control."Microsteps [TMC]" ("Output Unit") Unit_Control."Micron" ("Output Unit") Unit_Control."Millimeter" ("Output Unit") Unit_Control."Centimeter" ("Output Unit") Unit_Control."Inches" ("Output Unit")] -> w1509
                  tunnel: [Unit_Control."Microsteps [TMC]" ("Output Unit") Unit_Control."Microsteps [TMC]" ("Output Unit") Unit_Control."Microsteps [TMC]" ("Output Unit") Unit_Control."Microsteps [TMC]" ("Output Unit") Unit_Control."Microsteps [TMC]" ("Output Unit")] -> w1508
                  frame 0, Default {
                  }
                  frame 1 {
                  }
                  frame 2 {
                  }
                  frame 3 {
                  }
                  frame 4 {
                  }
                }
                n630 = call "Conversion_Simple.vi"("Motor"=w1507, "Output Unit"=w1508, "Input Unit"=w1509, "Input"=w1510) -> ("Output"=w1512:dbl)  [unwired: 6 in, 1 out]
                n631 = To Long Integer(number=w1512) -> (32bit integer=w1506:i32)
                n632 = Number To Decimal String(number=w1506) -> (decimal integer string=w1511:string)  [unwired: 1 in]
                n633 = call "Read_only_Manipulator.vi"("Motor"=w1507, "error in (no error)"=w1504, "Value"=w1511, "Command"=Set_Parameter."Move Relative (MR)", "VISA resource name"=w1503) -> ("error out"=w1514:errorcluster, "VISA ressource out"=w1515:refnum<visa-resource-name>)  [unwired: 3 in, 2 out]
              }
              event "Pos 3": Value Change {
                w1532 = u16 3 items=["none", "1", "2", "3", "4", "all"] ("Motor")
                n634 = event-data() -> ("OldVal"=w1543:dbl, "NewVal"=w1542:dbl)  [unwired: 1 in, 4 out]
                n635 = Subtract(x=w1542, y=w1543) -> (x-y=w1540:dbl)
                n636 = property on="Pos Unit" class="Ring (strict)"() -> ("Value"=w1537:T8)  [unwired: 2 in, 2 out]
                n637 = case shown="1" w1537 {
                  tunnel: [Unit_Control."Microsteps [TMC]" ("Output Unit") Unit_Control."Micron" ("Output Unit") Unit_Control."Millimeter" ("Output Unit") Unit_Control."Centimeter" ("Output Unit") Unit_Control."Inches" ("Output Unit")] -> w1539
                  tunnel: [Unit_Control."Microsteps [TMC]" ("Output Unit") Unit_Control."Microsteps [TMC]" ("Output Unit") Unit_Control."Microsteps [TMC]" ("Output Unit") Unit_Control."Microsteps [TMC]" ("Output Unit") Unit_Control."Microsteps [TMC]" ("Output Unit")] -> w1538
                  frame 0, Default {
                  }
                  frame 1 {
                  }
                  frame 2 {
                  }
                  frame 3 {
                  }
                  frame 4 {
                  }
                }
                n638 = call "Conversion_Simple.vi"("Motor"=w1532, "Output Unit"=w1538, "Input Unit"=w1539, "Input"=w1540) -> ("Output"=w1541:dbl)  [unwired: 6 in, 1 out]
                n639 = To Long Integer(number=w1541) -> (32bit integer=w1530:i32)
                n640 = property on="Z tilt comp" class="Bool (strict)"() -> ("Value"=w1533:bool)  [unwired: 2 in, 2 out]
                n641 = property on="Z tilt (degrees)" class="DigNum (strict)"() -> ("Value"=w1534:dbl)  [unwired: 2 in, 2 out]
                n642 = Number To Decimal String(number=w1530) -> (decimal integer string=w1531:string)  [unwired: 1 in]
                n643 = case shown="True" w1533 {
                  tunnel: w1528 -> [w1545 w1573]
                  tunnel: w1529 -> [w1544 w1574]
                  tunnel: [w1550 w1577] -> w1535
                  tunnel: [w1549 w1576] -> w1536
                  tunnel: w1531 -> [w1548 w1552]
                  tunnel: w1532 -> [w1546 w1583]
                  tunnel: w1530 -> [_ w1559]
                  tunnel: w1534 -> [_ w1579]
                  frame False {
                    n644 = call "Read_only_Manipulator.vi"("Motor"=w1546, "error in (no error)"=w1544, "Value"=w1548, "Command"=Set_Parameter."Move Relative (MR)", "VISA resource name"=w1545) -> ("error out"=w1550:errorcluster, "VISA ressource out"=w1549:refnum<visa-resource-name>)  [unwired: 3 in, 2 out]
                  }
                  frame True {
                    w1553 = 6.0
                    w1585 = Set_Parameter."Move Relative (MR)" ("Command")
                    w1566 = u16 2 items=["none", "1", "2", "3", "4", "all"] ("Motor")
                    # "This is the ratio of\nlength per step for\nmotors 3 and 2."
                    n645 = Negate(x=w1579) -> (-x=w1591:dbl)
                    n646 = Sign(1:w1559) -> (0:w1558:i32)
                    n647 = Sign(1:w1591) -> (0:w1590:dbl)
                    n648 = Multiply(x=w1590, y=w1558) -> (x*y=w1589:dbl)
                    n649 = call "Conversion_Simple.vi"("Output Unit"=Unit_Control."Rad", "Input Unit"=Unit_Control."Angle (Degrees)", "Input"=w1579) -> ("Output"=w1592:dbl)  [unwired: 7 in, 1 out]
                    n650 = To Long Integer(number=w1589) -> (32bit integer=w1588:i32)
                    n651 = Tangent(1:w1592) -> (0:w1578:dbl)
                    n652 = case shown="1" w1588 {
                      tunnel: ["-" "0" "+"] -> w1584
                      frame -1 {
                      }
                      frame 0, Default {
                      }
                      frame 1 {
                      }
                    }
                    n653 = Multiply(x=w1578, y=w1559) -> (x*y=w1564:dbl)
                    n654 = Multiply(x=w1578, y=15000.0) -> (x*y=w1562:dbl)
                    n655 = Multiply(x=w1553, y=w1562) -> (x*y=w1561:dbl)
                    n656 = Multiply(x=w1553, y=w1564) -> (x*y=w1563:dbl)
                    n657 = To Long Integer(number=w1561) -> (32bit integer=w1557:i32)
                    n658 = To Long Integer(number=w1563) -> (32bit integer=w1555:i32)
                    n659 = Absolute Value(x=w1557) -> (abs(x)=w1556:i32)
                    n660 = Absolute Value(x=w1555) -> (abs(x)=w1554:i32)
                    n661 = Number To Decimal String(number=w1556) -> (decimal integer string=w1571:string)  [unwired: 1 in]
                    n662 = Number To Decimal String(number=w1554) -> (decimal integer string=w1575:string)  [unwired: 1 in]
                    n663 = Concatenate Strings(w1584, w1575) -> (w1582:string)
                    n664 = call "Read_only_Manipulator.vi"("Motor"=w1566, "error in (no error)"=w1574, "Value"=w1571, "Command"=Set_Parameter."Velocity Maximum (VM)", "VISA resource name"=w1573) -> ("error out"=w1569:errorcluster, "VISA ressource out"=w1570:refnum<visa-resource-name>)  [unwired: 3 in, 2 out]
                    n665 = stacked-sequence {
                      tunnel: w1583 -> [w1598]
                      tunnel: w1582 -> [w1600]
                      tunnel: [w1598] -> w1581
                      tunnel: [w1600] -> w1580
                      tunnel: w1570 -> [w1597]
                      tunnel: w1569 -> [w1596]
                      tunnel: [w1596] -> w1568
                      tunnel: [w1597] -> w1567
                      tunnel: w1566 -> [w1599]
                      tunnel: [w1599] -> w1565
                      tunnel: w1552 -> [w1595]
                      tunnel: [w1595] -> w1551
                      frame #0 {
                      }
                    }
                    n666 = call "Read_only_Manipulator.vi"("Motor"=w1581, "error in (no error)"=w1568, "Value"=w1551, "Command"=w1585, "VISA resource name"=w1567) -> ("error out"=w1586:errorcluster, "VISA ressource out"=w1587:refnum<visa-resource-name>)  [unwired: 3 in, 2 out]
                    n667 = call "Read_only_Manipulator.vi"("Motor"=w1565, "error in (no error)"=w1586, "Value"=w1580, "Command"=w1585, "VISA resource name"=w1587) -> ("error out"=w1577:errorcluster, "VISA ressource out"=w1576:refnum<visa-resource-name>)  [unwired: 3 in, 2 out]
                  }
                }
              }
              event "Pos 4 [Angle]": Value Change {
                w1619 = u16 4 items=["none", "1", "2", "3", "4", "all"] ("Motor")
                n668 = event-data() -> ("OldVal"=w1628:dbl, "NewVal"=w1622:dbl)  [unwired: 1 in, 4 out]
                n669 = Subtract(x=w1622, y=w1628) -> (x-y=w1618:dbl)
                n670 = case shown="4" "Pos Unit" {
                  tunnel: [Unit_Control."Angle [TMC]" ("Output Unit") Unit_Control."Angle (Degrees)" ("Output Unit") Unit_Control."Angle (Degrees)" ("Output Unit") Unit_Control."Angle (Degrees)" ("Output Unit") Unit_Control."Angle (Degrees)" ("Output Unit")] -> w1620
                  tunnel: [Unit_Control."Angle [TMC]" ("Output Unit") Unit_Control."Angle [TMC]" ("Output Unit") Unit_Control."Angle [TMC]" ("Output Unit") Unit_Control."Angle [TMC]" ("Output Unit") Unit_Control."Angle [TMC]" ("Output Unit")] -> w1621
                  frame 0, Default {
                  }
                  frame 1 {
                  }
                  frame 2 {
                  }
                  frame 3 {
                  }
                  frame 4 {
                  }
                }
                n671 = call "Conversion_Simple.vi"("Motor"=w1619, "Output Unit"=w1621, "Input Unit"=w1620, "Input"=w1618) -> ("Output"=w1624:dbl)  [unwired: 6 in, 1 out]
                n672 = To Long Integer(number=w1624) -> (32bit integer=w1617:i32)
                n673 = Number To Decimal String(number=w1617) -> (decimal integer string=w1623:string)  [unwired: 1 in]
                n674 = call "Read_only_Manipulator.vi"("Motor"=w1619, "error in (no error)"=w1615, "Value"=w1623, "Command"=Set_Parameter."Move Relative (MR)", "VISA resource name"=w1616) -> ("error out"=w1626:errorcluster, "VISA ressource out"=w1627:refnum<visa-resource-name>)  [unwired: 3 in, 2 out]
              }
              event "Save Motor Positions": Value Change {
                n675 = event-data() -> ()  [unwired: 1 in, 6 out]
                n676 = case shown="12" "WAYPOINTS" {
                  tunnel: ["0" "1" "2" "3" "4" "5" "6" "7" "8" "9" "10" "11" "12" "13"] -> w1642
                  frame 0, Default {
                  }
                  frame 1 {
                  }
                  frame 2 {
                  }
                  frame 3 {
                  }
                  frame 4 {
                  }
                  frame 5 {
                  }
                  frame 6 {
                  }
                  frame 7 {
                  }
                  frame 8 {
                  }
                  frame 9 {
                  }
                  frame 10 {
                  }
                  frame 11 {
                  }
                  frame 12 {
                    n677 = global read "Pressure_Ch_1_2_Manipulator_Pos.vi" "Manipulator Pos"() -> (w1666:dbl[])
                    n678 = Index Array(array=w1666, index #1=0 ("index"), index #2=2 ("index")) -> (element #1=w1668:dbl, element #2=w1669:dbl)
                    n679 = Build Array(w1668, w1669) -> (→"corner 2":dbl[])
                  }
                  frame 13 {
                    n680 = global read "Pressure_Ch_1_2_Manipulator_Pos.vi" "Manipulator Pos"() -> (w1673:dbl[])
                    n681 = Index Array(array=w1673, index #1=0 ("index"), index #2=2 ("index")) -> (element #1=w1672:dbl, element #2=w1674:dbl)
                    n682 = Build Array(w1672, w1674) -> (→"corner 1":dbl[])
                  }
                }
                n683 = Concatenate Strings("Motor_Positions_" ("name or relative path"), w1642, ".txt" ("name or relative path")) -> (w1640:string)
                n684 = Build Path(base path=w1646, name or relative path=w1640) -> (appended path=w1645:path)
                n685 = call "save_motor_positions.vi"("Echo Mode"=w1644, "file path (use dialog)"=w1645, "error in"=w1650, "ComPort"=w1651) -> ("error out"=w1649:errorcluster, "Positions"=→"Saved Positions":string, "VISA ressource out"=w1648:refnum<visa-resource-name>)  [unwired: 5 in]
              }
              event "Go to Saved Position": Value Change {
                n686 = event-data() -> ()  [unwired: 1 in, 6 out]
                n687 = property on="WAYPOINTS" class="Ring (strict)"() -> ("Value"=w1682:u16)  [unwired: 2 in, 2 out]
                n688 = case shown="13" w1682 {
                  tunnel: ["0" "1" "2" "3" "4" "5" "6" "7" "8" "9" "10" "11" "12" "13"] -> w1680
                  frame 0, Default {
                  }
                  frame 1 {
                  }
                  frame 2 {
                  }
                  frame 3 {
                  }
                  frame 4 {
                  }
                  frame 5 {
                  }
                  frame 6 {
                  }
                  frame 7 {
                  }
                  frame 8 {
                  }
                  frame 9 {
                  }
                  frame 10 {
                  }
                  frame 11 {
                  }
                  frame 12 {
                  }
                  frame 13 {
                  }
                }
                n689 = Concatenate Strings("Motor_Positions_" ("name or relative path"), w1680, ".txt" ("name or relative path")) -> (w1678:string)
                n690 = Build Path(base path=w1688, name or relative path=w1678) -> (appended path=w1689:path)
                n691 = call "Go_to_Saved_Position.vi"("Echo Mode"=w1683, "file path (use dialog)"=w1689, "error in"=w1687, "ComPort"=w1686) -> ("error out"=w1685:errorcluster, "VISA ressource out"=w1684:refnum<visa-resource-name>)  [unwired: 5 in, 1 out]
              }
              event "Load Motor Positions": Value Change {
                # "Echo Mode not connected!\nStorage of Positions not\ndependent of Echo Mode."
                n692 = event-data() -> ()  [unwired: 1 in, 6 out]
                n693 = property on="WAYPOINTS" class="Ring (strict)"() -> ("Value"=w1711:u16)  [unwired: 2 in, 2 out]
                n694 = case shown="13" w1711 {
                  tunnel: ["0" "1" "2" "3" "4" "5" "6" "7" "8" "9" "10" "11" "12" "13"] -> w1709
                  frame 0, Default {
                  }
                  frame 1 {
                  }
                  frame 2 {
                  }
                  frame 3 {
                  }
                  frame 4 {
                  }
                  frame 5 {
                  }
                  frame 6 {
                  }
                  frame 7 {
                  }
                  frame 8 {
                  }
                  frame 9 {
                  }
                  frame 10 {
                  }
                  frame 11 {
                  }
                  frame 12 {
                  }
                  frame 13 {
                  }
                }
                n695 = Concatenate Strings("Motor_Positions_" ("name or relative path"), w1709, ".txt" ("name or relative path")) -> (w1707:string)
                n696 = Build Path(base path=w1713, name or relative path=w1707) -> (appended path=w1714:path)
                n697 = call "load_motor_positions.vi"("Echo Mode"=w1712, "file path (use dialog)"=w1714, "error in"=w1717, "ComPort"=w1718) -> ("error out"=w1705:errorcluster, "Loaded Positions"=→"Loaded Positions":string, "VISA ressource out"=w1716:refnum<visa-resource-name>)  [unwired: 5 in]
                n698 = property on="Load Motor Positions" class="Bool (strict)"(error in=w1705, "Value"=FALSE ("Load Motor Positions")) -> (error out=w1704:errorcluster)  [unwired: 1 in, 1 out]
              }
              event "Display Saved Position": Value Change {
                n699 = event-data() -> ()  [unwired: 1 in, 6 out]
                n700 = property on="WAYPOINTS" class="Ring (strict)"() -> ("Value"=w1742:u16)  [unwired: 2 in, 2 out]
                n701 = case shown="13" w1742 {
                  tunnel: ["0" "1" "2" "3" "4" "5" "6" "7" "8" "9" "10" "11" "12" "13"] -> w1740
                  frame 0, Default {
                  }
                  frame 1 {
                  }
                  frame 2 {
                  }
                  frame 3 {
                  }
                  frame 4 {
                  }
                  frame 5 {
                  }
                  frame 6 {
                  }
                  frame 7 {
                  }
                  frame 8 {
                  }
                  frame 9 {
                  }
                  frame 10 {
                  }
                  frame 11 {
                  }
                  frame 12 {
                  }
                  frame 13 {
                  }
                }
                n702 = Concatenate Strings("Motor_Positions_" ("name or relative path"), w1740, ".txt" ("name or relative path")) -> (w1736:string)
                n703 = Build Path(base path=w1737, name or relative path=w1736) -> (appended path=w1735:path)
                n704 = Open/Create/Replace File(file path (use dialog)=w1735, error in=w1734) -> (refnum out=w1746:refnum<file>, error out=w1745:errorcluster)  [unwired: 4 in, 1 out]
                n705 = Read from Text File(file (use dialog)=w1746, error in=w1745) -> (refnum out=w1744:refnum<file>, text=→"Display Saved Pos String":string, error out=w1743:errorcluster)  [unwired: 2 in, 1 out]
                n706 = Close File(refnum=w1744, error in=w1743) -> (error out=w1733:errorcluster)  [unwired: 1 out]
              }
              event "Set Angle Zero", "Set x,y,z Zero", "Define New Pos": Value Change {
                n707 = event-data() -> ()  [unwired: 1 in, 6 out]
                n708 = Two Button Dialog(message="Redefining position will render all saved waypoints useless.\nDo you want to continue?", 1:"Cancel" ("F button name (\"Cancel\")"), 2:"Yes" ("T button name (\"OK\")")) -> (T button?=w1767:bool)
                n709 = case shown="True" w1767 {
                  tunnel: "Set Angle Zero" -> [_ w1770]
                  tunnel: "Set x,y,z Zero" -> [_ w1769]
                  tunnel: "Define New Pos" -> [_ w1768]
                  frame False {
                  }
                  frame True {
                    n710 = case shown="True" w1770 {
                      selector: w1770 -> [_ w1773]
                      frame False {
                      }
                      frame True {
                        n711 = property on="Set Angle Zero Dummy" class="Bool (strict)"("Val(Sgnl)"=w1773) -> ()  [unwired: 2 in, 2 out]
                      }
                    }
                    n712 = case shown="True" w1769 {
                      selector: w1769 -> [_ w1772]
                      frame False {
                      }
                      frame True {
                        n713 = property on="Set x,y,z Zero Dummy" class="Bool (strict)"("Val(Sgnl)"=w1772) -> ()  [unwired: 2 in, 2 out]
                      }
                    }
                    n714 = case shown="True" w1768 {
                      selector: w1768 -> [_ w1771]
                      frame False {
                      }
                      frame True {
                        n715 = property on="Define New\nPos Dummy" class="Bool (strict)"("Val(Sgnl)"=w1771) -> ()  [unwired: 2 in, 2 out]
                      }
                    }
                  }
                }
              }
              event "Set x,y,z Zero Dummy", "Set Angle Zero Dummy": Value Change {
                n716 = event-data() -> ()  [unwired: 1 in, 6 out]
                n717 = case shown="True" "Set x,y,z Zero Dummy" {
                  tunnel: w1785 -> [w1800 w1815]
                  tunnel: w1784 -> [w1798 w1814]
                  tunnel: [w1800 w1806] -> w1783
                  tunnel: [w1798 w1802] -> w1782
                  tunnel: [w1799 w1805] -> w1781
                  tunnel: "0" ("Value") -> [w1799 w1805]
                  tunnel: Set_Parameter."Position (P)" ("Command") -> [w1797 w1801]
                  tunnel: [w1797 w1801] -> w1778
                  frame False {
                  }
                  frame True {
                    w1811 = u16 3 items=["none", "1", "2", "3", "4", "all"] ("Motor")
                    w1812 = u16 2 items=["none", "1", "2", "3", "4", "all"] ("Motor")
                    w1813 = u16 1 items=["none", "1", "2", "3", "4", "all"] ("Motor")
                    n718 = call "Read_and_Write_Manipulator.vi"("Motor"=w1813, "error in (no error)"=w1814, "Value"=w1805, "Command"=w1801, "VISA resource name"=w1815) -> ("error out"=w1809:errorcluster, "VISA ressource out"=w1810:refnum<visa-resource-name>)  [unwired: 2 in, 3 out]
                    n719 = call "Read_and_Write_Manipulator.vi"("Motor"=w1812, "error in (no error)"=w1809, "Value"=w1805, "Command"=w1801, "VISA resource name"=w1810) -> ("error out"=w1807:errorcluster, "VISA ressource out"=w1808:refnum<visa-resource-name>)  [unwired: 2 in, 3 out]
                    n720 = call "Read_and_Write_Manipulator.vi"("Motor"=w1811, "error in (no error)"=w1807, "Value"=w1805, "Command"=w1801, "VISA resource name"=w1808) -> ("error out"=w1803:errorcluster, "VISA ressource out"=w1806:refnum<visa-resource-name>)  [unwired: 2 in, 3 out]
                    n721 = property on="Set x,y,z Zero Dummy" class="Bool (strict)"(error in=w1803, "Value"=FALSE ("Set x,y,z Zero")) -> (error out=w1802:errorcluster)  [unwired: 1 in, 1 out]
                  }
                }
                n722 = case shown="True" "Set Angle Zero Dummy" {
                  tunnel: w1783 -> [w1787 w1795]
                  tunnel: w1782 -> [w1786 w1794]
                  tunnel: w1781 -> [_ w1793]
                  tunnel: w1778 -> [_ w1792]
                  tunnel: [w1787 w1791] -> w1777
                  tunnel: [w1786 w1788] -> w1776
                  frame False {
                  }
                  frame True {
                    w1796 = u16 4 items=["none", "1", "2", "3", "4", "all"] ("Motor")
                    n723 = call "Read_and_Write_Manipulator.vi"("Motor"=w1796, "error in (no error)"=w1794, "Value"=w1793, "Command"=w1792, "VISA resource name"=w1795) -> ("error out"=w1789:errorcluster, "VISA ressource out"=w1791:refnum<visa-resource-name>)  [unwired: 2 in, 3 out]
                    n724 = property on="Set Angle Zero Dummy" class="Bool (strict)"(error in=w1789, "Value"=FALSE ("Set Angle Zero")) -> (error out=w1788:errorcluster)  [unwired: 1 in, 1 out]
                  }
                }
              }
              event "Define New\nPos Dummy": Value Change {
                w1819 = Set_Parameter."Position (P)" ("Command")
                n725 = event-data() -> ()  [unwired: 1 in, 6 out]
                n726 = case shown="True" "M1 Change" {
                  tunnel: w1833 -> [w1889 w1900]
                  tunnel: w1832 -> [w1888 w1899]
                  tunnel: [w1889 w1898] -> w1829
                  tunnel: [w1888 w1897] -> w1828
                  tunnel: w1819 -> [_ w1896]
                  tunnel: "Unit of Move 3" -> [_ w1892]
                  frame False {
                  }
                  frame True {
                    w1895 = u16 1 items=["none", "1", "2", "3", "4", "all"] ("Motor")
                    n727 = case shown="0, Default" w1892 {
                      tunnel: [Unit_Control."Microsteps [TMC]" ("Output Unit") Unit_Control."Micron" ("Output Unit") Unit_Control."Millimeter" ("Output Unit") Unit_Control."Centimeter" ("Output Unit") Unit_Control."Inches" ("Output Unit")] -> w1891
                      frame 0, Default {
                      }
                      frame 1 {
                      }
                      frame 2 {
                      }
                      frame 3 {
                      }
                      frame 4 {
                      }
                    }
                    n728 = call "Conversion_Simple.vi"("Motor"=w1895, "Output Unit"=Unit_Control."Microsteps [TMC]", "Input Unit"=w1891, "Input"="Motor 1") -> ("Output"=w1893:string)  [unwired: 6 in, 1 out]
                    n729 = call "Read_and_Write_Manipulator.vi"("Motor"=w1895, "error in (no error)"=w1899, "Value"=w1893, "Command"=w1896, "VISA resource name"=w1900) -> ("error out"=w1897:errorcluster, "VISA ressource out"=w1898:refnum<visa-resource-name>)  [unwired: 2 in, 3 out]
                  }
                }
                n730 = case shown="True" "M2 Change" {
                  tunnel: w1829 -> [w1871 w1882]
                  tunnel: w1828 -> [w1870 w1881]
                  tunnel: [w1871 w1880] -> w1826
                  tunnel: [w1870 w1879] -> w1825
                  tunnel: w1819 -> [_ w1878]
                  tunnel: "Unit of Move 3" -> [_ w1875]
                  frame False {
                  }
                  frame True {
                    w1877 = u16 2 items=["none", "1", "2", "3", "4", "all"] ("Motor")
                    n731 = case shown="1" w1875 {
                      tunnel: [Unit_Control."Microsteps [TMC]" ("Output Unit") Unit_Control."Micron" ("Output Unit") Unit_Control."Millimeter" ("Output Unit") Unit_Control."Centimeter" ("Output Unit") Unit_Control."Inches" ("Output Unit")] -> w1874
                      frame 0, Default {
                      }
                      frame 1 {
                      }
                      frame 2 {
                      }
                      frame 3 {
                      }
                      frame 4 {
                      }
                    }
                    n732 = call "Conversion_Simple.vi"("Motor"=w1877, "Output Unit"=Unit_Control."Microsteps [TMC]", "Input Unit"=w1874, "Input"="Motor 2") -> ("Output"=w1876:string)  [unwired: 6 in, 1 out]
                    n733 = call "Read_and_Write_Manipulator.vi"("Motor"=w1877, "error in (no error)"=w1881, "Value"=w1876, "Command"=w1878, "VISA resource name"=w1882) -> ("error out"=w1879:errorcluster, "VISA ressource out"=w1880:refnum<visa-resource-name>)  [unwired: 2 in, 3 out]
                  }
                }
                n734 = case shown="True" "M3 Change" {
                  tunnel: w1826 -> [w1853 w1864]
                  tunnel: w1825 -> [w1852 w1863]
                  tunnel: [w1853 w1862] -> w1824
                  tunnel: [w1852 w1861] -> w1823
                  tunnel: w1819 -> [_ w1860]
                  tunnel: "Unit of Move 3" -> [_ w1857]
                  frame False {
                  }
                  frame True {
                    w1859 = u16 3 items=["none", "1", "2", "3", "4", "all"] ("Motor")
                    n735 = case shown="2" w1857 {
                      tunnel: [Unit_Control."Microsteps [TMC]" ("Output Unit") Unit_Control."Micron" ("Output Unit") Unit_Control."Millimeter" ("Output Unit") Unit_Control."Centimeter" ("Output Unit") Unit_Control."Inches" ("Output Unit")] -> w1856
                      frame 0, Default {
                      }
                      frame 1 {
                      }
                      frame 2 {
                      }
                      frame 3 {
                      }
                      frame 4 {
                      }
                    }
                    n736 = call "Conversion_Simple.vi"("Motor"=w1859, "Output Unit"=Unit_Control."Microsteps [TMC]", "Input Unit"=w1856, "Input"="Motor 3") -> ("Output"=w1858:string)  [unwired: 6 in, 1 out]
                    n737 = call "Read_and_Write_Manipulator.vi"("Motor"=w1859, "error in (no error)"=w1863, "Value"=w1858, "Command"=w1860, "VISA resource name"=w1864) -> ("error out"=w1861:errorcluster, "VISA ressource out"=w1862:refnum<visa-resource-name>)  [unwired: 2 in, 3 out]
                  }
                }
                n738 = case shown="True" "M4 Change" {
                  tunnel: w1824 -> [w1835 w1846]
                  tunnel: w1823 -> [w1834 w1845]
                  tunnel: [w1835 w1844] -> w1820
                  tunnel: [w1834 w1843] -> w1818
                  tunnel: w1819 -> [_ w1842]
                  tunnel: "Unit of Move 3" -> [_ w1839]
                  frame False {
                  }
                  frame True {
                    w1841 = u16 4 items=["none", "1", "2", "3", "4", "all"] ("Motor")
                    n739 = case shown="3" w1839 {
                      tunnel: [Unit_Control."Angle [TMC]" ("Output Unit") Unit_Control."Angle (Degrees)" ("Output Unit") Unit_Control."Angle (Degrees)" ("Output Unit") Unit_Control."Angle (Degrees)" ("Output Unit") Unit_Control."Angle (Degrees)" ("Output Unit")] -> w1838
                      frame 0, Default {
                      }
                      frame 1 {
                      }
                      frame 2 {
                      }
                      frame 3 {
                      }
                      frame 4 {
                      }
                    }
                    n740 = call "Conversion_Simple.vi"("Motor"=w1841, "Output Unit"=Unit_Control."Angle [TMC]", "Input Unit"=w1838, "Input"="Motor 4") -> ("Output"=w1840:string)  [unwired: 6 in, 1 out]
                    n741 = call "Read_and_Write_Manipulator.vi"("Motor"=w1841, "error in (no error)"=w1845, "Value"=w1840, "Command"=w1842, "VISA resource name"=w1846) -> ("error out"=w1843:errorcluster, "VISA ressource out"=w1844:refnum<visa-resource-name>)  [unwired: 2 in, 3 out]
                  }
                }
                n742 = property on="Define New\nPos Dummy" class="Bool (strict)"(error in=w1818, "Value"=FALSE ("Define New\nPos Dummy")) -> (error out=w1817:errorcluster)  [unwired: 1 in, 1 out]
              }
              event "Get Motor Positions": Value Change {
                w1921 = u16 4 items=["none", "1", "2", "3", "4", "all"] ("Motor In")
                w1922 = u16 3 items=["none", "1", "2", "3", "4", "all"] ("Motor In")
                w1927 = u16 2 items=["none", "1", "2", "3", "4", "all"] ("Motor In")
                w1930 = u16 1 items=["none", "1", "2", "3", "4", "all"] ("Motor In")
                n743 = event-data() -> ()  [unwired: 1 in, 6 out]
                n744 = property on="Pos Unit" class="Ring (strict)"() -> ("Value"=w1906:T8)  [unwired: 2 in, 2 out]
                n745 = case shown="2" w1906 {
                  tunnel: [Unit_Control."Microsteps [TMC]" ("Output Unit") Unit_Control."Micron" ("Output Unit") Unit_Control."Millimeter" ("Output Unit") Unit_Control."Centimeter" ("Output Unit") Unit_Control."Inches" ("Output Unit")] -> w1920
                  tunnel: [Unit_Control."Angle [TMC]" ("Output Unit") Unit_Control."Angle (Degrees)" ("Output Unit") Unit_Control."Angle (Degrees)" ("Output Unit") Unit_Control."Angle (Degrees)" ("Output Unit") Unit_Control."Angle (Degrees)" ("Output Unit")] -> w1908
                  frame 0, Default {
                  }
                  frame 1 {
                  }
                  frame 2 {
                  }
                  frame 3 {
                  }
                  frame 4 {
                  }
                }
                n746 = call "Get_Motor_Position.vi"("Echo Mode (2)"=w1907, "Motor In"=w1930, "error in (no error)"=w1931, "Output Unit"=w1920, "VISA resource name"=w1932) -> ("error out"=w1928:errorcluster, "Position (Steps)"=w1914:i32, "Position"=w1918:dbl, "VISA ressource out"=w1929:refnum<visa-resource-name>)  [unwired: 3 in]
                n747 = property on="Pos 1 (Steps)" class="DigNum (strict)"("Value"=w1914) -> ()  [unwired: 2 in, 2 out]
                n748 = property on="Pos 1" class="DigNum (strict)"("Value"=w1918) -> ()  [unwired: 2 in, 2 out]
                n749 = call "Get_Motor_Position.vi"("Echo Mode (2)"=w1907, "Motor In"=w1927, "error in (no error)"=w1928, "Output Unit"=w1920, "VISA resource name"=w1929) -> ("error out"=w1924:errorcluster, "Position (Steps)"=w1913:i32, "Position"=w1917:dbl, "VISA ressource out"=w1926:refnum<visa-resource-name>)  [unwired: 3 in]
                n750 = property on="Pos 2 (Steps)" class="DigNum (strict)"("Value"=w1913) -> ()  [unwired: 2 in, 2 out]
                n751 = property on="Pos 2" class="DigNum (strict)"("Value"=w1917) -> ()  [unwired: 2 in, 2 out]
                n752 = call "Get_Motor_Position.vi"("Echo Mode (2)"=w1907, "Motor In"=w1922, "error in (no error)"=w1924, "Output Unit"=w1920, "VISA resource name"=w1926) -> ("error out"=w1923:errorcluster, "Position (Steps)"=w1912:i32, "Position"=w1916:dbl, "VISA ressource out"=w1925:refnum<visa-resource-name>)  [unwired: 3 in]
                n753 = property on="Pos 3 (Steps)" class="DigNum (strict)"("Value"=w1912) -> ()  [unwired: 2 in, 2 out]
                n754 = property on="Pos 3" class="DigNum (strict)"("Value"=w1916) -> ()  [unwired: 2 in, 2 out]
                n755 = call "Get_Motor_Position.vi"("Echo Mode (2)"=w1907, "Motor In"=w1921, "error in (no error)"=w1923, "Output Unit"=w1908, "VISA resource name"=w1925) -> ("error out"=w1910:errorcluster, "Position (Steps)"=w1911:i32, "Position"=w1915:dbl, "VISA ressource out"=w1919:refnum<visa-resource-name>)  [unwired: 3 in]
                n756 = property on="Pos 4 (Steps)" class="DigNum (strict)"("Value"=w1911) -> ()  [unwired: 2 in, 2 out]
                n757 = stacked-sequence {
                  tunnel: w1910 -> [w1944]
                  tunnel: [w1944] -> w1909
                  frame #0 {
                    n758 = property on="Get Motor Positions" class="Bool (strict)"("Value"=FALSE ("Get Motor Positions")) -> ()  [unwired: 2 in, 2 out]
                  }
                }
                n759 = property on="Pos 4 [Angle]" class="DigNum (strict)"("Value"=w1915) -> ()  [unwired: 2 in, 2 out]
              }
              event Value Change {
                n760 = event-data() -> ("NewVal"=w1946:T8)  [unwired: 1 in, 5 out]
                n761 = local read "Sample\nScan"() -> (w1945:bool)
                n762 = case shown="True" w1945 {
                  tunnel: w1946 -> [w1949 _]
                  frame False {
                    n763 = property on="Unit of Move" class="Ring (strict)"("Value"=w1949) -> ()  [unwired: 2 in, 2 out]
                  }
                  frame True {
                  }
                }
                n764 = property on="Pos Unit" class="Ring (strict)"("Value"=w1946) -> ()  [unwired: 2 in, 2 out]
                n765 = property on="Unit of Move 3" class="Ring (strict)"("Value"=w1946) -> ()  [unwired: 2 in, 2 out]
                n766 = case shown="0, Default" w1946 {
                  tunnel: [w1950 1.0 1.0 1.0 1.0] -> w1948
                  tunnel: [w1950 0.01 ("Data Entry Limits:Increment") 0.1 ("Data Entry Limits:Increment") 1.0 ("Data Entry Limits:Increment") 10.0 ("Data Entry Limits:Increment")] -> w1947
                  frame 0, Default {
                    w1950 = 1.0
                  }
                  frame 1 {
                  }
                  frame 2 {
                  }
                  frame 3 {
                  }
                  frame 4 {
                  }
                }
                n767 = property on="Pos 1" class="DigNum (strict)"("Increment"=w1948) -> ()  [unwired: 2 in, 2 out]
                n768 = property on="Pos 2" class="DigNum (strict)"("Increment"=w1948) -> ()  [unwired: 2 in, 2 out]
                n769 = property on="Pos 3" class="DigNum (strict)"("Increment"=w1948) -> ()  [unwired: 2 in, 2 out]
                n770 = property on="Pos 4 [Angle]" class="DigNum (strict)"("Increment"=w1947) -> ()  [unwired: 2 in, 2 out]
              }
              event "Axis": Value Change {
                n771 = event-data() -> ()  [unwired: 1 in, 6 out]
                n772 = case shown="4" "Axis" {
                  tunnel: TRUE -> [w1965 w1966 w1968 w1971 w1972]
                  tunnel: FALSE -> [w1964 w1967 w1969 w1970 w1973]
                  tunnel: [w1965 w1966 w1968 w1970 w1973] -> w1960
                  tunnel: [w1964 w1967 w1969 w1971 w1972] -> w1959
                  frame 0, Default {
                  }
                  frame 1 {
                  }
                  frame 2 {
                  }
                  frame 3 {
                  }
                  frame 4 {
                  }
                }
                n773 = property on="Knife Edge Scan\n(1 Motor)" class="Bool"("Visible"=w1960) -> ()  [unwired: 2 in, 2 out]
                n774 = property on="Go to Cursor (1 Motor)" class="Bool"("Visible"=w1960) -> ()  [unwired: 2 in, 2 out]
                n775 = property on="Interrupt 1" class="Bool"("Visible"=w1960) -> ()  [unwired: 2 in, 2 out]
                n776 = property on="Knife Edge Scan\n(2 Motors)" class="Bool"("Visible"=w1959) -> ()  [unwired: 2 in, 2 out]
                n777 = property on="Go to Cursor (2 Motors)" class="Bool"("Visible"=w1959) -> ()  [unwired: 2 in, 2 out]
                n778 = property on="Interrupt 2" class="Bool"("Visible"=w1959) -> ()  [unwired: 2 in, 2 out]
              }
              event "Knife Edge Scan\n(1 Motor)": Value Change {
                w2018 = u32 100 ("y")
                n779 = event-data() -> ()  [unwired: 1 in, 6 out]
                n780 = stacked-sequence {
                  tunnel: w2034 -> [w2051 _]
                  tunnel: [w2051 _] -> w1997
                  tunnel: w2033 -> [w2050 _]
                  tunnel: [w2050 _] -> w2030
                  frame #0 {
                    w2049 = TRUE ("Wait")
                    n781 = local write "MM?"(w2049) -> ()
                    n782 = property on="Stop K" class="Bool (strict)"("Value"=w2049) -> ()  [unwired: 2 in, 2 out]
                    n783 = property on="Stop NI" class="Bool (strict)"("Value"=w2049) -> ()  [unwired: 2 in, 2 out]
                  }
                  frame #1 {
                    n784 = global read "Pressure_Ch_1_2_Manipulator_Pos.vi" "Manipulator Pos"() -> (w2053:dbl[])
                    n785 = local write "KE Positions"(w2053) -> ()
                    n786 = property on="angle" class="DigNum (strict)"("Value"=0.0 ("angle")) -> ()  [unwired: 2 in, 2 out]
                  }
                }
                n787 = property on="Current\nRange Ch1" class="Ring (strict)"() -> ("Value"=w1991:T3)  [unwired: 2 in, 2 out]
                n788 = property on="Current\nRange Ch2" class="Ring (strict)"() -> ("Value"=w1990:T3)  [unwired: 2 in, 2 out]
                n789 = case shown="False" "NI DAQ (t) / Keithley (f)" {
                  selector: "NI DAQ (t) / Keithley (f)" -> [w2040 w2047]
                  tunnel: w2001 -> [w2046 _]
                  tunnel: w2000 -> [w2045 w2048]
                  tunnel: [w2044 w2048] -> w1999
                  tunnel: w1998 -> [w2043 _]
                  tunnel: w1991 -> [w2042 _]
                  tunnel: w1990 -> [w2041 _]
                  tunnel: [w2040 w2047] -> w1977
                  frame False {
                    n790 = call "KE_scan_Init.vi"("GPIB (t) / RS-232 (f)"=w2043, "Current Range Ch 2"=w2041, "Current Range Ch 1"=w2042, "Cluster"=w2046, "Address in"=w2045) -> ("VISA resource name out"=w2044:refnum<visa-resource-name>)  [unwired: 5 in, 1 out]
                  }
                  frame True {
                  }
                }
                n791 = Divide(x="Scan Range", y="Nr. of Steps") -> (x/y=→"Resolution":dbl)
                n792 = property on="Axis" class="Ring (strict)"() -> ("Value"=w2031:u16)  [unwired: 2 in, 2 out]
                n793 = call "Knife_Edge_Scan_Parameters.vi"("VISA Ressource in"=w2032, "Axis"=w2031, "Scan Range (mum)"="Scan Range", "Nr. of Steps"="Nr. of Steps", "error in (no error)"=w1997, "Echo Mode"=w2030) -> ("VISA ressource out"=w2029:refnum<visa-resource-name>, "single steps 1"=w2013:i32[], "move time (ms)"=w2021:u32, "error out"=w1996:errorcluster)  [unwired: 1 in, 5 out]
                "single steps" <- w2013
                n794 = case shown="0, Default" w2031 {
                  tunnel: [w2096 w2097 w2098] -> w2003
                  frame 0, Default {
                    w2096 = u16 1 items=["none", "1", "2", "3", "4", "all"] ("Motor")
                  }
                  frame 1 {
                    w2097 = u16 2 items=["none", "1", "2", "3", "4", "all"] ("Motor")
                  }
                  frame 2 {
                    w2098 = u16 3 items=["none", "1", "2", "3", "4", "all"] ("Motor")
                  }
                }
                n795 = call "create_motor_scan_files.vi"("base path"=w1984) -> ("error out"=w1983:errorcluster, "Save Files Array"=w1985:path[], "Scan Number"=w1982:i32)  [unwired: 6 in, 2 out]
                n796 = local write "Scan Number"(w1982) -> ()
                n797 = local write "Save Files Array"(w1985) -> ()
                n798 = Array Size(array=w2013) -> (size(s)=w2028:i32)
                n799 = call "Get_Time_Stamp.vi"("error in"=w1996) -> ("error out"=w1995:errorcluster, "current time"=w2019:timestamp)  [unwired: 9 in]
                "Start\nTime" <- w2019
                n800 = call "KE_scan_time_calc.vi"("Nr. of Steps"="Nr. of Steps", "Start time"=w2019, "wait time (ms)"=w2018, "Integration Time per Step (ms)"="Integration Time per Step", "move time (ms)"=w2021) -> ("Estimated stop time"=→"Estimated\nStop Time":timestamp, "Scan Time"=w2014:dbl, "Start time out"=w2015:timestamp)  [unwired: 4 in]
                n801 = for {
                  N: w2028 -> [_]
                  tunnel: w2013 -> [w2082] mode=indexing
                  tunnel: w2029 -> [w2089]
                  tunnel: w1995 -> [w2086]
                  tunnel: Set_Parameter."Move Absolute (MA)" ("Command") -> [w2088]
                  tunnel: "Integration Time per Step" -> [w2083]
                  tunnel: w2003 -> [w2080]
                  tunnel: w2021 -> [w2073]
                  tunnel: w1999 -> [w2084]
                  tunnel: [w2060] -> w1981
                  shift-right: [w2066] -> w2027
                  shift-left: dbl[][] [] ("KE scan out") -> [w2068]
                  tunnel: "Nr. of Steps" -> [w2074]
                  tunnel: w1998 -> [w2070]
                  tunnel: [w2069] -> w1988
                  tunnel: w2018 -> [w2063]
                  tunnel: w2015 -> [_]
                  tunnel: w2014 -> [_]
                  tunnel: [w2061] -> w2012
                  tunnel: w1977 -> [w2056]
                  tunnel: w1983 -> [_]
                  tunnel: ["div I zero"] -> w1976
                  tunnel: ["Channel"] -> w1975
                  i -> [w2065]
                  stop <- "Interrupt 1" stop-if-true
                  n802 = Number To Decimal String(number=w2082) -> (decimal integer string=w2087:string)  [unwired: 1 in]
                  n803 = call "Read_only_Manipulator.vi"("Motor"=w2080, "error in (no error)"=w2086, "Value"=w2087, "Command"=w2088, "VISA resource name"=w2089) -> ("error out"=w2076:errorcluster, "VISA ressource out"=w2061:refnum<visa-resource-name>)  [unwired: 3 in, 2 out]
                  n804 = Equal?(x=0, y=w2065) -> (x = y?=w2075:bool)
                  n805 = case shown="False" w2075 {
                    tunnel: [w2091 w2095] -> w2077
                    tunnel: w2076 -> [w2091 w2095]
                    tunnel: w2074 -> [_ w2093]
                    tunnel: w2073 -> [w2090 w2092]
                    tunnel: [w2090 w2094] -> w2071
                    frame False {
                    }
                    frame True {
                      n806 = Multiply(x=w2092, y=w2093) -> (x*y=w2094:u32)
                    }
                  }
                  n807 = Add(x=w2071, y=w2063) -> (x+y=w2072:u32)
                  n808 = call "Conversion_Simple.vi"("Motor"=w2080, "Output Unit"=Unit_Control."Micron", "Input Unit"=Unit_Control."Microsteps [TMC]", "Input"=w2082) -> ("Output"=w2079:dbl)  [unwired: 6 in, 1 out]
                  n809 = call "wait_milliseconds.vi"("milliseconds to wait"=w2072, "error in"=w2077) -> ("error out"=w2085:errorcluster)  [unwired: 9 in]
                  n810 = call "Keithley_DAQ_for_Knife_Edge_Scan.vi"("GPIB (t) / RS-232 (f)"=w2070, "Keithley / NI DAQ Ch"="Channel", "error in (no error)"=w2085, "NI DAQ (t) / Keithley (f)"=w2056, "t_measure (ms) (1500)"=w2083, "Address in"=w2084) -> ("error out"=w2060:errorcluster, "Mean Value"=w2059:dbl, "Mean"=w2058:dbl[], "Address out"=w2069:refnum<visa-resource-name>)  [unwired: 2 out]
                  n811 = Build Array (concatenate)(w2079, w2059, w2058) -> (w2067:dbl[])
                  n812 = call "KE_scan_create_cluster_for_graph.vi"("Channel"="Channel", "new data point"=w2067, "NI DAQ (t) / Keithley (f)"=w2056, "iteration"=w2065, "div I zero"="div I zero", "KE scan in"=w2068) -> ("XY Graph Array"=→"XY Graph":cluster{dbl[], "subarray":dbl[]}[], "KE scan out"=w2066:dbl[][])  [unwired: 4 in]
                }
                n813 = call "get_middle_element_of_array.vi"("array in"=w2013) -> ("middle element of array (dbl)"=w2007:dbl, "middle element of array (string)"=w2010:string)  [unwired: 6 in, 3 out]
                n814 = call "Conversion_Simple.vi"("Motor"=w2003, "Output Unit"=Unit_Control."Micron", "Input Unit"=Unit_Control."Microsteps [TMC]", "Input"=w2007) -> ("Output"=w2004:dbl)  [unwired: 6 in, 1 out]
                n815 = call "KE_scan_Gaussian_Fit.vi"("NI DAQ (t) / Keithley (f)"=w1977, "GaussFit der (f, def) / raw (t)"="GaussFit der (f, def) / raw (t)", "Channel"=w1975, "div I zero"=w1976, "KE scan Array"=w2027) -> ("center"=→"Center":dbl, "FWHM"=→"FWHM":dbl, "KE scan Array OUT"=→"KE Scan Array":dbl[][], "residue"=→"Residue":dbl, "XY Graph Array"=w2011:cluster{dbl[], "Best Gaussian Fit":dbl[]}[])  [unwired: 2 out]
                n816 = property on="XY Graph" class="XYGraph (strict)"("Cursor.Cursor X"=w2004, "Value"=w2011) -> ()  [unwired: 2 in, 2 out]
                n817 = call "Play_Beep_Sound.vi"("error in"=w1981, "duration (s)"=0.5, "frequency (Hz)"=u32 5000) -> ("error out"=w1980:errorcluster)  [unwired: 8 in]
                n818 = call "Read_only_Manipulator.vi"("Motor"=w2003, "error in (no error)"=w1980, "Value"=w2010, "Command"=Set_Parameter."Move Absolute (MA)", "VISA resource name"=w2012) -> ("error out"=w1993:errorcluster, "VISA ressource out"=w2008:refnum<visa-resource-name>)  [unwired: 3 in, 2 out]
                n819 = property on="Save latest KE Scan" class="Bool (strict)"(error in=w1993, "Val(Sgnl)"=TRUE ("Value (Signaling)")) -> (error out=w1987:errorcluster)  [unwired: 1 in, 1 out]
                n820 = case shown="False" w1977 {
                  tunnel: w1988 -> [w2038 _]
                  tunnel: w1987 -> [w2037 w2039]
                  tunnel: [w2036 w2039] -> w1986
                  frame False {
                    n821 = VISA Close(VISA resource name=w2038, error in (no error)=w2037) -> (error out=w2036:errorcluster)
                  }
                  frame True {
                  }
                }
              }
              event "Knife Edge Scan\n(2 Motors)": Value Change {
                w2126 = Set_Parameter."Move Absolute (MA)" ("Command")
                w2141 = u32 100 ("y")
                n822 = event-data() -> ()  [unwired: 1 in, 6 out]
                n823 = stacked-sequence {
                  tunnel: w2162 -> [w2178 _]
                  tunnel: w2161 -> [w2179 _]
                  tunnel: [w2179 _] -> w2120
                  tunnel: [w2178 _] -> w2156
                  frame #0 {
                    w2177 = TRUE ("Wait")
                    n824 = local write "MM?"(w2177) -> ()
                    n825 = property on="Stop K" class="Bool (strict)"("Value"=w2177) -> ()  [unwired: 2 in, 2 out]
                    n826 = property on="Stop NI" class="Bool (strict)"("Value"=w2177) -> ()  [unwired: 2 in, 2 out]
                  }
                  frame #1 {
                    n827 = global read "Pressure_Ch_1_2_Manipulator_Pos.vi" "Manipulator Pos"() -> (→"KE Positions":dbl[])
                  }
                }
                n828 = property on="Current\nRange Ch2" class="Ring (strict)"() -> ("Value"=w2112:T3)  [unwired: 2 in, 2 out]
                n829 = property on="Current\nRange Ch1" class="Ring (strict)"() -> ("Value"=w2110:T3)  [unwired: 2 in, 2 out]
                n830 = property on="NI DAQ (t) / Keithley (f)" class="Bool (strict)"() -> ("Value"=w2111:bool)  [unwired: 2 in, 2 out]
                n831 = property on="Nr. of Steps" class="DigNum (strict)"() -> ("Value"=w2140:u32)  [unwired: 2 in, 2 out]
                n832 = property on="Scan Range" class="DigNum (strict)"() -> ("Value"=w2146:dbl)  [unwired: 2 in, 2 out]
                n833 = property on="Integration Time per Step" class="DigNum (strict)"() -> ("Value"=w2144:u32)  [unwired: 2 in, 2 out]
                n834 = property on="Z tilt (degrees)" class="DigNum (strict)"() -> ("Value"=w2155:dbl)  [unwired: 2 in, 2 out]
                n835 = case shown="False" w2111 {
                  selector: w2111 -> [w2168 w2175]
                  tunnel: w2124 -> [w2174 _]
                  tunnel: w2123 -> [w2173 w2176]
                  tunnel: [w2172 w2176] -> w2122
                  tunnel: w2121 -> [w2171 _]
                  tunnel: w2110 -> [w2170 _]
                  tunnel: w2112 -> [w2169 _]
                  tunnel: [w2168 w2175] -> w2101
                  frame False {
                    n836 = call "KE_scan_Init.vi"("GPIB (t) / RS-232 (f)"=w2171, "Current Range Ch 2"=w2169, "Current Range Ch 1"=w2170, "Cluster"=w2174, "Address in"=w2173) -> ("VISA resource name out"=w2172:refnum<visa-resource-name>)  [unwired: 5 in, 1 out]
                  }
                  frame True {
                  }
                }
                n837 = Divide(x=w2146, y=w2140) -> (x/y=w2145:dbl)
                n838 = property on="Resolution" class="DigNum (strict)"("Value"=w2145) -> ()  [unwired: 2 in, 2 out]
                n839 = property on="Axis" class="Ring (strict)"() -> ("Value"=w2159:u16)  [unwired: 2 in, 2 out]
                n840 = call "Knife_Edge_Scan_Parameters.vi"("VISA Ressource in"=w2158, "Axis"=w2159, "Scan Range (mum)"=w2146, "Nr. of Steps"=w2140, "Z tilt (angle)"=w2155, "error in (no error)"=w2120, "Echo Mode"=w2156) -> ("V_max 1/3 and 2"=→"V_max 1/3 and 2":i32[], "angle"=→"angle":dbl, "VISA ressource out"=w2157:refnum<visa-resource-name>, "micron steps"=w2138:dbl[], "single steps 1"=w2136:i32[], "single steps 2"=w2135:i32[], "Array Lengths equal?"=→"Array Lengths equal?":bool, "move time (ms)"=w2142:u32, "error out"=w2119:errorcluster)
                "single steps 1" <- w2136
                "single steps 2" <- w2135
                "micron steps" <- w2138
                n841 = case shown="3" w2159 {
                  tunnel: [w2228 w2229 w2230 w2232 w2234] -> w2130
                  tunnel: [_ _ _ w2231 w2233] -> w2129
                  frame 0, Default {
                    w2228 = u16 1 items=["none", "1", "2", "3", "4", "all"] ("Motor")
                  }
                  frame 1 {
                    w2229 = u16 2 items=["none", "1", "2", "3", "4", "all"] ("Motor")
                  }
                  frame 2 {
                    w2230 = u16 3 items=["none", "1", "2", "3", "4", "all"] ("Motor")
                  }
                  frame 3 {
                    w2231 = u16 2 items=["none", "1", "2", "3", "4", "all"] ("Motor")
                    w2232 = u16 1 items=["none", "1", "2", "3", "4", "all"] ("Motor")
                  }
                  frame 4 {
                    w2233 = u16 2 items=["none", "1", "2", "3", "4", "all"] ("Motor")
                    w2234 = u16 3 items=["none", "1", "2", "3", "4", "all"] ("Motor")
                  }
                }
                n842 = call "create_motor_scan_files.vi"("base path"=w2105) -> ("error out"=w2103:errorcluster, "Save Files Array"=w2104:path[], "Scan Number"=→"Scan Number":i32)  [unwired: 6 in, 2 out]
                n843 = local write "Save Files Array"(w2104) -> ()
                n844 = Array Size(array=w2136) -> (size(s)=w2160:i32)
                n845 = call "Get_Time_Stamp.vi"("error in"=w2119) -> ("error out"=w2118:errorcluster, "current time"=w2143:timestamp)  [unwired: 9 in]
                n846 = call "get_middle_element_of_array.vi"("array in"=w2135) -> ("middle element of array (string)"=w2127:string)  [unwired: 6 in, 4 out]
                n847 = call "get_middle_element_of_array.vi"("array in"=w2136) -> ("middle element of array (string)"=w2128:string)  [unwired: 6 in, 4 out]
                n848 = call "KE_scan_time_calc.vi"("Nr. of Steps"=w2140, "Start time"=w2143, "wait time (ms)"=w2141, "Integration Time per Step (ms)"=w2144, "move time (ms)"=w2142) -> ("Estimated stop time"=w2117:timestamp, "Scan Time"=w2139:dbl, "Start time out"=w2116:timestamp)  [unwired: 4 in]
                n849 = for {
                  N: w2160 -> [_]
                  tunnel: w2136 -> [w2221] mode=indexing
                  tunnel: w2157 -> [w2219]
                  tunnel: w2118 -> [w2217]
                  tunnel: Set_Parameter."Move Absolute (MA)" ("Command") -> [w2209]
                  tunnel: w2144 -> [w2214]
                  shift-right: [w2192] -> w2150
                  shift-left: dbl[][] [] ("KE scan out") -> [w2193]
                  tunnel: w2130 -> [w2220]
                  tunnel: w2142 -> [w2203]
                  tunnel: w2122 -> [w2215]
                  tunnel: w2135 -> [w2213] mode=indexing
                  tunnel: w2129 -> [w2210]
                  tunnel: [w2187] -> w2108
                  tunnel: w2138 -> [w2207] mode=indexing
                  tunnel: w2140 -> [w2200]
                  tunnel: w2121 -> [w2198]
                  tunnel: [w2197] -> w2106
                  tunnel: [w2191] -> w2134
                  tunnel: w2141 -> [w2190]
                  tunnel: w2139 -> [_]
                  tunnel: w2116 -> [_]
                  tunnel: w2101 -> [w2184]
                  tunnel: w2103 -> [_]
                  tunnel: [w2181] -> w2100
                  tunnel: [w2182] -> w2099
                  i -> [w2195]
                  stop <- "Interrupt 2" stop-if-true
                  # "improve\nX-axis !!!"
                  n850 = property on="Channel" class="DigNum (strict)"() -> ("Value"=w2181:i32)  [unwired: 2 in, 2 out]
                  n851 = Number To Decimal String(number=w2221) -> (decimal integer string=w2218:string)  [unwired: 1 in]
                  n852 = Number To Decimal String(number=w2213) -> (decimal integer string=w2208:string)  [unwired: 1 in]
                  n853 = call "Read_only_Manipulator.vi"("Motor"=w2220, "error in (no error)"=w2217, "Value"=w2218, "Command"=w2209, "VISA resource name"=w2219) -> ("error out"=w2211:errorcluster, "Transmitted String"=→"Transmitted 1/3":string, "VISA ressource out"=w2212:refnum<visa-resource-name>)  [unwired: 3 in, 1 out]
                  n854 = call "Read_only_Manipulator.vi"("Motor"=w2210, "error in (no error)"=w2211, "Value"=w2208, "Command"=w2209, "VISA resource name"=w2212) -> ("error out"=w2205:errorcluster, "Transmitted String"=→"Transmitted 2":string, "VISA ressource out"=w2191:refnum<visa-resource-name>)  [unwired: 3 in, 1 out]
                  n855 = Equal?(x=0, y=w2195) -> (x = y?=w2199:bool)
                  n856 = local read "div I zero"() -> (w2182:bool)
                  n857 = case shown="True" w2199 {
                    tunnel: w2205 -> [w2223 w2227]
                    tunnel: [w2223 w2227] -> w2204
                    tunnel: w2203 -> [w2222 w2225]
                    tunnel: [w2222 w2224] -> w2202
                    tunnel: w2200 -> [_ w2226]
                    frame False {
                    }
                    frame True {
                      n858 = Multiply(x=w2225, y=w2226) -> (x*y=w2224:u32)
                    }
                  }
                  n859 = Add(x=w2202, y=w2190) -> (x+y=w2206:u32)
                  n860 = call "wait_milliseconds.vi"("milliseconds to wait"=w2206, "error in"=w2204) -> ("error out"=w2216:errorcluster)  [unwired: 9 in]
                  n861 = call "Keithley_DAQ_for_Knife_Edge_Scan.vi"("GPIB (t) / RS-232 (f)"=w2198, "Keithley / NI DAQ Ch"=w2181, "error in (no error)"=w2216, "NI DAQ (t) / Keithley (f)"=w2184, "t_measure (ms) (1500)"=w2214, "Address in"=w2215) -> ("error out"=w2187:errorcluster, "Mean Value"=w2196:dbl, "Mean"=w2183:dbl[], "Address out"=w2197:refnum<visa-resource-name>)  [unwired: 2 out]
                  n862 = Build Array (concatenate)(w2207, w2196, w2183) -> (w2194:dbl[])
                  n863 = call "KE_scan_create_cluster_for_graph.vi"("Channel"=w2181, "new data point"=w2194, "NI DAQ (t) / Keithley (f)"=w2184, "iteration"=w2195, "div I zero"=w2182, "KE scan in"=w2193) -> ("XY Graph Array"=w2185:cluster{dbl[], "subarray":dbl[]}[], "KE scan out"=w2192:dbl[][])  [unwired: 4 in]
                  n864 = property on="XY Graph" class="XYGraph (strict)"("Value"=w2185) -> ()  [unwired: 2 in, 2 out]
                }
                n865 = call "get_middle_element_of_array.vi"("array in"=w2138) -> ("middle element of array (dbl)"=w2151:dbl)  [unwired: 6 in, 4 out]
                n866 = property on="Start\nTime" class="AbsTime (strict)"("Value"=w2116) -> ()  [unwired: 2 in, 2 out]
                n867 = property on="Estimated\nStop Time" class="AbsTime (strict)"("Value"=w2117) -> ()  [unwired: 2 in, 2 out]
                n868 = call "Read_only_Manipulator.vi"("Motor"=w2130, "error in (no error)"=w2108, "Value"=w2128, "Command"=w2126, "VISA resource name"=w2134) -> ("error out"=w2133:errorcluster, "VISA ressource out"=w2132:refnum<visa-resource-name>)  [unwired: 3 in, 2 out]
                n869 = call "Read_only_Manipulator.vi"("Motor"=w2129, "error in (no error)"=w2133, "Value"=w2127, "Command"=w2126, "VISA resource name"=w2132) -> ("error out"=w2114:errorcluster, "VISA ressource out"=w2131:refnum<visa-resource-name>)  [unwired: 3 in, 2 out]
                n870 = property on="Save latest KE Scan" class="Bool (strict)"(error in=w2114, "Val(Sgnl)"=TRUE ("Value (Signaling)")) -> (error out=w2107:errorcluster)  [unwired: 1 in, 1 out]
                n871 = call "KE_scan_Gaussian_Fit.vi"("NI DAQ (t) / Keithley (f)"=w2101, "Channel"=w2100, "div I zero"=w2099, "KE scan Array"=w2150) -> ("center"=w2147:dbl, "FWHM"=w2148:dbl, "KE scan Array OUT"=w2149:dbl[][], "residue"=w2115:dbl, "XY Graph Array"=w2137:cluster{dbl[], "Best Gaussian Fit":dbl[]}[])  [unwired: 1 in, 2 out]
                n872 = property on="XY Graph" class="XYGraph (strict)"("Cursor.Cursor X"=w2151, "Value"=w2137) -> ()  [unwired: 2 in, 2 out]
                n873 = property on="FWHM" class="DigNum (strict)"("Value"=w2148) -> ()  [unwired: 2 in, 2 out]
                n874 = property on="KE Scan Array" class="Arr (strict)"("Value"=w2149) -> ()  [unwired: 2 in, 2 out]
                n875 = property on="Center" class="DigNum (strict)"("Value"=w2147) -> ()  [unwired: 2 in, 2 out]
                n876 = property on="Residue" class="DigNum (strict)"("Value"=w2115) -> ()  [unwired: 2 in, 2 out]
                n877 = case shown="False" w2101 {
                  tunnel: [w2166 w2167] -> w2109
                  tunnel: w2107 -> [w2165 w2167]
                  tunnel: w2106 -> [w2164 _]
                  frame False {
                    n878 = VISA Close(VISA resource name=w2164, error in (no error)=w2165) -> (error out=w2166:errorcluster)
                  }
                  frame True {
                  }
                }
              }
              event "Save latest KE Scan": Value Change {
                w2236 = "\t"
                n879 = event-data() -> ()  [unwired: 1 in, 6 out]
                n880 = property on="Axis" class="Ring (strict)"() -> ("Value"=w2267:u16)  [unwired: 2 in, 2 out]
                n881 = property on="Integration Time per Step" class="DigNum (strict)"() -> ("Value"=w2265:u32)  [unwired: 2 in, 2 out]
                n882 = property on="FWHM" class="DigNum (strict)"() -> ("Value"=w2260:dbl)  [unwired: 2 in, 2 out]
                n883 = property on="Center" class="DigNum (strict)"() -> ("Value"=w2263:dbl)  [unwired: 2 in, 2 out]
                n884 = property on="Residue" class="DigNum (strict)"() -> ("Value"=w2262:dbl)  [unwired: 2 in, 2 out]
                n885 = property on="angle" class="DigNum (strict)"() -> ("Value"=w2261:dbl)  [unwired: 2 in, 2 out]
                n886 = case shown="4" w2267 {
                  tunnel: ["Detector" "X-Rays" "Vertical" "In-Plain" "Vertical (with tilt)"] -> w2266
                  frame 0, Default {
                  }
                  frame 1 {
                  }
                  frame 2 {
                  }
                  frame 3 {
                  }
                  frame 4 {
                  }
                }
                n887 = Number To Decimal String(number=w2265) -> (decimal integer string=w2264:string)  [unwired: 1 in]
                n888 = Number To Fractional String(number=w2260) -> (F-format string=w2259:string)  [unwired: 3 in]
                n889 = Number To Fractional String(number=w2263) -> (F-format string=w2258:string)  [unwired: 3 in]
                n890 = Number To Exponential String(number=w2262) -> (E-format string=w2257:string)  [unwired: 3 in]
                n891 = Number To Fractional String(number=w2261) -> (F-format string=w2256:string)  [unwired: 3 in]
                n892 = local read "KE Positions"() -> (w2244:dbl[])
                n893 = Index Array(array=w2244, index #1=0 ("index"), index #2=1 ("index"), index #3=2 ("index"), index #4=3 ("index")) -> (element #1=w2245:dbl, element #2=w2243:dbl, element #3=w2242:dbl, element #4=w2241:dbl)
                n894 = Number To Fractional String(number=w2245) -> (F-format string=w2240:string)  [unwired: 3 in]
                n895 = Number To Fractional String(number=w2243) -> (F-format string=w2239:string)  [unwired: 3 in]
                n896 = Number To Fractional String(number=w2242) -> (F-format string=w2238:string)  [unwired: 3 in]
                n897 = Number To Fractional String(number=w2241) -> (F-format string=w2237:string)  [unwired: 3 in]
                n898 = Concatenate Strings(w2266, w2236, w2264, w2236, w2259, w2236, w2258, w2236, w2257, w2236, w2256, w2236, w2240, w2236, w2239, w2236, w2238, w2236, w2237, w2236) -> (w2268:string)
                n899 = Index Array(array="Save Files Array", index=0) -> (element=w2276:path)
                n900 = Index Array(array="Save Files Array", index=1) -> (element=w2277:path)
                n901 = property on="KE Scan Array" class="Arr (strict)"() -> ("Value"=w2281:dbl[][])  [unwired: 2 in, 2 out]
                n902 = Open/Create/Replace File(file path (use dialog)=w2276, error in=w2251) -> (refnum out=w2275:refnum<file>, error out=w2273:errorcluster)  [unwired: 4 in, 1 out]
                n903 = Transpose 2D Array(2D array=w2281) -> (transposed array=w2280:dbl[][])
                n904 = Set File Position(refnum=w2275, from (0:start)=enum16{"start", "end", "current"}."end", error in=w2273) -> (refnum out=w2274:refnum<file>, error out=w2272:errorcluster)  [unwired: 1 in]
                n905 = call-poly <vilib>:"Write To Spreadsheet File.vi"("format (%.3f)"="%.4e", "2D data"=w2280, "file path (dialog if empty)"=w2277) -> ()  [unwired: 5 in, 1 out]
                n906 = Write to Text File(file (use dialog)=w2274, text=w2268, error in=w2272) -> (refnum out=w2270:refnum<file>, error out=w2271:errorcluster)  [unwired: 1 in, 1 out]
                n907 = Close File(refnum=w2270, error in=w2271) -> (error out=w2254:errorcluster)  [unwired: 1 out]
                n908 = property on="Save latest KE Scan" class="Bool (strict)"(error in=w2254, "Value"=FALSE ("Save latest KE Scan")) -> (error out=w2253:errorcluster)  [unwired: 1 in, 1 out]
                n909 = case shown="True" TRUE {
                  tunnel: w2253 -> [w2283 w2285]
                  tunnel: [w2283 w2284] -> w2252
                  frame False {
                  }
                  frame True {
                    n910 = property on="Reset V_max" class="Bool (strict)"(error in=w2285, "Val(Sgnl)"=TRUE ("Value (Signaling)")) -> (error out=w2284:errorcluster)  [unwired: 1 in, 1 out]
                  }
                }
              }
              event "Go to Cursor (1 Motor)": Value Change {
                n911 = event-data() -> ()  [unwired: 1 in, 6 out]
                n912 = property on="Axis" class="Ring (strict)"() -> ("Value"=w2299:u16)  [unwired: 2 in, 2 out]
                n913 = property on="XY Graph" class="XYGraph (strict)"() -> ("Cursor.Cursor X"=w2295:dbl)  [unwired: 2 in, 2 out]
                n914 = case shown="1" w2299 {
                  tunnel: [w2303 w2304 w2305] -> w2294
                  frame 0, Default {
                    w2303 = u16 1 items=["none", "1", "2", "3", "4", "all"] ("Motor")
                  }
                  frame 1 {
                    w2304 = u16 2 items=["none", "1", "2", "3", "4", "all"] ("Motor")
                  }
                  frame 2 {
                    w2305 = u16 3 items=["none", "1", "2", "3", "4", "all"] ("Motor")
                  }
                }
                n915 = call "Conversion_Simple.vi"("Motor"=w2294, "Output Unit"=Unit_Control."Microsteps [TMC]", "Input Unit"=Unit_Control."Micron", "Input"=w2295) -> ("Output"=w2296:string)  [unwired: 6 in, 1 out]
                n916 = call "Read_only_Manipulator.vi"("Motor"=w2294, "error in (no error)"=w2292, "Value"=w2296, "Command"=Set_Parameter."Move Absolute (MA)", "VISA resource name"=w2293) -> ("error out"=w2300:errorcluster, "VISA ressource out"=w2301:refnum<visa-resource-name>)  [unwired: 3 in, 2 out]
              }
              event "Go to Cursor (2 Motors)": Value Change {
                (unwired) 0 ("index")
                w2344 = Set_Parameter."Move Absolute (MA)" ("Command")
                n917 = event-data() -> ()  [unwired: 1 in, 6 out]
                n918 = property on="Axis" class="Ring (strict)"() -> ("Value"=w2343:u16)  [unwired: 2 in, 2 out]
                n919 = property on="XY Graph" class="XYGraph (strict)"() -> ("Cursor.Cursor X"=w2317:dbl)  [unwired: 2 in, 2 out]
                n920 = property on="micron steps" class="Arr (strict)"() -> ("Value"=w2319:dbl[])  [unwired: 2 in, 2 out]
                n921 = property on="single steps 1" class="Arr (strict)"() -> ("Value"=w2337:i32[])  [unwired: 2 in, 2 out]
                n922 = property on="single steps 2" class="Arr (strict)"() -> ("Value"=w2336:i32[])  [unwired: 2 in, 2 out]
                n923 = Reverse 1D Array(array=w2319) -> (reversed array=w2321:dbl[])
                n924 = Index Array(array=w2319) -> (element=w2318:dbl)  [unwired: 1 in]
                n925 = Reverse 1D Array(array=w2337) -> (reversed array=w2334:i32[])
                n926 = Index Array(array=w2337, index=0) -> (element=w2312:i32)
                n927 = Reverse 1D Array(array=w2336) -> (reversed array=w2335:i32[])
                n928 = Index Array(array=w2336, index=0) -> (element=w2325:i32)
                "Min Value X-Rays" <- w2325
                n929 = case shown="3" w2343 {
                  tunnel: [w2347 w2348 w2349 w2351 w2353] -> w2310
                  tunnel: [_ _ _ w2350 w2352] -> w2342
                  frame 0, Default {
                    w2347 = u16 1 items=["none", "1", "2", "3", "4", "all"] ("Motor")
                  }
                  frame 1 {
                    w2348 = u16 2 items=["none", "1", "2", "3", "4", "all"] ("Motor")
                  }
                  frame 2 {
                    w2349 = u16 3 items=["none", "1", "2", "3", "4", "all"] ("Motor")
                  }
                  frame 3 {
                    w2350 = u16 2 items=["none", "1", "2", "3", "4", "all"] ("Motor")
                    w2351 = u16 1 items=["none", "1", "2", "3", "4", "all"] ("Motor")
                  }
                  frame 4 {
                    w2352 = u16 2 items=["none", "1", "2", "3", "4", "all"] ("Motor")
                    w2353 = u16 1 items=["none", "1", "2", "3", "4", "all"] ("Motor")
                  }
                }
                n930 = Index Array(array=w2321, index=0) -> (element=w2322:dbl)
                n931 = Index Array(array=w2334, index=0) -> (element=w2309:i32)
                n932 = Index Array(array=w2335, index=0) -> (element=w2333:i32)
                n933 = Subtract(x=w2317, y=w2318) -> (x-y=w2323:dbl)
                n934 = Subtract(x=w2322, y=w2318) -> (x-y=w2324:dbl)
                n935 = Divide(x=w2323, y=w2324) -> (x/y=w2313:dbl)
                "Percentage Range Micron Pos" <- w2313
                n936 = Subtract(x=w2309, y=w2312) -> (x-y=w2314:i32)
                "Range M1/M3" <- w2314
                n937 = Subtract(x=w2333, y=w2325) -> (x-y=w2328:i32)
                "Range X-Rays" <- w2328
                n938 = Multiply(x=w2313, y=w2328) -> (x*y=w2329:dbl)
                n939 = Multiply(x=w2313, y=w2314) -> (x*y=w2315:dbl)
                n940 = To Long Integer(number=w2329) -> (32bit integer=w2327:i32)
                n941 = To Long Integer(number=w2315) -> (32bit integer=w2316:i32)
                n942 = Add(x=w2325, y=w2327) -> (x+y=w2326:i32)
                "New X-Ray Pos" <- w2326
                n943 = Add(x=w2312, y=w2316) -> (x+y=w2308:i32)
                "New M1/M3 Pos" <- w2308
                n944 = Number To Decimal String(number=w2308) -> (decimal integer string=w2311:string)  [unwired: 1 in]
                n945 = call "Read_only_Manipulator.vi"("Motor"=w2310, "error in (no error)"=w2306, "Value"=w2311, "Command"=w2344, "VISA resource name"=w2307) -> ("error out"=w2346:errorcluster, "VISA ressource out"=w2345:refnum<visa-resource-name>)  [unwired: 3 in, 2 out]
                n946 = Number To Decimal String(number=w2326) -> (decimal integer string=w2332:string)  [unwired: 1 in]
                n947 = call "Read_only_Manipulator.vi"("Motor"=w2342, "error in (no error)"=w2346, "Value"=w2332, "Command"=w2344, "VISA resource name"=w2345) -> ("error out"=w2330:errorcluster, "VISA ressource out"=w2331:refnum<visa-resource-name>)  [unwired: 3 in, 2 out]
              }
              event "Nr. of Steps", "Scan Range": Value Change {
                n948 = event-data() -> ()  [unwired: 1 in, 6 out]
                n949 = local read "Scan Range"() -> (w2356:dbl)
                n950 = local read "Nr. of Steps"() -> (w2355:u32)
                n951 = Divide(x=w2356, y=w2355) -> (x/y=w2354:dbl)
                n952 = local write "Resolution"(w2354) -> ()
              }
              event "Calc Scan Time": Value Change {
                n953 = event-data() -> ()  [unwired: 1 in, 6 out]
                n954 = local read "Speed [microns/s]"() -> (w2359:dbl)
                n955 = local read "Scan Mode"() -> (w2361:T7)
                n956 = local read "Line Spacing [microns]"() -> (w2360:dbl)
                n957 = local read "Z tilt (degrees)"() -> (w2357:dbl)
                n958 = call "Sample_Scan_Pause.vi"("waypoints path"=w2366, "Z tilt"=w2357, "Spacing [microns]"=w2360, "Long Side Speed [micron/s]"=w2359, "Scan Mode"=w2361, "VISA resource name"=w2358) -> ("Scan Time (hous:minutes:seconds)"=w2367:string)  [unwired: 1 in, 4 out]
                n959 = property on="Scan Time" class="Str"(error in=w2365, "Value"=w2367) -> (error out=w2364:errorcluster)  [unwired: 1 in, 1 out]
                n960 = property on="Calc Scan Time" class="Bool (strict)"(error in=w2364, "Value"=FALSE ("Calc Scan Time")) -> (error out=w2362:errorcluster)  [unwired: 1 in, 1 out]
              }
              event "Sample\nScan": Value Change {
                n961 = event-data() -> ()  [unwired: 1 in, 6 out]
                n962 = local read "Z tilt (x/z)"() -> (w2388:dbl)
                n963 = local read "Z tilt comp"() -> (w2384:bool)
                n964 = call "Sample_Scan_Pause_v2.vi"("Z tilt comp"=w2384, "Tilt x/z"=w2388, "Spacing [microns]"="Line Spacing [microns]", "Long Side Speed [micron/s]"="Speed [microns/s]", "Scan Mode"="Scan Mode", "waypoints path"=w2387) -> ("velocity cluster"=→"velocity cluster":T1, "Scan Time (hous:minutes:seconds)"=→"Scan Time":string, "Sample Scan Array"=w2389:i32[][], "Problem"=→"Scan\nProb?":bool, "Number of Points"=→"Number of Scan Steps":i32)  [unwired: 1 in]
                n965 = call "Sample_Scan_Move_to_first_Pos.vi"("use semaphore?"=FALSE, "error in"=w2371, "Sample Scan Array In"=w2389, "ComPort"=w2386) -> ("error out"=w2377:errorcluster, "At first Pos?"=→"At first Scan Pos?":bool, "Sample Scan Array Out"=→"Sample Scan Array Out":i32[][], "VISA ressource out"=w2382:refnum<visa-resource-name>)  [unwired: 3 in, 1 out]
                n966 = global write "Global_Stop_Scan.vi" "Stop Scan"(FALSE ("Stop Scan")) -> ()
                n967 = global write "Global_Next_Scan_Position.vi" "XAS(f) / XPS(t)"(FALSE ("XAS(f) / XPS(t)")) -> ()
                n968 = property on="Next Scan Step" class="Bool (strict)"(error in=w2377, "Val(Sgnl)"=TRUE ("Value (Signaling)")) -> (error out=w2376:errorcluster)  [unwired: 1 in, 1 out]
                "Current Scan Step" <- 0 ("Current Scan Steps")
              }
              event "Next Scan Step": Value Change {
                n969 = event-data() -> ()  [unwired: 1 in, 6 out]
                n970 = global read "Global_Stop_Scan.vi" "Stop Scan"() -> (w2391:bool)
                "Stop Scan GLOBAL" <- w2391
                n971 = case shown="False" w2391 {
                  tunnel: w2395 -> [w2410 w2437]
                  tunnel: [w2400 w2437] -> w2394
                  tunnel: [w2398 w2438] -> w2393
                  tunnel: w2392 -> [w2396 w2438]
                  frame False {
                    # "even (R=0) -> long side move\nodd  (R=1) -> spacing move"
                    n972 = local read "Scan Mode"() -> (w2409:T7)
                    n973 = local read "Current Scan Step"() -> (w2407:i32)
                    n974 = local read "Sample Scan Array Out"() -> (w2406:i32[][])
                    n975 = local read "velocity cluster"() -> (w2408:T1)
                    n976 = Increment(x=w2407) -> (x+1=w2411:i32)
                    n977 = Quotient & Remainder(x=w2407, y=2) -> (x-y*floor(x/y)=w2414:i32)  [unwired: 1 out]
                    n978 = Number To Boolean Array(number=w2414) -> (Boolean array=w2415:bool[])
                    n979 = local write "Current Scan Step"(w2411) -> ()
                    n980 = Index Array(array=w2406, index (row)=w2407) -> (element=w2405:i32[])  [unwired: 1 in]
                    n981 = Index Array(array=w2415, index=0) -> (element=w2404:bool)
                    n982 = call "Sample_Scan_Pause_Exe.vi"("waiting time (ms)"=u32 25, "Spacing (t) / Long Side (f)"=w2404, "Scan Mode"=w2409, "error in"=w2396, "velocity cluster"=w2408, "Position Array"=w2405, "VISA resource name"=w2410) -> ("error out"=w2399:errorcluster, "Position Array out"=w2401:i32[], "VISA ressource out"=w2400:refnum<visa-resource-name>, "Move Motor"=w2402:u16)  [unwired: 1 out]
                    n983 = global write "Global_Next_Scan_Position.vi" "Next Scan Pos"(w2401) -> ()
                    n984 = global write "Global_Next_Scan_Position.vi" "MM Scan"(w2402) -> ()
                    n985 = case shown="True" "Last Scan Step?" {
                      tunnel: w2409 -> [_ w2418]
                      frame False {
                      }
                      frame True {
                        w2419 = u16 0 items=["none", "1", "2", "3", "4", "all"] ("Motor 6")
                        # "Scan Once OR\nStop Scan = true"
                        n986 = case shown="True" "Scan Type" {
                          tunnel: w2418 -> [w2430 w2432]
                          tunnel: [w2430 w2431] -> w2417
                          frame False {
                          }
                          frame True {
                            n987 = case shown="3" w2432 {
                              tunnel: [w2433 w2434 w2435 w2436] -> w2431
                              frame 0, Default {
                                w2433 = T7 2 items=["Mode 1", "Mode 2", "Reversed 1", "Reversed 2"] ("Scan Mode 2")
                              }
                              frame 1 {
                                w2434 = T7 3 items=["Mode 1", "Mode 2", "Reversed 1", "Reversed 2"] ("Scan Mode 2")
                              }
                              frame 2 {
                                w2435 = T7 0 items=["Mode 1", "Mode 2", "Reversed 1", "Reversed 2"] ("Scan Mode 2")
                              }
                              frame 3 {
                                w2436 = T7 1 items=["Mode 1", "Mode 2", "Reversed 1", "Reversed 2"] ("Scan Mode 2")
                              }
                            }
                          }
                        }
                        n988 = global read "Global_Stop_Scan.vi" "Stop Scan"() -> (w2422:bool)
                        n989 = Not(x=w2422) -> (.not. x?=w2424:bool)
                        n990 = And(x="Scan Type", y=w2424) -> (x .and. y?=w2423:bool)
                        n991 = global write "Global_Next_Scan_Position.vi" "MM Scan"(w2419) -> ()
                        n992 = case shown="False" w2423 {
                          selector: w2423 -> [w2427 w2428]
                          tunnel: w2417 -> [_ w2429]
                          frame False {
                            n993 = property on="Sample\nScan" class="Bool (strict)"("Value"=w2427) -> ()  [unwired: 2 in, 2 out]
                            n994 = global write "Global_Stop_Scan.vi" "Stop Scan"(FALSE ("Stop Scan")) -> ()
                            n995 = property on="Reset V_max" class="Bool (strict)"("Val(Sgnl)"=TRUE ("Value (Signaling)")) -> ()  [unwired: 2 in, 2 out]
                          }
                          frame True {
                            n996 = global write "Global_Next_Scan_Position.vi" "verfluchter Kackdreck"(w2428) -> ()
                            n997 = property on="Scan Mode" class="Ring (strict)"("Value"=w2429) -> ()  [unwired: 2 in, 2 out]
                          }
                        }
                        n998 = property on="Stop Scan (2D)" class="Bool (strict)"("Value"=FALSE) -> ()  [unwired: 2 in, 2 out]
                      }
                    }
                    n999 = disable-structure shown="Disabled" {
                      frame Disabled {
                        n1000 = local read "Number of Scan Steps"() -> ()  [unwired: 1 out]
                        n1001 = local read "Paused?"() -> ()  [unwired: 1 out]
                      }
                      frame Enabled {
                      }
                    }
                    n1002 = property on="Next Scan Step" class="Bool (strict)"(error in=w2399, "Value"=FALSE ("Next Scan Step")) -> (error out=w2398:errorcluster)  [unwired: 1 in, 1 out]
                  }
                  frame True {
                  }
                }
              }
              event "pause scan": Value Change {
                n1003 = event-data() -> ()  [unwired: 1 in, 6 out]
                n1004 = local read "Sample\nScan"() -> (w2441:bool)
                n1005 = case shown="True" "pause scan" {
                  selector: "pause scan" -> [w2444 _]
                  tunnel: w2442 -> [w2446 _]
                  tunnel: w2441 -> [w2445 w2453]
                  tunnel: w2440 -> [_ w2452]
                  tunnel: w2439 -> [_ w2451]
                  frame False {
                    # "Resume Scan"
                    n1006 = case shown="True" w2445 {
                      selector: w2445 -> [_ w2449]
                      tunnel: w2446 -> [_ _]
                      tunnel: w2444 -> [_ w2450]
                      frame False {
                      }
                      frame True {
                        n1007 = local read "Current Scan Step"() -> (w2447:i32)
                        n1008 = property on="Paused?" class="Bool (strict)"("Visible"=w2450) -> ()  [unwired: 2 in, 2 out]
                        n1009 = property on="Next Scan Step" class="Bool (strict)"("Val(Sgnl)"=w2449) -> ()  [unwired: 2 in, 2 out]
                        n1010 = Decrement(x=w2447) -> (x-1=w2448:i32)
                        n1011 = local write "Current Scan Step"(w2448) -> ()
                      }
                    }
                  }
                  frame True {
                    # "Pause Scan"
                    n1012 = case shown="True" w2453 {
                      selector: w2453 -> [_ w2456]
                      tunnel: w2452 -> [_ w2455]
                      tunnel: w2451 -> [_ w2454]
                      frame False {
                      }
                      frame True {
                        n1013 = stacked-sequence {
                          tunnel: w2456 -> [w2457 _]
                          tunnel: w2455 -> [_ w2458]
                          tunnel: w2454 -> [_ _]
                          frame #0 {
                            n1014 = property on="Paused?" class="Bool (strict)"("Visible"=w2457) -> ()  [unwired: 2 in, 2 out]
                            "Paused?" <- w2457
                          }
                          frame #1 {
                            w2459 = u16 5 items=["none", "1", "2", "3", "4", "all"] ("Motor")
                            n1015 = call "Read_only_Manipulator.vi"("Motor"=w2459, "Value"="0", "Command"=Set_Parameter."Slew (SL)", "VISA resource name"=w2458) -> ()  [unwired: 4 in, 4 out]
                          }
                        }
                      }
                    }
                  }
                }
              }
              event "Stop Scan (2D)": Value Change {
                # "merge with XPS scan?"
                n1016 = event-data() -> ()  [unwired: 1 in, 6 out]
                n1017 = local read "Sample\nScan"() -> (w2466:bool)
                n1018 = And(x="Stop Scan (2D)", y=w2466) -> (x .and. y?=w2464:bool)
                n1019 = case shown="True" w2464 {
                  selector: w2464 -> [_ w2469]
                  tunnel: [FALSE FALSE] -> w2463
                  tunnel: w2462 -> [_ _]
                  frame False {
                  }
                  frame True {
                    n1020 = global write "Global_Stop_Scan.vi" "Stop Scan"(w2469) -> ()
                  }
                }
                n1021 = local write "Stop Scan (2D)"(w2463) -> ()
              }
              event "Move Time Test": Value Change {
                n1022 = event-data() -> ()  [unwired: 1 in, 6 out]
                n1023 = Number To Decimal String(number="steps 2") -> (decimal integer string=w2479:string)  [unwired: 1 in]
                n1024 = call "calc_movement_time.vi"("waiting time end (0)"=u32 50, "Echo Mode"=w2476, "Motor"="Motor 5", "error in (no error)"=w2478, "steps"="steps 2", "VISA ressource in"=w2477) -> ("error out"=w2481:errorcluster, "move time (ms)"=w2473:u32, "VISA ressource out"=w2482:refnum<visa-resource-name>)  [unwired: 2 in, 1 out]
                "move time (ms)" <- w2473
                n1025 = call "Read_only_Manipulator.vi"("Motor"="Motor 5", "error in (no error)"=w2481, "Value"=w2479, "Command"=Set_Parameter."Move Relative (MR)", "VISA resource name"=w2482) -> ("error out"=w2484:errorcluster, "VISA ressource out"=w2472:refnum<visa-resource-name>)  [unwired: 3 in, 2 out]
                n1026 = case shown="True" TRUE {
                  tunnel: w2484 -> [w2487 w2497]
                  tunnel: [w2487 w2490] -> w2474
                  tunnel: w2473 -> [_ w2489]
                  tunnel: w2472 -> [w2486 w2488]
                  tunnel: [w2486 w2488] -> w2471
                  frame False {
                  }
                  frame True {
                    w2493 = TRUE
                    n1027 = stacked-sequence {
                      tunnel: w2497 -> [w2503]
                      tunnel: [w2503] -> w2494
                      tunnel: [w2502] -> w2495
                      frame #0 {
                        n1028 = Tick Count (ms)() -> (millisecond timer value=w2502:u32)
                      }
                    }
                    n1029 = Add(x=w2495, y=w2489) -> (x+y=w2496:u32)
                    n1030 = while {
                      tunnel: w2496 -> [w2520]
                      tunnel: w2495 -> [_]
                      shift-right: [w2504] -> _
                      shift-left: w2493 -> [w2509]
                      tunnel: w2494 -> [w2512]
                      tunnel: [w2512] -> w2491
                      shift-right: [w2511] -> _
                      shift-left: w2493 -> [w2510]
                      shift-right: [w2508] -> _
                      shift-left: u32 0 ("waiting time end (0)") -> [w2507]
                      stop <- "Loop Stop" stop-if-true
                      n1031 = Tick Count (ms)() -> (millisecond timer value=w2518:u32)
                      n1032 = Greater Or Equal?(x=w2518, y=w2520) -> (x >= y?=w2516:bool)
                      n1033 = And(x=w2516, y=w2509) -> (x .and. y?=w2515:bool)
                      n1034 = And(x="motor stopped", y=w2510) -> (x .and. y?=w2513:bool)
                      n1035 = case shown="True" w2515 {
                        tunnel: [TRUE FALSE] -> w2505
                        frame False {
                        }
                        frame True {
                          n1036 = Tick Count (ms)() -> (millisecond timer value=→"1":u32)
                        }
                      }
                      n1037 = case shown="True" w2513 {
                        tunnel: [TRUE FALSE] -> w2511
                        frame False {
                        }
                        frame True {
                          n1038 = Tick Count (ms)() -> (millisecond timer value=→"2":u32)
                        }
                      }
                      n1039 = Greater Than 0?(x=w2507) -> (x > 0?=w2506:bool)
                      n1040 = case shown="False" w2505 {
                        tunnel: w2507 -> [w2524 w2525]
                        tunnel: [w2523 w2525] -> w2508
                        frame False {
                          n1041 = Increment(x=w2524) -> (x+1=w2523:u32)
                        }
                        frame True {
                        }
                      }
                      n1042 = case shown="False" w2506 {
                        tunnel: w2505 -> [w2521 _]
                        tunnel: [w2521 FALSE] -> w2504
                        frame False {
                        }
                        frame True {
                        }
                      }
                      n1043 = Wait Until Next ms Multiple(millisecond multiple=u32 10) -> ()  [unwired: 1 out]
                    }
                    n1044 = stacked-sequence {
                      tunnel: w2491 -> [w2498]
                      tunnel: [w2498] -> w2490
                      frame #0 {
                        n1045 = property on="1" class="DigNum (strict)"() -> ("Value"=w2501:u32)  [unwired: 2 in, 2 out]
                        n1046 = property on="2" class="DigNum (strict)"() -> ("Value"=w2500:u32)  [unwired: 2 in, 2 out]
                        n1047 = Subtract(x=w2501, y=w2500) -> (x-y=→"delta time (ms)":u32)
                      }
                    }
                  }
                }
              }
              event "Reset V_max": Value Change {
                w2538 = u16 5 items=["none", "1", "2", "3", "4", "all"] ("Motor")
                n1048 = event-data() -> ()  [unwired: 1 in, 6 out]
                n1049 = call "Read_only_Manipulator.vi"("Motor"=w2538, "error in (no error)"=w2539, "Value"="15000", "Command"=Set_Parameter."Velocity Maximum (VM)", "VISA resource name"=w2540) -> ("error out"=w2533:errorcluster, "VISA ressource out"=w2535:refnum<visa-resource-name>)  [unwired: 3 in, 2 out]
                n1050 = property on="Reset V_max" class="Bool (strict)"(error in=w2533, "Value"=FALSE ("Reset V_max")) -> (error out=w2532:errorcluster)  [unwired: 1 in, 1 out]
              }
              event "Stop w Save Pos": Value Change {
                n1051 = event-data() -> ()  [unwired: 1 in, 6 out]
                n1052 = case shown="True" "Stop w Save Pos" {
                  tunnel: w2543 -> [w2544 w2548]
                  tunnel: [w2544 w2548] -> w2542
                  frame True {
                    n1053 = Two Button Dialog(message="Stopping the program without saving the current position may render all waypoints useless.\nDo you want to continue?", 1:"Cancel" ("F button name (\"Cancel\")"), 2:"Yes" ("T button name (\"OK\")")) -> ()  [unwired: 1 out]
                  }
                  frame False {
                  }
                }
              }
              event "Disp Axis Info": Value Change {
                n1054 = event-data() -> ()  [unwired: 1 in, 6 out]
                n1055 = property on="axis info pic" class="Pict"("Visible"="Disp Axis Info") -> ()  [unwired: 2 in, 2 out]
              }
              event "Disp Scan Info": Value Change {
                n1056 = event-data() -> ()  [unwired: 1 in, 6 out]
                n1057 = property on="scan info pic" class="Pict"("Visible"="Disp Scan Info") -> ()  [unwired: 2 in, 2 out]
              }
              event "Disp Waypoint Info": Value Change {
                n1058 = event-data() -> ()  [unwired: 1 in, 6 out]
                n1059 = property on="waypoint info pic" class="Pict"("Visible"="Disp Waypoint Info") -> ()  [unwired: 2 in, 2 out]
              }
              event "Idiotensicherung": Value Change {
                n1060 = event-data() -> ()  [unwired: 1 in, 6 out]
                n1061 = Not(x="Idiotensicherung") -> (.not. x?=w2554:bool)
                n1062 = property on="Set Angle Zero" class="Bool"("Visible"=w2554) -> ()  [unwired: 2 in, 2 out]
                n1063 = property on="Stop w Save Pos" class="Bool (strict)"("Visible"=w2554) -> ()  [unwired: 2 in, 2 out]
                n1064 = property on="Set x,y,z Zero" class="Bool"("Visible"=w2554) -> ()  [unwired: 2 in, 2 out]
                n1065 = property on="Define New Pos" class="Bool"("Visible"=w2554) -> ()  [unwired: 2 in, 2 out]
                n1066 = property on="Unit of Move 3" class="Ring (strict)"("Visible"=w2554) -> ()  [unwired: 2 in, 2 out]
                n1067 = property on="Motor 1" class="DigNum (strict)"("Visible"=w2554) -> ()  [unwired: 2 in, 2 out]
                n1068 = property on="Motor 2" class="DigNum (strict)"("Visible"=w2554) -> ()  [unwired: 2 in, 2 out]
                n1069 = property on="Motor 3" class="DigNum (strict)"("Visible"=w2554) -> ()  [unwired: 2 in, 2 out]
                n1070 = property on="Motor 4" class="DigNum (strict)"("Visible"=w2554) -> ()  [unwired: 2 in, 2 out]
                n1071 = property on="M1 Change" class="Bool (strict)"("Visible"=w2554) -> ()  [unwired: 2 in, 2 out]
                n1072 = property on="M2 Change" class="Bool (strict)"("Visible"=w2554) -> ()  [unwired: 2 in, 2 out]
                n1073 = property on="M3 Change" class="Bool (strict)"("Visible"=w2554) -> ()  [unwired: 2 in, 2 out]
                n1074 = property on="M4 Change" class="Bool (strict)"("Visible"=w2554) -> ()  [unwired: 2 in, 2 out]
                n1075 = case shown="False" "Idiotensicherung" {
                  tunnel: [u32 225 ("Button Size:Width") u32 345 ("Button Size:Width")] -> w2552
                  frame False {
                  }
                  frame True {
                  }
                }
                n1076 = property on="POV Map" class="Bool (strict)"("Visible"="Idiotensicherung") -> ()  [unwired: 2 in, 2 out]
                n1077 = property on="Reset Map" class="Bool"("Visible"="Idiotensicherung") -> ()  [unwired: 2 in, 2 out]
                n1078 = property on="Pos Graph" class="XYGraph (strict)"("Visible"="Idiotensicherung") -> ()  [unwired: 2 in, 2 out]
                n1079 = property on="Disp Path" class="Bool (strict)"("Visible"="Idiotensicherung") -> ()  [unwired: 2 in, 2 out]
                n1080 = property on="refresh (s)" class="DigNum (strict)"("Visible"="Idiotensicherung") -> ()  [unwired: 2 in, 2 out]
                n1081 = property on="emergency stop" class="Bool (strict)"("Width"=w2552) -> ()  [unwired: 2 in, 2 out]
              }
              event "Rel Steps": Value Change {
                n1082 = event-data() -> ("OldVal"=w2557:string, "NewVal"=w2561:string)  [unwired: 1 in, 4 out]
                n1083 = Scan From String(format string="%.6f", input string=w2561) -> (remaining string=w2560:string)  [unwired: 4 in, 2 out]
                n1084 = Equal?(x=w2560, y="") -> (x = y?=w2558:bool)
                n1085 = case shown="False" w2558 {
                  tunnel: w2557 -> [w2563 _]
                  frame False {
                    n1086 = local write "Rel Steps"(w2563) -> ()
                  }
                  frame True {
                  }
                }
              }
              event "Speed [microns/s]": Value Change {
                n1087 = event-data() -> ()  [unwired: 1 in, 6 out]
                n1088 = local read "Scan Mode"() -> (w2567:T7)
                n1089 = local read "Speed [microns/s]"() -> (w2566:dbl)
                n1090 = case shown="0, Default" w2567 {
                  tunnel: [1500.0 ("upper limit") 250.0 ("upper limit") 1500.0 ("upper limit") 250.0 ("upper limit")] -> w2570
                  frame 0, Default {
                  }
                  frame 1 {
                  }
                  frame 2 {
                  }
                  frame 3 {
                  }
                }
                n1091 = In Range and Coerce(upper limit=w2570, x=w2566, lower limit=0.0) -> (coerced(x)=w2565:dbl, In Range?=w2568:bool)
                n1092 = case shown="True" w2568 {
                  tunnel: w2565 -> [w2571 w2573]
                  tunnel: [w2571 w2575] -> w2564
                  frame False {
                    n1093 = One Button Dialog(message="Mode 1: maximum speed is 1500 microns/s (max. speed for up/down, in-plain movement will  be 250 microns/s)\nMode 2: maximum speed is 250 microns/s (up/down movement will be 250 microns/s) ") -> ()  [unwired: 1 in, 1 out]
                  }
                  frame True {
                    n1094 = In Range and Coerce(upper limit=1200.0, x=w2573, lower limit=800.0) -> (In Range?=w2574:bool)  [unwired: 1 out]
                    n1095 = case shown="True" w2574 {
                      frame False {
                      }
                      frame True {
                        n1096 = One Button Dialog(message="Currently values between 600 and 1400 not possible.") -> ()  [unwired: 1 in, 1 out]
                      }
                    }
                    n1097 = case shown="False" w2574 {
                      tunnel: [w2578 500.0 ("upper limit")] -> w2575
                      tunnel: w2573 -> [w2578 _]
                      frame False {
                      }
                      frame True {
                      }
                    }
                  }
                }
                n1098 = local write "Speed [microns/s]"(w2564) -> ()
              }
              event "Speed": Value Change {
                n1099 = event-data() -> ("OldVal"=w2586:dbl)  [unwired: 1 in, 5 out]
                n1100 = case shown="True" FALSE {
                  tunnel: "Speed" -> [_ w2590]
                  tunnel: w2586 -> [_ w2588]
                  frame False {
                  }
                  frame True {
                    n1101 = In Range and Coerce(upper limit=1200.0, x=w2590, lower limit=800.0) -> (In Range?=w2589:bool)  [unwired: 1 out]
                    n1102 = case shown="True" w2589 {
                      tunnel: w2588 -> [_ w2594]
                      frame False {
                      }
                      frame True {
                        n1103 = local write "Speed"(w2594) -> ()
                        n1104 = One Button Dialog(message="Currently values between 800 and 1200 not possible.") -> ()  [unwired: 1 in, 1 out]
                      }
                    }
                  }
                }
              }
              event "Def Speed": Value Change {
                n1105 = event-data() -> ()  [unwired: 1 in, 6 out]
                n1106 = property on="Speed" class="DigNum (strict)"("Visible"="Def Speed") -> ()  [unwired: 2 in, 2 out]
              }
              event "Z tilt (x/z)": Value Change {
                n1107 = event-data() -> ()  [unwired: 1 in, 6 out]
                n1108 = Inverse Tangent(1:"Z tilt (x/z)") -> (0:w2599:dbl)
                n1109 = call "Conversion_Simple.vi"("Output Unit"=Unit_Control."Angle (Degrees)", "Input Unit"=Unit_Control."Rad", "Input"=w2599) -> ("Output"=w2597:dbl)  [unwired: 7 in, 1 out]
                n1110 = Negate(x=w2597) -> (-x=w2596:dbl)
                n1111 = local write "Z tilt (degrees)"(w2596) -> ()
              }
              event "Z tilt (degrees)": Value Change {
                n1112 = event-data() -> ()  [unwired: 1 in, 6 out]
                n1113 = call "Conversion_Simple.vi"("Output Unit"=Unit_Control."Rad", "Input Unit"=Unit_Control."Angle (Degrees)", "Input"="Z tilt (degrees)") -> ("Output"=w2605:dbl)  [unwired: 7 in, 1 out]
                n1114 = Tangent(1:w2605) -> (0:w2603:dbl)
                n1115 = Negate(x=w2603) -> (-x=w2602:dbl)
                n1116 = local write "Z tilt (x/z)"(w2602) -> ()
              }
              event "Hor Angle Offset (degrees)": Value Change {
                n1117 = event-data() -> ()  [unwired: 1 in, 6 out]
                n1118 = call "Conversion_Simple.vi"("Output Unit"=Unit_Control."Rad", "Input Unit"=Unit_Control."Angle (Degrees)", "Input"="Hor Angle Offset (degrees)") -> ("Output"=w2609:dbl)  [unwired: 7 in, 1 out]
                n1119 = Tangent(1:w2609) -> (0:w2608:dbl)
                n1120 = local write "Hor Angle Offset (rad) M2/M1"(w2608) -> ()
              }
              event "Hor Angle Offset (rad) M2/M1": Value Change {
                n1121 = event-data() -> ()  [unwired: 1 in, 6 out]
                n1122 = Inverse Tangent(1:"Hor Angle Offset (rad) M2/M1") -> (0:w2616:dbl)
                n1123 = call "Conversion_Simple.vi"("Output Unit"=Unit_Control."Angle (Degrees)", "Input Unit"=Unit_Control."Rad", "Input"=w2616) -> ("Output"=w2614:dbl)  [unwired: 7 in, 1 out]
                n1124 = Negate(x=w2614) -> (-x=w2613:dbl)
                n1125 = local write "Hor Angle Offset (degrees)"(w2613) -> ()
              }
              event "Move Pico": Value Change {
                n1126 = event-data() -> ()  [unwired: 1 in, 6 out]
                n1127 = Two Button Dialog(message="Moving the mirror can cause reflections and lead to blindness and potentially to death.\nBy clicking \"Move\" you state that you are aware of this fact and take full responsability for all your actions. ", 2:"Move" ("T button name (\"OK\")")) -> (T button?=w2621:bool)  [unwired: 1 in]
                n1128 = case shown="True" w2621 {
                  tunnel: w2624 -> [w2625 w2631]
                  tunnel: [w2625 w2630] -> w2623
                  tunnel: w2622 -> [_ w2629]
                  frame False {
                  }
                  frame True {
                    n1129 = call "Spatial_Overlap.vi"("error in"=w2631, "Steps"="Pico Steps", "Motor"="PicoMotor", "Resource Name"=w2629) -> ("error out"=w2626:errorcluster)  [unwired: 5 in, 2 out]
                    n1130 = flat-sequence {
                      tunnel: w2626 -> [w2637]
                      tunnel: [w2637] -> w2636
                      tunnel: [w2641] -> w2635
                      tunnel: w2636 -> [w2641]
                      tunnel: w2635 -> [w2643]
                      tunnel: [w2643] -> w2634
                      tunnel: w2634 -> [w2645]
                      tunnel: [w2645] -> w2633
                      tunnel: w2633 -> [w2647]
                      tunnel: [w2647] -> w2632
                      tunnel: [w2649] -> w2630
                      tunnel: w2632 -> [w2649]
                      frame #0 {
                        n1131 = Unbundle By Name(w2637) -> ("status"=w2638:bool)
                        n1132 = Not(x=w2638) -> (.not. x?=→"Pico Error":bool)
                      }
                      frame #1 {
                        n1133 = Wait (ms)(milliseconds to wait=u32 100) -> ()  [unwired: 1 out]
                      }
                      frame #2 {
                        n1134 = local write "Move Pico"(FALSE ("Move Pico")) -> ()
                      }
                      frame #3 {
                        n1135 = property on="Pico Error" class="Bool (strict)"("Visible"=TRUE) -> ()  [unwired: 2 in, 2 out]
                      }
                      frame #4 {
                        n1136 = Wait (ms)(milliseconds to wait=u32 500) -> ()  [unwired: 1 out]
                      }
                      frame #5 {
                        n1137 = property on="Pico Error" class="Bool (strict)"("Visible"=FALSE) -> ()  [unwired: 2 in, 2 out]
                      }
                    }
                  }
                }
              }
              event "Change Baud Rate": Value Change {
                w2654 = u16 5 items=["none", "1", "2", "3", "4", "all"] ("Motor")
                n1138 = event-data() -> ()  [unwired: 1 in, 6 out]
                n1139 = case shown="115200" "Baudrate" {
                  tunnel: ["96" "19" "38" "11"] -> w2655
                  frame 9600, Default {
                  }
                  frame 19200 {
                  }
                  frame 38400 {
                  }
                  frame 115200 {
                  }
                }
                n1140 = call "Read_only_Manipulator.vi"("waiting time (ms)"=u32 250, "Motor"=w2654, "error in (no error)"=w2658, "Value"=w2655, "Command"=Set_Parameter."Baud Rate (BD)", "VISA resource name"=w2659) -> ("error out"=w2652:errorcluster, "Transmitted String"=→"Transmitted String Baud Rate":string, "VISA ressource out"=w2651:refnum<visa-resource-name>)  [unwired: 2 in, 1 out]
                n1141 = property class="Instr"(reference=w2651, error in=w2652, "Baud"="Baudrate") -> (reference out=w2661:refnum<visa-resource-name>, error out=w2660:errorcluster)
              }
              event "stop": Value Change {
                n1142 = event-data() -> ()  [unwired: 1 in, 6 out]
                n1143 = property on="Stop w Save Pos" class="Bool (strict)"() -> ("Value"=w2677:bool)  [unwired: 2 in, 2 out]
                n1144 = case shown="False" w2677 {
                  tunnel: w2681 -> [w2688 w2691]
                  tunnel: w2680 -> [w2687 w2692]
                  tunnel: w2667 -> [w2686 _]
                  tunnel: [w2685 w2691] -> w2679
                  tunnel: [w2684 w2692] -> w2671
                  tunnel: w2678 -> [w2683 _]
                  frame False {
                    n1145 = Build Path(base path=w2686, name or relative path="Motor_Positions_0.txt") -> (appended path=w2689:path)
                    n1146 = call "save_motor_positions.vi"("Echo Mode"=w2683, "file path (use dialog)"=w2689, "error in"=w2687, "ComPort"=w2688) -> ("error out"=w2684:errorcluster, "VISA ressource out"=w2685:refnum<visa-resource-name>)  [unwired: 5 in, 1 out]
                  }
                  frame True {
                  }
                }
                n1147 = Build Path(base path=w2667, name or relative path="Notizen.txt") -> (appended path=w2666:path)
                n1148 = Open/Create/Replace File(file path (use dialog)=w2666, error in=w2671, operation (0:open)=T13."replace or create") -> (refnum out=w2676:refnum<file>, error out=w2675:errorcluster)  [unwired: 3 in, 1 out]
                n1149 = Write to Text File(file (use dialog)=w2676, text="Notizen", error in=w2675) -> (refnum out=w2674:refnum<file>, error out=w2673:errorcluster)  [unwired: 1 in, 1 out]
                n1150 = Close File(refnum=w2674, error in=w2673) -> (error out=w2670:errorcluster)  [unwired: 1 out]
              }
            }
            "ComPort out" <- w323
            "error out" <- w322
            n1151 = Wait Until Next ms Multiple(millisecond multiple=u32 250) -> ()  [unwired: 1 out]
            "Firmware Version" <- w319
          }
          n1152 = while {
            shift-right: [w88] -> _
            shift-left: dbl[][] [] -> [w97]
            shift-right: [w85] -> _
            shift-left: 0 ("counter") -> [w86]
            stop <- w98 stop-if-true
            w82 = TRUE ("Map M1(t)/M2(f)")
            n1153 = case shown="False" "Reset Map" {
              tunnel: w97 -> [w103 _]
              tunnel: [w103 dbl[][] []] -> w89
              frame False {
              }
              frame True {
              }
            }
            n1154 = Get Date/Time In Seconds() -> (seconds since 1Jan1904=w80:timestamp)
            n1155 = global read "Pressure_Ch_1_2_Manipulator_Pos.vi" "Manipulator Pos"() -> (w87:dbl[])
            n1156 = Get Date/Time String(seconds (now)=w80, want seconds? (F)=TRUE) -> (time string=→"current time":string)  [unwired: 1 in, 1 out]
            n1157 = call "Map_Pos_sub_VI.vi"("counter"=w86, "array"=w87, "M1(t)/M2(f)"=w82, "Array"=w89) -> ("counter out"=w85:i32, "appended array"=w88:dbl[][])  [unwired: 6 in]
            n1158 = local read "corner 1"() -> (w93:dbl[])
            n1159 = local read "corner 2"() -> (w92:dbl[])
            n1160 = call "Generate_Map.vi"("current position"=w87, "corner 2"=w92, "2D array"=w88, "corner 1"=w93, "POV"="POV Map", "Map M1(t)/M2(f)"=w82, "Display Corner Positions?"="Disp Path") -> ("Cluster Array Plot"=w90:cluster{dbl[], dbl[]}[], "POV"=w91:bool)  [unwired: 3 in]
            n1161 = stacked-sequence {
              tunnel: w91 -> [w101 _]
              tunnel: w90 -> [_ w102]
              frame #0 {
                n1162 = property on="Pos Graph" class="XYGraph (strict)"("XScale.Flipped"=w101, "YScale.Flipped"=w101) -> ()  [unwired: 2 in, 2 out]
              }
              frame #1 {
                "Pos Graph" <- w102
                "Pos Graph 2" <- w102
              }
            }
            n1163 = Multiply(x="refresh (s)", y=1000.0 ("millisecond timer value")) -> (x*y=w84:dbl)
            n1164 = local read "stop"() -> (w98:bool)
            n1165 = To Unsigned Long Integer(number=w84) -> (unsigned 32bit integer=w83:u32)
            n1166 = Wait Until Next ms Multiple(millisecond multiple=w83) -> ()  [unwired: 1 out]
          }
        }
        frame Error {
          n1167 = One Button Dialog(message="Connection Problem:\n1) Is the controller turned on?\n[USB connection needs to be unplugged when turning the controller on]\n2) Unplug and plug in USB\n3) Look up the available connections in the \"Device Manager\"\nand try them in the \"ComPort\" Input\n4) Restart Computer") -> ()  [unwired: 1 in, 1 out]
        }
      }
    }
    frame #2 {
      n1168 = property on="stop" class="Bool (strict)"("Value"=FALSE) -> ()  [unwired: 2 in, 2 out]
    }
  }
